vi "数据采集传输系统.vi"(8 "停止 2":bool) -> ()   [LabVIEW 2016]
uses:
  <vilib>/Averna/Notify Icon/NotifyIcon.llb/BalloonIcon.ctl
  <vilib>/Utility/miscctls.llb/LVPointTypeDef.ctl
  <vilib>/Utility/config.llb/Read Key (String).vi
  <vilib>/Utility/config.llb/Read Key (I32).vi
  <vilib>/Utility/config.llb/Read Key (Boolean).vi
  <vilib>/Utility/config.llb/Write Key (String).vi
  <vilib>/Utility/config.llb/Write Key (U32).vi
  <vilib>/Utility/config.llb/Write Key (I32).vi
  <vilib>/Utility/config.llb/Write Key (Boolean).vi
  <vilib>/Averna/Notify Icon/NotifyIcon.llb/GetSelectedItemEvent.vi
  <vilib>/Averna/Notify Icon/NotifyIcon.llb/SetVisible.vi
  <vilib>/Averna/Notify Icon/NotifyIcon.llb/SetMenuDefaultItem.vi
  <vilib>/Averna/Notify Icon/NotifyIcon.llb/SetTipText.vi
  <vilib>/Averna/Notify Icon/NotifyIcon.llb/NotifyIcon.lvclass
  <vilib>/Utility/config.llb/NI_LVConfig.lvlib
  data/FreeMem.dll
  <vilib>/ptbypt/NI_PtbyPt.lvlib
panel:
  in  "数据组合发送":bool
  in  "日志、参数发送":bool
  in  "2011发送":bool
  in  "判断数据反馈":bool
  in  "数据发送协议":enum16{"2005-212协议", "2017-212协议"}(ring)=enum."2017-212协议"
  in  "数据发送通道":enum16{"TCP", "VISA"}(ring)
  in  "baud rate":u32=9600 caption="波特率"
  in  "VISA resource name":refnum<visa-resource-name> caption="VISA资源名称"
  in  "查询质控数据起始时间":bool
  in  "返回主界面":bool
  out "零点核查索引起始时间":string
  out "跨度核查索引起始时间":string
  out "加标回收索引起始时间":string
  out "标样核查索引起始时间":string
  out "数据接收超时指示灯":bool
  in  "重发时间":T1(ring)
  in  "重发日期":T2(ring)
  in  "锁":bool
  in  "开机启动":bool
  in  "确定更改起始时间":bool
  in  "更改起始时间":bool
  in  "数据发送起始时间":timestamp format="%<%.3X\n%Y/%m/%d>T"
  in  "每周自动重发":bool=TRUE
  in  "确定":bool
  in  "返回":bool
  in  "PW":string
  in  "MN":string
  in  "PORT":string
  in  "IP":string
  in  "站点设备":string
  in  "站点名称":string
  out "设置超时时间/min":i32=1
  in  "实时数据发送时间间隔/min":u32=1
  out "空闲时间/s":string
  out "状态信息":T3={"1st Error to Convert "=63, "步骤 "=enum."打开连接", "元素"="实时数据", "TCP服务端掉线计数"=4, "TCP掉线时间节点"="2019/05/08 15:24:17"} {"1st Error to Convert" items=["无错误", "参数错误", "内存已满", "超出区域", "文件结束", "文件已打开", "一般文件IO错误", "未找到文件", "文件权限错误", "磁盘已满", "路径副本", "打开过多文件", "未启用", "未找到资源文件", "无法添加资源", "未找到资源", "未找到图像", "图像内存错误", "画笔不存在", "配置错误类型", "配置未找到解析段", "配置解析错误", "配置内存错误", "错误外部代码格式", "错误外部代码偏移量", "外部代码不存在", "空窗口", "销毁窗口错误", "空菜单", "打印已中止", "错误打印记录", "打印驱动程序错误", "打印时窗口错误", "打印时内存错误", "打印对话框错误", "一般打印错误", "无效设备引用句柄", "设备未找到", "设备参数错误", "设备单位错误", "无法打开设备", "设备调用已中止", "一般错误", "用户已取消", "对象ID过低", "对象ID过高", "对象不在堆中", "未知的堆", "错误DefProc ID", "DefProc不在表格中", "范围外信息", "空方法", "未知信息", "不支持管理器调用", "错误地址", "连接过程中", "连接超时", "连接过程中", "不支持网络属性", "网络错误", "正在使用的地址", "系统缺少内存", "连接已中止", "连接已拒绝", "连接未建立", "连接已建立", "连接已关闭", "初始化错误（交互应用程序管理器）", "错误事件发生", "等待无约束事件发生处理程序", "事件发生队列溢出", "错误路径", "未发出信号量", "未识别类型（交互应用程序管理器）"]}
  out "系统时间":string
  out "实时小时数据上传":bool
  out "系统状态改变":bool
  out "软件版本":string
  out "掉线指示":bool
  out "核查数据上传":bool
  out "通信状态":bool
  out "重发数据":bool
  out "配置信息":T4
  in  "参数配置":bool
  out "查询数据发送":bool
  out "读取报文显示":string
  out "发送报文显示":string
  out "心跳包":bool
  in  "参数数值":T5={"CODMn"=TRUE, "CODCr"=TRUE, "DO"=TRUE, "铜"=TRUE, "PH"=TRUE, "氨氮"=TRUE, "比电导率"=TRUE, "水温"=TRUE, "盐度(海水)"=TRUE, "浊度"=TRUE, "总氮"=TRUE, "总磷"=TRUE, "叶绿素a"=TRUE, "藻密度"=TRUE, "水位"=TRUE, "流速"=TRUE, "瞬时流量"=TRUE, "累积流量"=TRUE}
  in  "系统编码选择框":string(combo)="地表水质量监测"
  out "主队列输出":refnum<queue>
  in  "TCP掉线时间节点":string
  out "TCP服务端掉线计数":i32
  out "元素":string
  out "步骤":T6(ring)
  out "1st Error to Convert":i32(ring)=56 items=["无错误", "参数错误", "内存已满", "超出区域", "文件结束", "文件已打开", "一般文件IO错误", "未找到文件", "文件权限错误", "磁盘已满", "路径副本", "打开过多文件", "未启用", "未找到资源文件", "无法添加资源", "未找到资源", "未找到图像", "图像内存错误", "画笔不存在", "配置错误类型", "配置未找到解析段", "配置解析错误", "配置内存错误", "错误外部代码格式", "错误外部代码偏移量", "外部代码不存在", "空窗口", "销毁窗口错误", "空菜单", "打印已中止", "错误打印记录", "打印驱动程序错误", "打印时窗口错误", "打印时内存错误", "打印对话框错误", "一般打印错误", "无效设备引用句柄", "设备未找到", "设备参数错误", "设备单位错误", "无法打开设备", "设备调用已中止", "一般错误", "用户已取消", "对象ID过低", "对象ID过高", "对象不在堆中", "未知的堆", "错误DefProc ID", "DefProc不在表格中", "范围外信息", "空方法", "未知信息", "不支持管理器调用", "错误地址", "连接过程中", "连接超时", "连接过程中", "不支持网络属性", "网络错误", "正在使用的地址", "系统缺少内存", "连接已中止", "连接已拒绝", "连接未建立", "连接已建立", "连接已关闭", "初始化错误（交互应用程序管理器）", "错误事件发生", "等待无约束事件发生处理程序", "事件发生队列溢出", "错误路径", "未发出信号量", "未识别类型（交互应用程序管理器）"]
  out "QN":string
  out "时间QN":string
  out "系统编码ST":string
  out "命令编码CN":string
  out "密码PW":string
  out "设备编码MN":string
  out "拆分包及应答Flag":string
  out "数据":string
  in  "实时数据参数选择框":T7={"水样测量数据"=FALSE, "零点核查数据"=TRUE, "跨度核查数据"=TRUE, "加标回收数据"=TRUE, "平行样数据"=FALSE, "标样核查"=TRUE, "集成干预测试"=TRUE}
  out "数据输出":string
  in  "table元素":string
  out "数组":string[](array[string])
  out "数组 2":string[](array[string])
  out "空闲时间":dbl
  out "错误输出":errorcluster
  out "error out":errorcluster
  # "数 据 采 集 传 输 系 统"
  # "读取的参数区"
  # "水样测量数据"
  # "空白测试数据"
  # "跨度核查数据"
  # "加标回收数据"
  # "平行样数据"
  # "标样核查"
  # "集成干预测试"
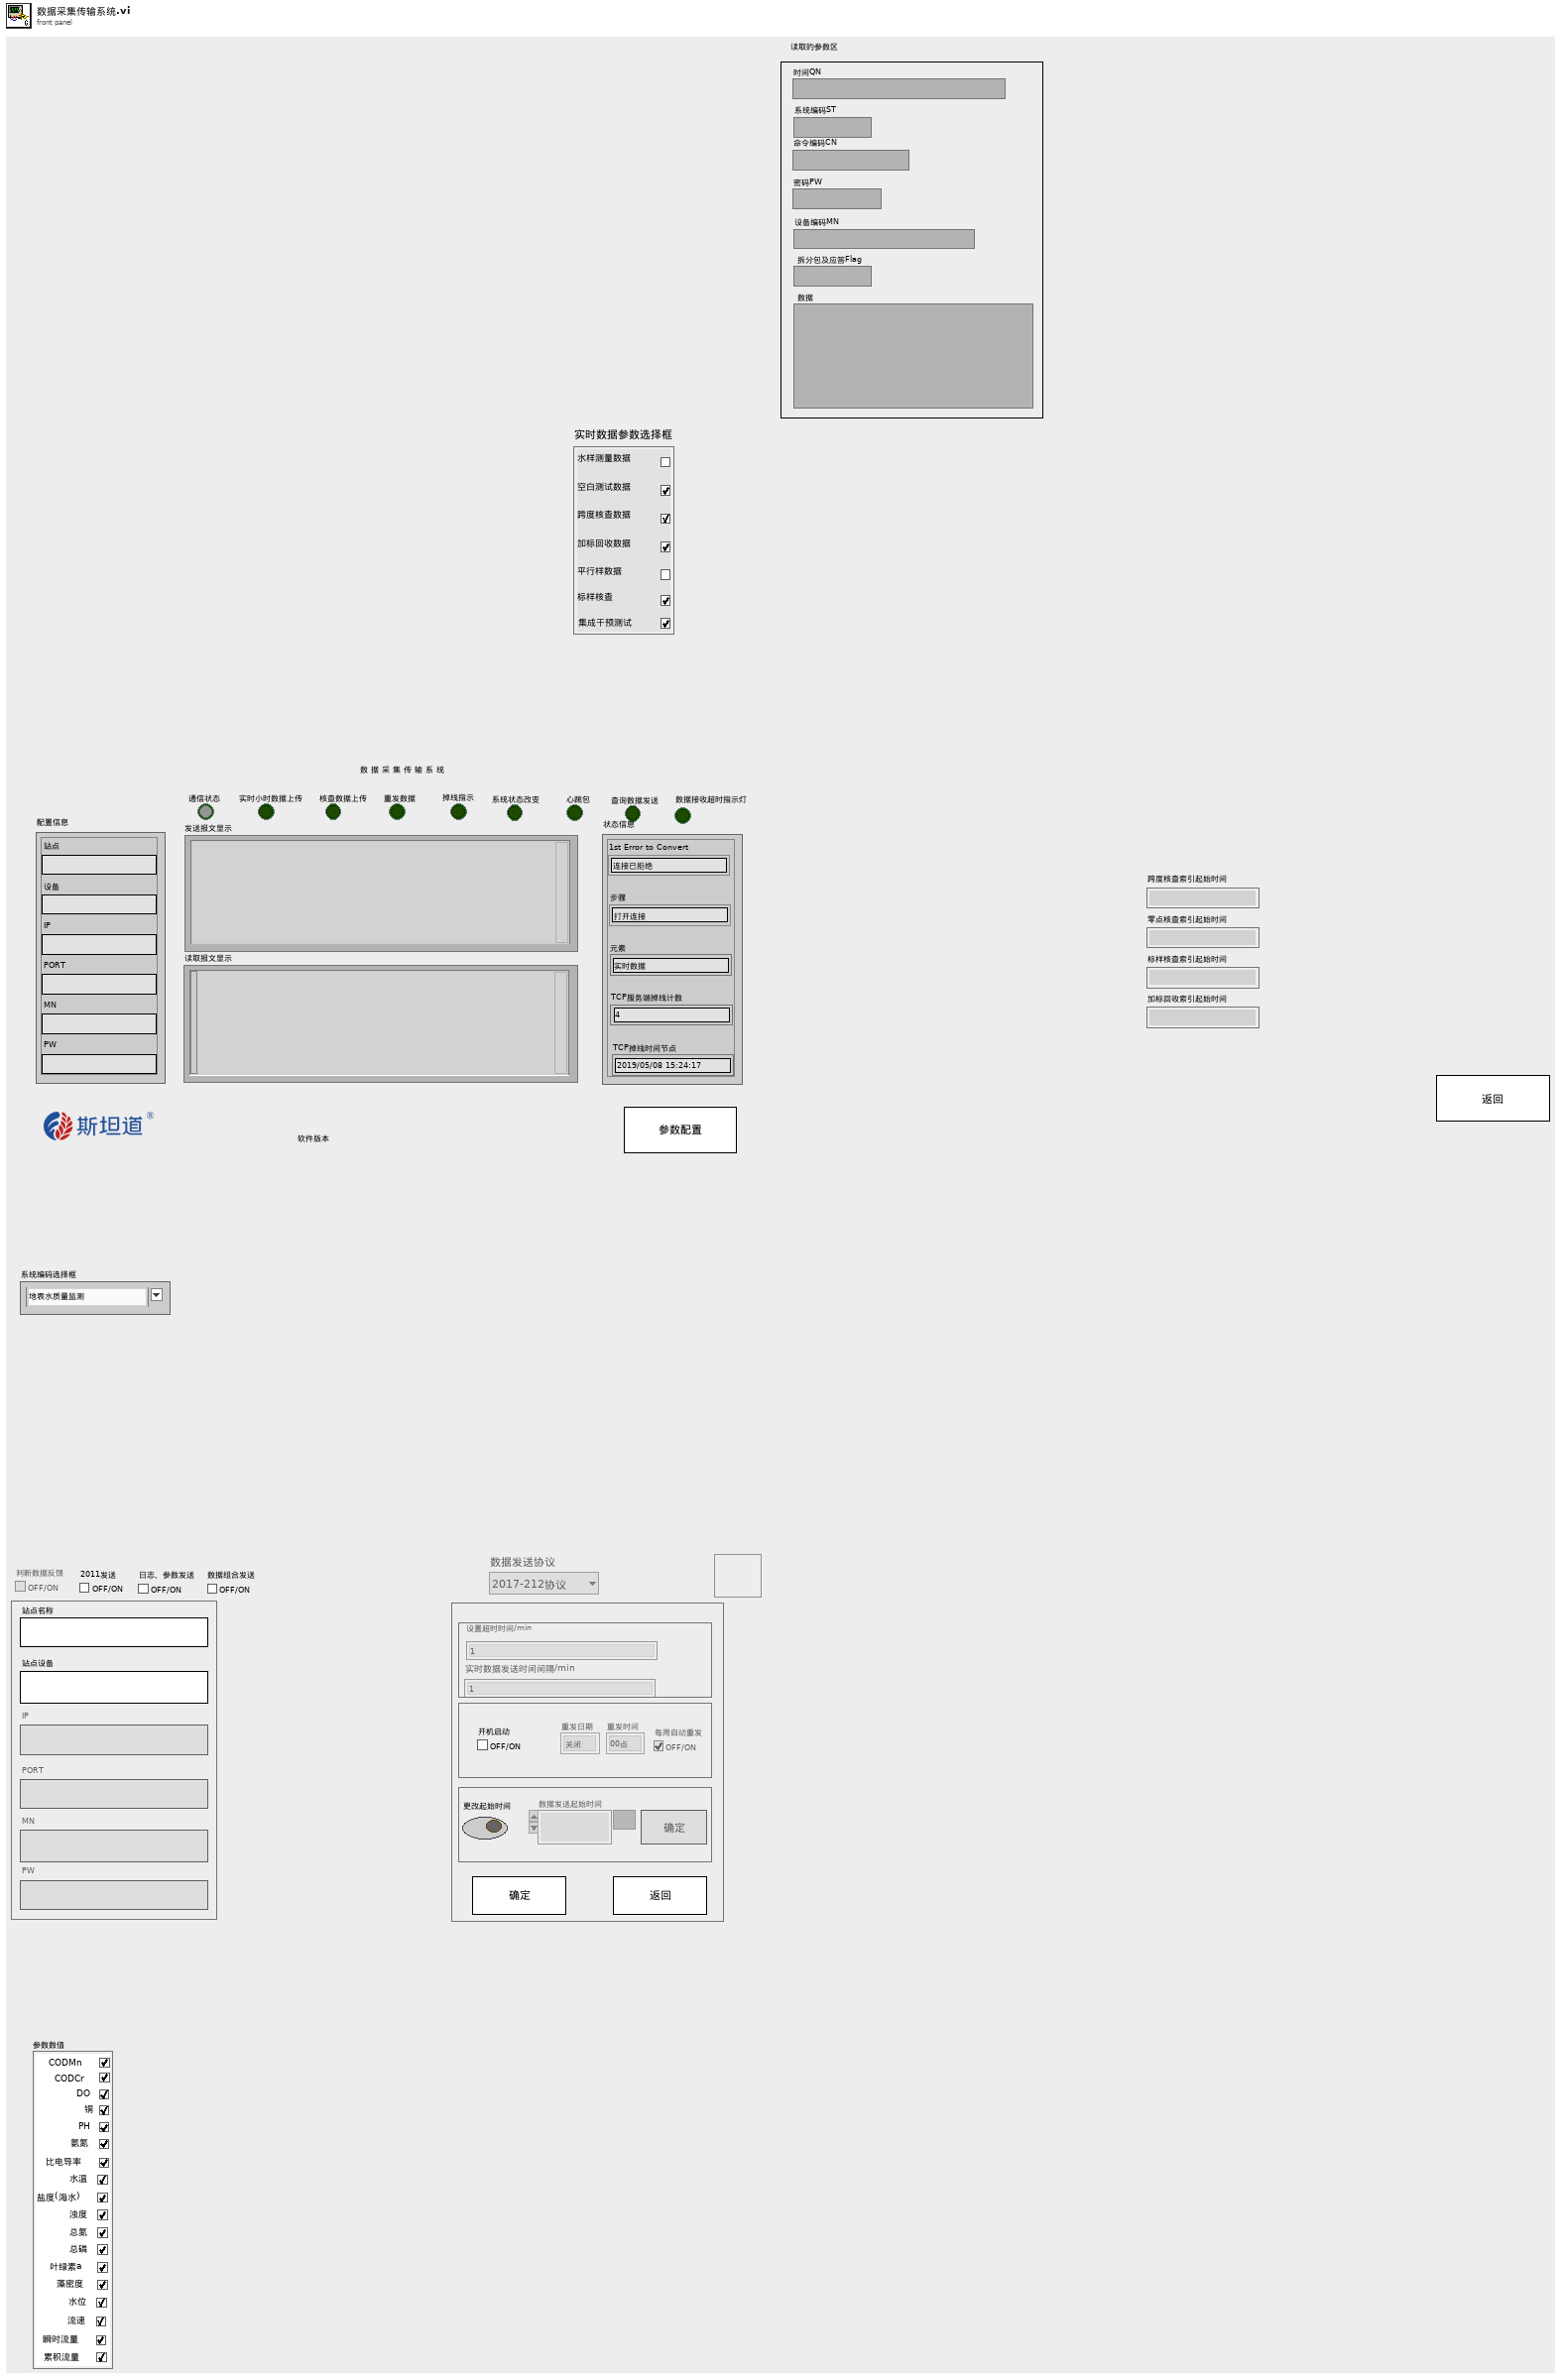
[diagram p1: front panel]
types:
  T1 = enum16{"00点", "01点", "02点", "03点", "04点", "05点", "06点", "07点", "08点", "09点", "10点", "11点", "12点", "13点", "14点", "15点", "16点", "17点", "18点", "19点", "20点", "21点", "22点", "23点"}
  T2 = enum16{"关闭", "星期日", "星期一", "星期二", "星期三", "星期四", "星期五", "星期六"}
  T3 = cluster{"1st Error to Convert ":i32, "步骤 ":enum16{"初始化", "打开连接", "表格比对", "发送数据", "读取数据", "数据处理"}, "元素":string, "TCP服务端掉线计数":i32, "TCP掉线时间节点":string}
  T4 = cluster{"站点":string, "设备":string, "IP":string, "PORT":string, "MN":string, "PW":string}
  T5 = cluster{"CODMn":bool, "CODCr":bool, "DO":bool, "铜":bool, "PH":bool, "氨氮":bool, "比电导率":bool, "水温":bool, "盐度(海水)":bool, "浊度":bool, "总氮":bool, "总磷":bool, "叶绿素a":bool, "藻密度":bool, "水位":bool, "流速":bool, "瞬时流量":bool, "累积流量":bool}
  T6 = enum16{"初始化", "打开连接", "表格比对", "发送数据", "读取数据", "数据处理"}
  T7 = cluster{"水样测量数据":bool, "零点核查数据":bool, "跨度核查数据":bool, "加标回收数据":bool, "平行样数据":bool, "标样核查":bool, "集成干预测试":bool}
  T8 = typedef "NI_LVConfig.lvlib/Config Data RefNum.ctl" = refnum<k1>
  T9 = typedef "LVDateTimeRec.ctl" = cluster{"秒数的小数部分":dbl, "秒":i32, "分":i32, "时":i32, "日":i32, "月":i32, "年":i32, "天数（周）":i32, "天数（年）":i32, "DST":i32}
  T10 = cluster{"PH":string[][], "CODCr":string[][], "氨氮":string[][], "CODMn":string[][], "总氮":string[][], "总磷":string[][], "电导率":string[][], "水温":string[][], "DO":string[][], "浊度":string[][], "叶绿素":string[][], "藻密度":string[][], "铜":string[][], "盐度":string[][], "水位":string[][], "流速":string[][], "瞬时流量":string[][], "累积流量":string[][]}
  T11 = typedef "LVPointTypeDef.ctl" = cluster{"Horizontal":i16, "Vertical":i16}
  T12 = enum8{"Enabled", "Disabled", "Disabled and Grayed Out"}
  T13 = typedef "imagedata.ctl" = cluster{"image type":i32, "image depth":i32, "image":u8[], "mask":u8[], "colors":u32[], "Rectangle":cluster{"left":i16, "top":i16, "right":i16, "bottom":i16}}
  T14 = enum32{"invalid app kind", "Development System", "Run Time System", "Student Edition", "Embedded LabVIEW", "Evaluation", "Custom"}
  T15 = enum32{"Invalid", "Standard", "Closed", "Hidden", "Minimized", "Maximized"}
  T16 = enum16{"水样测试", "小时数据", "日志信息", "报警信息", "零点核查", "标样核查", "平行样", "加标回收"}
  T17 = enum16{"CODMn", "CODCr", "氨氮", "总磷", "总氮", "数采仪"}
  T18 = cluster{"高锰酸盐":string, "化学需氧量":string, "氨氮":string, "总磷":string, "总氮":string, "数采仪":string, "高锰酸盐":bool, "化学需氧量":bool, "氨氮":bool, "总磷":bool, "总氮":bool, "数采仪":bool}
  T19 = typedef "NotifyIcon.lvlib/NotifyIcon.lvclass/BalloonIcon.ctl" = enum32{"None", "Information", "Warning", "Error"}
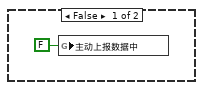
[diagram p3: hidden frame]
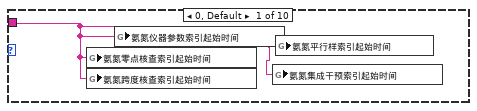
[diagram p7: hidden frame]
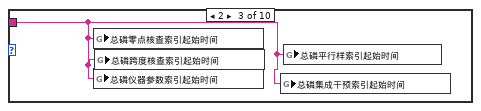
[diagram p8: hidden frame]
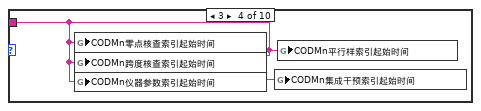
[diagram p9: hidden frame]
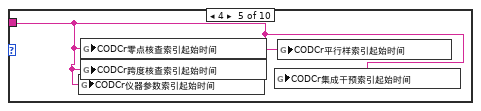
[diagram p10: hidden frame]
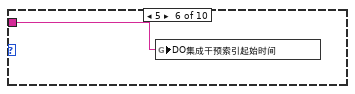
[diagram p11: hidden frame]
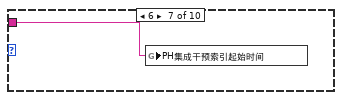
[diagram p12: hidden frame]
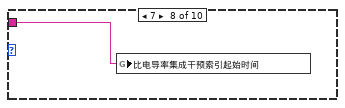
[diagram p13: hidden frame]
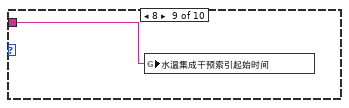
[diagram p14: hidden frame]
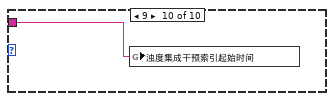
[diagram p15: hidden frame]
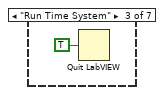
[diagram p17: hidden frame]
diagram:
  w23 = string[] ["OPEN线程一", "APP_SEPARATOR", "EXIT线程一"]
  (unwired) string[] ["CODMn", "CODCr", "DO", "DOper", "PH", "氨氮", "电导率", "水温", "盐度", "浊度", "总氮", "总磷", "叶绿素a", "藻密度", "水位", "流速", "瞬时流量", "累积流量"] ("查询参数数组")
  (unwired) 0 items=["无错误", "参数错误", "内存已满", "超出区域", "文件结束", "文件已打开", "一般文件IO错误", "未找到文件", "文件权限错误", "磁盘已满", "路径副本", "打开过多文件", "未启用", "未找到资源文件", "无法添加资源", "未找到资源", "未找到图像", "图像内存错误", "画笔不存在", "配置错误类型", "配置未找到解析段", "配置解析错误", "配置内存错误", "错误外部代码格式", "错误外部代码偏移量", "外部代码不存在", "空窗口", "销毁窗口错误", "空菜单", "打印已中止", "错误打印记录", "打印驱动程序错误", "打印时窗口错误", "打印时内存错误", "打印对话框错误", "一般打印错误", "无效设备引用句柄", "设备未找到", "设备参数错误", "设备单位错误", "无法打开设备", "设备调用已中止", "一般错误", "用户已取消", "对象ID过低", "对象ID过高", "对象不在堆中", "未知的堆", "错误DefProc ID", "DefProc不在表格中", "范围外信息", "空方法", "未知信息", "不支持管理器调用", "错误地址", "连接过程中", "连接超时", "连接过程中", "不支持网络属性", "网络错误", "正在使用的地址", "系统缺少内存", "连接已中止", "连接已拒绝", "连接未建立", "连接已建立", "连接已关闭", "初始化错误（交互应用程序管理器）", "错误事件发生", "等待无约束事件发生处理程序", "事件发生队列溢出", "错误路径", "未发出信号量", "未识别类型（交互应用程序管理器）"] ("1st Error to Convert")
  # "6."
  # "3."
  # "1."
  # "判定当数据没有传送完毕并掉线，将数据存储入临时表格"
  # "上传本地时间点的实时数据"
  # "目前时间太短，如果掉线了，数据存不了临时表格"
  # "获取需要发送的数据表"
  n1 = Cluster To Array(cluster="参数数值") -> (array=w33:bool[])
  n2 = for {
    tunnel: w33 -> [_] mode=indexing
    tunnel: [w73] -> w32
    i -> [w73]
    w62 = "线程一数据重发功能" ("section")
    # "初始化水样搜索起始时间"
    n3 = case shown="3" w73 {
      tunnel: [w104 w106 w108 w110 w112 w114 w116 w118 w120 w122 w124 w126 w128 w130 w132 w134 w136 w138] -> w77
      frame 0, Default {
        n4 = control-ref of="CODMn"() -> (w105:refnum<vi>)
        n5 = property class="Bool (严格)"(reference=w105) -> ("Label.Text"=w104:string)  [unwired: 1 in, 2 out]
      }
      frame 1 {
        n6 = control-ref of="CODCr"() -> (w107:refnum<vi>)
        n7 = property class="Bool (严格)"(reference=w107) -> ("Label.Text"=w106:string)  [unwired: 1 in, 2 out]
      }
      frame 2 {
        n8 = control-ref of="DO"() -> (w109:refnum<vi>)
        n9 = property class="Bool (严格)"(reference=w109) -> ("Label.Text"=w108:string)  [unwired: 1 in, 2 out]
      }
      frame 3 {
        n10 = control-ref of="铜"() -> (w111:refnum<vi>)
        n11 = property class="Bool (严格)"(reference=w111) -> ("Label.Text"=w110:string)  [unwired: 1 in, 2 out]
      }
      frame 4 {
        n12 = control-ref of="PH"() -> (w113:refnum<vi>)
        n13 = property class="Bool (严格)"(reference=w113) -> ("Label.Text"=w112:string)  [unwired: 1 in, 2 out]
      }
      frame 5 {
        n14 = control-ref of="氨氮"() -> (w115:refnum<vi>)
        n15 = property class="Bool (严格)"(reference=w115) -> ("Label.Text"=w114:string)  [unwired: 1 in, 2 out]
      }
      frame 6 {
        n16 = control-ref of="比电导率"() -> (w117:refnum<vi>)
        n17 = property class="Bool (严格)"(reference=w117) -> ("Label.Text"=w116:string)  [unwired: 1 in, 2 out]
      }
      frame 7 {
        n18 = control-ref of="水温"() -> (w119:refnum<vi>)
        n19 = property class="Bool (严格)"(reference=w119) -> ("Label.Text"=w118:string)  [unwired: 1 in, 2 out]
      }
      frame 8 {
        n20 = control-ref of="盐度(海水)"() -> (w121:refnum<vi>)
        n21 = property class="Bool (严格)"(reference=w121) -> ("Label.Text"=w120:string)  [unwired: 1 in, 2 out]
      }
      frame 9 {
        n22 = control-ref of="浊度"() -> (w123:refnum<vi>)
        n23 = property class="Bool (严格)"(reference=w123) -> ("Label.Text"=w122:string)  [unwired: 1 in, 2 out]
      }
      frame 10 {
        n24 = control-ref of="总氮"() -> (w125:refnum<vi>)
        n25 = property class="Bool (严格)"(reference=w125) -> ("Label.Text"=w124:string)  [unwired: 1 in, 2 out]
      }
      frame 11 {
        n26 = control-ref of="总磷"() -> (w127:refnum<vi>)
        n27 = property class="Bool (严格)"(reference=w127) -> ("Label.Text"=w126:string)  [unwired: 1 in, 2 out]
      }
      frame 12 {
        n28 = control-ref of="叶绿素a"() -> (w129:refnum<vi>)
        n29 = property class="Bool (严格)"(reference=w129) -> ("Label.Text"=w128:string)  [unwired: 1 in, 2 out]
      }
      frame 13 {
        n30 = control-ref of="藻密度"() -> (w131:refnum<vi>)
        n31 = property class="Bool (严格)"(reference=w131) -> ("Label.Text"=w130:string)  [unwired: 1 in, 2 out]
      }
      frame 14 {
        n32 = control-ref of="水位"() -> (w133:refnum<vi>)
        n33 = property class="Bool (严格)"(reference=w133) -> ("Label.Text"=w132:string)  [unwired: 1 in, 2 out]
      }
      frame 15 {
        n34 = control-ref of="流速"() -> (w135:refnum<vi>)
        n35 = property class="Bool (严格)"(reference=w135) -> ("Label.Text"=w134:string)  [unwired: 1 in, 2 out]
      }
      frame 16 {
        n36 = control-ref of="瞬时流量"() -> (w137:refnum<vi>)
        n37 = property class="Bool (严格)"(reference=w137) -> ("Label.Text"=w136:string)  [unwired: 1 in, 2 out]
      }
      frame 17 {
        n38 = control-ref of="累积流量"() -> (w139:refnum<vi>)
        n39 = property class="Bool (严格)"(reference=w139) -> ("Label.Text"=w138:string)  [unwired: 1 in, 2 out]
      }
    }
    n40 = call <vilib>:"Application Directory.vi"() -> ("Application Directory"=w83:path)
    n41 = Build Path(base path=w83, name or relative path="data\\Set.ini" ("名称或相对路径")) -> (appended path=w81:path)
    n42 = call <vilib>:"Open Config Data.vi"("configuration file path"=w81) -> ("error out"=w79:errorcluster, "refnum"=w80:T8)  [unwired: 8 in, 1 out]
    n43 = call-poly <vilib>:"Read Key.vi"("section"="线程一数据搜索起始时间", "error in (no error)"=w79, "key"=w77, "refnum"=w80) -> ("error out"=w71:errorcluster, "value"=w74:string, "refnum out"=w72:T8)  [unwired: 4 in, 1 out]
    n44 = Empty String/Path?(string/path=w74) -> (empty?=w76:bool)
    n45 = case shown="真" w76 {
      tunnel: [w84 "1904/01/01 00:00:00"] -> w75
      tunnel: w74 -> [w84 _]
      frame False {
      }
      frame True {
      }
    }
    n46 = call-poly <vilib>:"Read Key.vi"("section"=w62, "error in (no error)"=w71, "key"="重发功能", "refnum"=w72) -> ("error out"=w65:errorcluster, "value"=w69:bool, "refnum out"=w66:T8)  [unwired: 4 in, 1 out]
    n47 = local write "每周自动重发"(w69) -> ()
    n48 = call-poly <vilib>:"Read Key.vi"("section"=w62, "error in (no error)"=w65, "key"="重发日期", "refnum"=w66) -> ("error out"=w63:errorcluster, "value"=w59:i32, "refnum out"=w64:T8)  [unwired: 4 in, 1 out]
    n49 = local write "重发日期"(w59) -> ()
    n50 = case shown="3" w73 {
      tunnel: w75 -> [w86 w87 w88 w89 w90 w91 w92 w93 w94 w95 w96 w97 w98 w99 w100 w101 w102 w103]
      frame 0, Default {
        n51 = global write "全局 水样时间.vi" "time1"(w86) -> ()
      }
      frame 1 {
        n52 = global write "全局 水样时间.vi" "time2"(w87) -> ()
      }
      frame 2 {
        n53 = global write "全局 水样时间.vi" "time3"(w88) -> ()
      }
      frame 3 {
        n54 = global write "全局 水样时间.vi" "time4"(w89) -> ()
      }
      frame 4 {
        n55 = global write "全局 水样时间.vi" "time5"(w90) -> ()
      }
      frame 5 {
        n56 = global write "全局 水样时间.vi" "time6"(w91) -> ()
      }
      frame 6 {
        n57 = global write "全局 水样时间.vi" "time7"(w92) -> ()
      }
      frame 7 {
        n58 = global write "全局 水样时间.vi" "time8"(w93) -> ()
      }
      frame 8 {
        n59 = global write "全局 水样时间.vi" "time9"(w94) -> ()
      }
      frame 9 {
        n60 = global write "全局 水样时间.vi" "time10"(w95) -> ()
      }
      frame 10 {
        n61 = global write "全局 水样时间.vi" "time11"(w96) -> ()
      }
      frame 11 {
        n62 = global write "全局 水样时间.vi" "time12"(w97) -> ()
      }
      frame 12 {
        n63 = global write "全局 水样时间.vi" "time13"(w98) -> ()
      }
      frame 13 {
        n64 = global write "全局 水样时间.vi" "time14"(w99) -> ()
      }
      frame 14 {
        n65 = global write "全局 水样时间.vi" "time15"(w100) -> ()
      }
      frame 15 {
        n66 = global write "全局 水样时间.vi" "time16"(w101) -> ()
      }
      frame 16 {
        n67 = global write "全局 水样时间.vi" "time17"(w102) -> ()
      }
      frame 17 {
        n68 = global write "全局 水样时间.vi" "time18"(w103) -> ()
      }
    }
    n69 = call-poly <vilib>:"Read Key.vi"("section"=w62, "error in (no error)"=w63, "key"="重发时间", "refnum"=w64) -> ("error out"=w60:errorcluster, "value"=w58:i32, "refnum out"=w61:T8)  [unwired: 4 in, 1 out]
    n70 = local write "重发时间"(w58) -> ()
    n71 = call <vilib>:"Close Config Data.vi"("error in (no error)"=w60, "refnum"=w61) -> ()  [unwired: 8 in, 2 out]
  }
  n72 = Obtain Queue(name (unnamed)="数据发送" ("名称（未命名）"), element data type="") -> (queue out=w38:refnum<queue>, error out=w37:errorcluster)  [unwired: 3 in, 1 out]
  n73 = Obtain Queue(name (unnamed)="实时数据参数选择" ("名称（未命名）"), element data type="") -> (queue out=w39:refnum<queue>, error out=w36:errorcluster)  [unwired: 3 in, 1 out]
  n74 = while {
    tunnel: w38 -> [w155]
    stop <- FALSE stop-if-true
    # "核查和质控数据的定期发送在实时数据周期上传"
    # "指定周期发一次核查数据，仪器参数日志"
    n75 = local read "核查数据上传"() -> (w141:bool)
    n76 = local read "查询数据发送"() -> (w150:bool)
    n77 = local read "实时小时数据上传"() -> (w154:bool)
    n78 = local read "重发数据"() -> (w151:bool)
    n79 = Multiply(x="实时数据发送时间间隔/min", y=u32 60000 ("等待时间（毫秒）")) -> (x*y=w158:u32)
    n80 = local read "步骤"() -> (w149:T6)
    n81 = Not(x=w141) -> (.not. x?=w140:bool)
    n82 = Not(x=w150) -> (.not. x?=w146:bool)
    n83 = Wait (ms)(milliseconds to wait=w158) -> ()  [unwired: 1 out]
    n84 = Not(x=w151) -> (.not. x?=w145:bool)
    n85 = Not(x=w154) -> (.not. x?=w152:bool)
    n86 = First Call?() -> (First Call?: T/F=w156:bool)
    n87 = Equal?(x=w149, y=T6."读取数据" ("步骤")) -> (x = y?=w147:bool)
    n88 = case shown="真" w156 {
      tunnel: w155 -> [_ _]
      frame False {
      }
      frame True {
        (unwired) "1994/01/01 00:00:00"
        # "上传最近一年的质控数据"
        n89 = Get Date/Time In Seconds() -> (seconds since 1Jan1904=w193:timestamp)
        n90 = Seconds To Date/Time(time stamp (now)=w193) -> (date time rec=w192:T9)  [unwired: 1 in]
        n91 = Unbundle By Name(w192) -> ("年"=w177:i32)
        n92 = Bundle By Name(cluster=w192, "年"=w177) -> (w190:T9)
        n93 = Date/Time To Seconds(2:w190) -> (0:w191:timestamp)  [unwired: 1 in]
        n94 = Format Date/Time String(time format string (%c)="%Y/%m/%d %H:%M:%S" ("时间格式字符串(%c)"), seconds (now)=w191) -> (date/time string=w188:string)  [unwired: 1 in]
        n95 = global write "全局 时间2.vi" "跨度核查索引起始时间"(w188) -> ()
        n96 = global write "全局 时间2.vi" "零点核查索引起始时间"(w188) -> ()
        n97 = global write "全局 时间2.vi" "平行样索引起始时间"(w188) -> ()
        n98 = global write "全局 时间2.vi" "加标回收索引起始时间"(w188) -> ()
        n99 = global write "全局 时间2.vi" "标样核查索引起始时间"(w188) -> ()
        n100 = call <vilib>:"Application Directory.vi"() -> ("Application Directory"=w185:path)
        n101 = Build Path(base path=w185, name or relative path="data\\hecha.ini" ("名称或相对路径")) -> (appended path=w187:path)
        n102 = call <vilib>:"Open Config Data.vi"("configuration file path"=w187) -> ("error out"=w181:errorcluster, "refnum"=w182:T8)  [unwired: 8 in, 1 out]
        n103 = vi-ref "全局 时间2.vi"() -> (w183:refnum<vi>)
        n104 = call <userlib>:"Read Panel from INI__ogtk.vi"("error in (no error)"=w181, "VI ref"=w183, "refnum"=w182) -> ("error out"=w180:errorcluster, "refnum out"=w184:T8)  [unwired: 7 in]
        n105 = call <vilib>:"Close Config Data.vi"("error in (no error)"=w180, "refnum"=w184) -> ("error out"=w179:errorcluster)  [unwired: 8 in, 1 out]
        n106 = for {
          N: 10 -> [_]
          tunnel: w188 -> [w194]
          tunnel: w179 -> [_]
          i -> [w195]
          n107 = case shown="1" w195 {
            tunnel: w194 -> [w196 w197 w198 w199 w200 w201 w202 w203 w204 w205]
            frame 0, Default {
              n108 = global write "全局 时间2.vi" "氨氮零点核查索引起始时间"(w196) -> ()
              n109 = global write "全局 时间2.vi" "氨氮跨度核查索引起始时间"(w196) -> ()
              n110 = global write "全局 时间2.vi" "氨氮仪器参数索引起始时间"(w196) -> ()
              n111 = global write "全局 时间2.vi" "氨氮集成干预索引起始时间"(w196) -> ()
              n112 = global write "全局 时间2.vi" "氨氮平行样索引起始时间"(w196) -> ()
            }
            frame 1 {
              n113 = global write "全局 时间2.vi" "总氮仪器参数索引起始时间"(w197) -> ()
              n114 = global write "全局 时间2.vi" "总氮跨度核查索引起始时间"(w197) -> ()
              n115 = global write "全局 时间2.vi" "总氮零点核查索引起始时间"(w197) -> ()
              n116 = global write "全局 时间2.vi" "总氮集成干预索引起始时间"(w197) -> ()
              n117 = global write "全局 时间2.vi" "总氮平行样索引起始时间"(w197) -> ()
            }
            frame 2 {
              n118 = global write "全局 时间2.vi" "总磷零点核查索引起始时间"(w198) -> ()
              n119 = global write "全局 时间2.vi" "总磷仪器参数索引起始时间"(w198) -> ()
              n120 = global write "全局 时间2.vi" "总磷跨度核查索引起始时间"(w198) -> ()
              n121 = global write "全局 时间2.vi" "总磷集成干预索引起始时间"(w198) -> ()
              n122 = global write "全局 时间2.vi" "总磷平行样索引起始时间"(w198) -> ()
            }
            frame 3 {
              n123 = global write "全局 时间2.vi" "CODMn零点核查索引起始时间"(w199) -> ()
              n124 = global write "全局 时间2.vi" "CODMn跨度核查索引起始时间"(w199) -> ()
              n125 = global write "全局 时间2.vi" "CODMn仪器参数索引起始时间"(w199) -> ()
              n126 = global write "全局 时间2.vi" "CODMn集成干预索引起始时间"(w199) -> ()
              n127 = global write "全局 时间2.vi" "CODMn平行样索引起始时间"(w199) -> ()
            }
            frame 4 {
              n128 = global write "全局 时间2.vi" "CODCr仪器参数索引起始时间"(w200) -> ()
              n129 = global write "全局 时间2.vi" "CODCr零点核查索引起始时间"(w200) -> ()
              n130 = global write "全局 时间2.vi" "CODCr跨度核查索引起始时间"(w200) -> ()
              n131 = global write "全局 时间2.vi" "CODCr集成干预索引起始时间"(w200) -> ()
              n132 = global write "全局 时间2.vi" "CODCr平行样索引起始时间"(w200) -> ()
            }
            frame 5 {
              n133 = global write "全局 时间2.vi" "DO集成干预索引起始时间"(w201) -> ()
            }
            frame 6 {
              n134 = global write "全局 时间2.vi" "PH集成干预索引起始时间"(w202) -> ()
            }
            frame 7 {
              n135 = global write "全局 时间2.vi" "比电导率集成干预索引起始时间"(w203) -> ()
            }
            frame 8 {
              n136 = global write "全局 时间2.vi" "水温集成干预索引起始时间"(w204) -> ()
            }
            frame 9 {
              n137 = global write "全局 时间2.vi" "浊度集成干预索引起始时间"(w205) -> ()
            }
          }
        }
      }
    }
    n138 = local read "数据发送协议"() -> (w144:enum16{"2005-212协议", "2017-212协议"})
    n139 = Equal?(x=w144, y=enum16{"2005-212协议", "2017-212协议"}."2017-212协议" ("数据发送协议")) -> (x = y?=w142:bool)
    n140 = Compound Arithmetic op=AND ("复合运算")(w140, w142, w145, w146, w147, w152) -> (w153:bool)
    n141 = case shown="真" w153 {
      tunnel: w155 -> [_ w165]
      frame False {
      }
      frame True {
        n142 = call "实时数据参数入列队.vi"("实时数据参数选择框"="实时数据参数选择框") -> ("错误输出"=w167:errorcluster)  [unwired: 10 in]
        n143 = local read "日志、参数发送"() -> (w161:bool)
        n144 = call <vilib>:"Clear Errors.vi"("error in (no error)"=w167) -> ()  [unwired: 5 in, 2 out]
        n145 = Enqueue Element(queue=w165, element="send" ("元素")) -> (queue out=w164:refnum<queue>, error out=w163:errorcluster)  [unwired: 2 in, 1 out]
        n146 = case shown="真" w161 {
          tunnel: w164 -> [_ w174]
          tunnel: w163 -> [_ w173]
          frame False {
          }
          frame True {
            n147 = Enqueue Element(queue=w174, element="操作日志" ("元素"), error in (no error)=w173) -> (queue out=w171:refnum<queue>, error out=w170:errorcluster)  [unwired: 1 in, 1 out]
            n148 = Enqueue Element(queue=w171, element="仪器参数" ("元素"), error in (no error)=w170) -> (queue out=w169:refnum<queue>, error out=w168:errorcluster)  [unwired: 1 in, 1 out]
            n149 = Enqueue Element(queue=w169, element="报警信息" ("元素"), error in (no error)=w168) -> ()  [unwired: 1 in, 3 out]
          }
        }
      }
    }
  }
  n150 = while "While循环" {
    tunnel: w38 -> [w218]
    tunnel: w39 -> [w222]
    tunnel: w37 -> [w221]
    tunnel: w36 -> [w220]
    stop <- FALSE stop-if-true
    # "判定数据发送时要发送实时数据"
    # "所有的主动上传数据都是有数据才会上传"
    n151 = Get Queue Status(queue=w218) -> (# elements in queue=w210:i32)  [unwired: 2 in, 7 out]
    n152 = local read "查询数据发送"() -> (w216:bool)
    n153 = global read "全局 数据发送重叠.vi" "主动上报数据中"() -> (w208:bool)
    n154 = local read "重发数据"() -> (w207:bool)
    n155 = Not Equal To 0?(x=w210) -> (x != 0?=w217:bool)
    n156 = And(x=w217, y=w216) -> (x .and. y?=w209:bool)
    n157 = call <vilib>:"Boolean Crossing PtByPt.vi"("direction"=enum16{"either", "false-true", "true-false"}."false-true", "input"=w209) -> ("crossing"=w215:bool)  [unwired: 1 in]
    n158 = Not(x=w208) -> (.not. x?=w212:bool)
    n159 = Not(x=w207) -> (.not. x?=w206:bool)
    n160 = Not(x=w216) -> (.not. x?=w213:bool)
    n161 = case shown="真" w215 {
      frame False {
      }
      frame True {
        n162 = Get Date/Time In Seconds() -> (seconds since 1Jan1904=w228:timestamp)
        n163 = Seconds To Date/Time(time stamp (now)=w228) -> (date time rec=w225:T9)  [unwired: 1 in]
        n164 = Date/Time To Seconds(2:w225) -> (0:w227:timestamp)  [unwired: 1 in]
        n165 = Format Date/Time String(time format string (%c)="%Y/%m/%d %H:%M:%S" ("时间格式字符串(%c)"), seconds (now)=w227) -> (date/time string=w224:string)  [unwired: 1 in]
        n166 = global write "全局 数据发送重叠.vi" "数据发送重叠开始时间戳"(w224) -> ()
      }
    }
    n167 = Compound Arithmetic op=AND ("复合运算")(w213, w212, w206) -> (w211:bool)
    n168 = Wait (ms)(milliseconds to wait=u32 1000 ("等待时间（毫秒）")) -> ()  [unwired: 1 out]
    n169 = case shown="真" w211 {
      tunnel: w218 -> [_ w238]
      tunnel: w222 -> [_ w237]
      tunnel: w221 -> [_ w236]
      tunnel: w220 -> [_ w235]
      tunnel: w210 -> [_ w231]
      tunnel: w209 -> [_ w230]
      frame False {
        n170 = local write "核查数据上传"(FALSE ("数据上传")) -> ()
      }
      frame True {
        n171 = Equal To 0?(x=w231) -> (x = 0?=w232:bool)
        n172 = global write "全局 数据发送重叠.vi" "数据发送重叠"(w230) -> ()
        n173 = Not(x=w232) -> (.not. x?=w233:bool)
        n174 = local write "核查数据上传"(w233) -> ()
        n175 = Dequeue Element(queue=w238, error in (no error)=w236) -> (element=w234:string)  [unwired: 1 in, 3 out]
        n176 = case shown="\"仪器参数\"" w234 {
          tunnel: w237 -> [_ w240 _ _ _ _ _ _ _ _ _]
          tunnel: w235 -> [_ w239 _ _ _ _ _ _ _ _ _]
          frame "假", Default {
          }
          frame "send" {
            # "间隔时间上传"
            n177 = while {
              tunnel: w240 -> [w244]
              tunnel: w239 -> [w241]
              stop <- w245 stop-if-true
              n178 = Dequeue Element(queue=w244, error in (no error)=w241) -> (queue out=w243:refnum<queue>, element=w246:string)  [unwired: 1 in, 2 out]
              n179 = case shown="\"跨度核查\"" w246 {
                tunnel: [_ _ _ w412 _ _ _ w619] -> w245
                tunnel: w243 -> [_ _ _ _ _ _ _ w622]
                frame "水样测试" {
                  n180 = flat-sequence {
                    frame #0 {
                      n181 = global write "全局 小时数据发送次数.vi" "小时数据发送次数"(0 ("小时数据发送次数")) -> ()
                      n182 = global write "全局 实时数据参数.vi" "实时数据参数"("水样测试") -> ()
                      n183 = global write "全局1.vi" "枚举"(enum16{"返回请求应答", "上传数据", "返回执行结果"}."上传数据" ("枚举")) -> ()
                    }
                    frame #1 {
                      n184 = call "从数据库获取数据通用可配置(子VI).vi"("table输入"="实时数据" ("新元素/子数组"), "列队名（唯一）"="a") -> ()  [unwired: 8 in, 2 out]
                    }
                    frame #2 {
                      n185 = call "实时小时数据处理整合 (子VI).vi"("枚举"=enum16{"实时数据排序", "小时数据排序"}."实时数据排序") -> ("已排序的数组"=w253:string[])  [unwired: 10 in]
                      n186 = Array Size(array=w253) -> (size(s)=w254:i32)
                      n187 = global write "全局 数据数组大小.vi" "数据数组大小"(w254) -> ()
                    }
                    frame #3 {
                      n188 = while {
                        stop <- w259 stop-if-true
                        n189 = property on="TCP服务端掉线计数" class="DigNum (严格)"() -> ("Value"=w262:i32)  [unwired: 2 in, 2 out]
                        n190 = Greater Or Equal?(x=w262, y=1) -> (x >= y?=w261:bool)
                        n191 = case shown="假" w261 {
                          frame False {
                            n192 = global read "全局 数据数组大小.vi" "数据数组大小"() -> (w264:i32)
                            n193 = Greater Than 0?(x=w264) -> (x > 0?=w265:bool)
                            n194 = case shown="真" w265 {
                              frame False {
                              }
                              frame True {
                                n195 = local read "MN"() -> (w271:string)
                                n196 = local read "PW"() -> (w270:string)
                                n197 = local read "数据发送通道"() -> (w269:enum16{"TCP", "VISA"})
                                n198 = call "数据编码.vi"("table输入"="实时数据" ("新元素/子数组"), "MN"=w271, "PW"=w270) -> ("通讯包字符串"=w266:string)  [unwired: 11 in, 1 out]
                                n199 = local write "发送报文显示"(w266) -> ()
                                n200 = call "VISATCP组合选择发送.vi"("数据发送通道"=w269, "命令"="write", "写入缓冲区"=w266) -> ("错误输出"=→"错误输出":errorcluster)  [unwired: 9 in, 3 out]
                                n201 = Build Array(w266) -> (w273:string[])
                                n202 = call "发送数据记录到文档(子VI).vi"("数组"=w273) -> ()  [unwired: 9 in, 1 out]
                                "核查数据上传" <- TRUE ("主动数据上传")
                              }
                            }
                          }
                          frame True {
                          }
                        }
                        n203 = Wait (ms)(milliseconds to wait=u32 500 ("等待时间（毫秒）")) -> ()  [unwired: 1 out]
                        n204 = global read "全局 数据数组大小.vi" "数据数组大小"() -> (w256:i32)
                        n205 = global read "全局 小时数据发送次数.vi" "小时数据发送次数"() -> (w260:i32)
                        n206 = Decrement(x=w256) -> (x-1=w255:i32)
                        n207 = Greater Or Equal?(x=w260, y=w255) -> (x >= y?=w258:bool)
                        n208 = Compound Arithmetic op=OR ("复合运算")(w258) -> (w259:bool)
                      }
                    }
                  }
                }
                frame "空白测试" {
                  n209 = flat-sequence {
                    frame #0 {
                      n210 = global write "全局 小时数据发送次数.vi" "小时数据发送次数"(0 ("小时数据发送次数")) -> ()
                      n211 = global write "全局 实时数据参数.vi" "实时数据参数"("空白测试") -> ()
                      n212 = global write "全局1.vi" "枚举"(enum16{"返回请求应答", "上传数据", "返回执行结果"}."上传数据" ("枚举")) -> ()
                    }
                    frame #1 {
                      n213 = call "从数据库获取数据通用可配置(子VI).vi"("table输入"="实时数据" ("新元素/子数组"), "列队名（唯一）"="b") -> ()  [unwired: 8 in, 2 out]
                    }
                    frame #2 {
                      n214 = for {
                        N: 5 -> [_]
                        i -> [w282]
                        # "行数大于零"
                        n215 = case shown="3" w282 {
                          tunnel: [w286 w287 w288 w289 w290] -> w281
                          frame 0, Default {
                            n216 = global read "全局 所有参数.vi" "氨氮"() -> (w286:string[][])
                          }
                          frame 1 {
                            n217 = global read "全局 所有参数.vi" "总氮"() -> (w287:string[][])
                          }
                          frame 2 {
                            n218 = global read "全局 所有参数.vi" "总磷"() -> (w288:string[][])
                          }
                          frame 3 {
                            n219 = global read "全局 所有参数.vi" "CODMn"() -> (w289:string[][])
                          }
                          frame 4 {
                            n220 = global read "全局 所有参数.vi" "CODCr"() -> (w290:string[][])
                          }
                        }
                        n221 = Array Size(array=w281) -> (size(s)=w284:i32[])
                        n222 = Index Array(array=w284) -> (element=w283:i32)  [unwired: 1 in]
                        n223 = Greater Than 0?(x=w283) -> (x > 0?=w285:bool)
                        n224 = case shown="真" w285 {
                          tunnel: w282 -> [_ w296]
                          tunnel: w283 -> [_ _]
                          tunnel: w281 -> [_ w294]
                          frame False {
                          }
                          frame True {
                            # "最新时间戳加1分钟"
                            n225 = Index Array(array=w294, index (row)=0 ("禁用的索引 (行)"), index (col)=0 ("禁用的索引 (列)")) -> (element=w293:string)
                            n226 = call "日期时间字符串转换分钟数加一.vi"("data[0]"=w293) -> ("日期/时间字符串"=w292:string)  [unwired: 10 in]
                            n227 = case shown="0, 默认" w296 {
                              tunnel: w292 -> [w297 w298 w299 w300 w301]
                              frame 0, Default {
                                n228 = global write "全局 时间2.vi" "氨氮零点核查索引起始时间"(w297) -> ()
                              }
                              frame 1 {
                                n229 = global write "全局 时间2.vi" "总氮零点核查索引起始时间"(w298) -> ()
                              }
                              frame 2 {
                                n230 = global write "全局 时间2.vi" "总磷零点核查索引起始时间"(w299) -> ()
                              }
                              frame 3 {
                                n231 = global write "全局 时间2.vi" "CODMn零点核查索引起始时间"(w300) -> ()
                              }
                              frame 4 {
                                n232 = global write "全局 时间2.vi" "CODCr零点核查索引起始时间"(w301) -> ()
                              }
                            }
                          }
                        }
                      }
                    }
                    frame #3 {
                      n233 = call <vilib>:"Application Directory.vi"() -> ("Application Directory"=w315:path)
                      n234 = Build Path(base path=w315, name or relative path="data\\hecha.ini" ("名称或相对路径")) -> (appended path=w313:path)
                      n235 = call <vilib>:"Open Config Data.vi"("configuration file path"=w313) -> ("error out"=w309:errorcluster, "refnum"=w312:T8)  [unwired: 8 in, 1 out]
                      n236 = call "数据处理整合 (子VI).vi"("枚举"=enum16{"实时数据排序", "小时数据排序"}."实时数据排序") -> ("已排序的数组"=w318:string[])  [unwired: 10 in]
                      n237 = vi-ref "全局 时间2.vi"() -> (w311:refnum<vi>)
                      n238 = Array Size(array=w318) -> (size(s)=w317:i32)
                      n239 = call <userlib>:"Write Panel to INI__ogtk.vi"("error in (no error)"=w309, "VI ref"=w311, "refnum"=w312) -> ("error out"=w308:errorcluster, "refnum out"=w310:T8)  [unwired: 7 in]
                      n240 = call <vilib>:"Close Config Data.vi"("error in (no error)"=w308, "refnum"=w310) -> ("error out"=w303:errorcluster, "file path"=w302:path)  [unwired: 8 in]
                      n241 = global write "全局 数据数组大小.vi" "数据数组大小"(w317) -> ()
                      n242 = Open/Create/Replace File(file path (use dialog)=w302, error in=w303) -> (refnum out=w306:refnum<file>, error out=w307:errorcluster)  [unwired: 4 in, 1 out]
                      n243 = Flush File(refnum=w306, error in=w307) -> (refnum out=w305:refnum<file>, error out=w304:errorcluster)
                      n244 = Close File(refnum=w305, error in=w304) -> ()  [unwired: 2 out]
                    }
                    frame #4 {
                      n245 = while {
                        stop <- w321 stop-if-true
                        n246 = property on="TCP服务端掉线计数" class="DigNum (严格)"() -> ("Value"=w325:i32)  [unwired: 2 in, 2 out]
                        n247 = Greater Or Equal?(x=w325, y=1) -> (x >= y?=w324:bool)
                        n248 = case shown="假" w324 {
                          frame False {
                            n249 = global read "全局 数据数组大小.vi" "数据数组大小"() -> (w328:i32)
                            n250 = Greater Than 0?(x=w328) -> (x > 0?=w327:bool)
                            n251 = case shown="真" w327 {
                              frame False {
                              }
                              frame True {
                                w329 = 0 ("禁用的索引 (列)")
                                n252 = global read "插值后的新数组.vi" "插值后的数组元素"() -> (w339:T10)
                                n253 = local read "MN"() -> (w335:string)
                                n254 = local read "PW"() -> (w334:string)
                                n255 = local read "数据发送通道"() -> (w333:enum16{"TCP", "VISA"})
                                n256 = call "数据编码.vi"("table输入"="实时数据" ("新元素/子数组"), "MN"=w335, "PW"=w334) -> ("通讯包字符串"=w331:string)  [unwired: 11 in, 1 out]
                                n257 = Unbundle By Name(w339) -> ("氨氮"=w338:string[][])
                                n258 = local write "发送报文显示"(w331) -> ()
                                n259 = Build Array(w331) -> (w341:string[])
                                n260 = call "VISATCP组合选择发送.vi"("数据发送通道"=w333, "命令"="write", "写入缓冲区"=w331) -> ("错误输出"=w330:errorcluster)  [unwired: 9 in, 3 out]
                                n261 = Index Array(array=w338, index (row)=w329, index (col)=w329) -> (element=w337:string)
                                n262 = call "发送数据记录到文档(子VI).vi"("数组"=w341) -> ()  [unwired: 9 in, 1 out]
                                n263 = local write "错误输出"(w330) -> ()
                                n264 = call "日期时间字符串转换分钟数加一.vi"("data[0]"=w337) -> ("日期/时间字符串"=w336:string)  [unwired: 10 in]
                                n265 = global write "全局 时间2.vi" "零点核查索引起始时间"(w336) -> ()
                                n266 = local write "核查数据上传"(TRUE ("数据上传")) -> ()
                              }
                            }
                          }
                          frame True {
                          }
                        }
                        n267 = Wait (ms)(milliseconds to wait=u32 500 ("等待时间（毫秒）")) -> ()  [unwired: 1 out]
                        n268 = global read "全局 数据数组大小.vi" "数据数组大小"() -> (w319:i32)
                        n269 = global read "全局 小时数据发送次数.vi" "小时数据发送次数"() -> (w323:i32)
                        n270 = Greater Or Equal?(x=w323, y=w319) -> (x >= y?=w322:bool)
                        n271 = Compound Arithmetic op=OR ("复合运算")(w322) -> (w321:bool)
                      }
                    }
                  }
                }
                frame "跨度核查" {
                  n272 = flat-sequence {
                    frame #0 {
                      n273 = global write "全局 小时数据发送次数.vi" "小时数据发送次数"(0 ("小时数据发送次数")) -> ()
                      n274 = global write "全局 实时数据参数.vi" "实时数据参数"("跨度核查") -> ()
                      n275 = global write "全局1.vi" "枚举"(enum16{"返回请求应答", "上传数据", "返回执行结果"}."上传数据" ("枚举")) -> ()
                    }
                    frame #1 {
                      n276 = call "从数据库获取数据通用可配置(子VI).vi"("table输入"="实时数据" ("新元素/子数组"), "列队名（唯一）"="c") -> ()  [unwired: 8 in, 2 out]
                    }
                    frame #2 {
                      n277 = for {
                        N: 5 -> [_]
                        i -> [w349]
                        # "行数大于零"
                        n278 = case shown="3" w349 {
                          tunnel: [w354 w355 w356 w357 w358] -> w350
                          frame 0, Default {
                            n279 = global read "全局 所有参数.vi" "氨氮"() -> (w354:string[][])
                          }
                          frame 1 {
                            n280 = global read "全局 所有参数.vi" "总氮"() -> (w355:string[][])
                          }
                          frame 2 {
                            n281 = global read "全局 所有参数.vi" "总磷"() -> (w356:string[][])
                          }
                          frame 3 {
                            n282 = global read "全局 所有参数.vi" "CODMn"() -> (w357:string[][])
                          }
                          frame 4 {
                            n283 = global read "全局 所有参数.vi" "CODCr"() -> (w358:string[][])
                          }
                        }
                        n284 = Array Size(array=w350) -> (size(s)=w352:i32[])
                        n285 = Index Array(array=w352) -> (element=w351:i32)  [unwired: 1 in]
                        n286 = Greater Than 0?(x=w351) -> (x > 0?=w353:bool)
                        n287 = case shown="真" w353 {
                          tunnel: w349 -> [_ w364]
                          tunnel: w351 -> [_ _]
                          tunnel: w350 -> [_ w362]
                          frame False {
                          }
                          frame True {
                            # "最新时间戳加1分钟"
                            n288 = Index Array(array=w362, index (row)=0 ("禁用的索引 (行)"), index (col)=0 ("禁用的索引 (列)")) -> (element=w361:string)
                            n289 = call "日期时间字符串转换分钟数加一.vi"("data[0]"=w361) -> ("日期/时间字符串"=w360:string)  [unwired: 10 in]
                            n290 = case shown="3" w364 {
                              tunnel: w360 -> [w365 w366 w367 w368 w369]
                              frame 0, Default {
                                n291 = global write "全局 时间2.vi" "氨氮跨度核查索引起始时间"(w365) -> ()
                              }
                              frame 1 {
                                n292 = global write "全局 时间2.vi" "总氮跨度核查索引起始时间"(w366) -> ()
                              }
                              frame 2 {
                                n293 = global write "全局 时间2.vi" "总磷跨度核查索引起始时间"(w367) -> ()
                              }
                              frame 3 {
                                n294 = global write "全局 时间2.vi" "CODMn跨度核查索引起始时间"(w368) -> ()
                              }
                              frame 4 {
                                n295 = global write "全局 时间2.vi" "CODCr跨度核查索引起始时间"(w369) -> ()
                              }
                            }
                          }
                        }
                      }
                    }
                    frame #3 {
                      n296 = call <vilib>:"Application Directory.vi"() -> ("Application Directory"=w383:path)
                      n297 = call "数据处理整合 (子VI).vi"("枚举"=enum16{"实时数据排序", "小时数据排序"}."实时数据排序") -> ("已排序的数组"=w386:string[])  [unwired: 10 in]
                      n298 = Build Path(base path=w383, name or relative path="data\\hecha.ini" ("名称或相对路径")) -> (appended path=w381:path)
                      n299 = call <vilib>:"Open Config Data.vi"("configuration file path"=w381) -> ("error out"=w377:errorcluster, "refnum"=w380:T8)  [unwired: 8 in, 1 out]
                      n300 = Array Size(array=w386) -> (size(s)=w385:i32)
                      n301 = vi-ref "全局 时间2.vi"() -> (w379:refnum<vi>)
                      n302 = global write "全局 数据数组大小.vi" "数据数组大小"(w385) -> ()
                      n303 = call <userlib>:"Write Panel to INI__ogtk.vi"("error in (no error)"=w377, "VI ref"=w379, "refnum"=w380) -> ("error out"=w376:errorcluster, "refnum out"=w378:T8)  [unwired: 7 in]
                      n304 = call <vilib>:"Close Config Data.vi"("error in (no error)"=w376, "refnum"=w378) -> ("error out"=w371:errorcluster, "file path"=w370:path)  [unwired: 8 in]
                      n305 = Open/Create/Replace File(file path (use dialog)=w370, error in=w371) -> (refnum out=w374:refnum<file>, error out=w375:errorcluster)  [unwired: 4 in, 1 out]
                      n306 = Flush File(refnum=w374, error in=w375) -> (refnum out=w373:refnum<file>, error out=w372:errorcluster)
                      n307 = Close File(refnum=w373, error in=w372) -> ()  [unwired: 2 out]
                    }
                    frame #4 {
                      n308 = while {
                        stop <- w389 stop-if-true
                        n309 = property on="TCP服务端掉线计数" class="DigNum (严格)"() -> ("Value"=w393:i32)  [unwired: 2 in, 2 out]
                        n310 = property on="TCP服务端掉线计数" class="DigNum (严格)" props=["Value"]() -> ()  [unwired: 2 in, 3 out]
                        n311 = Greater Or Equal?(x=w393, y=1) -> (x >= y?=w392:bool)
                        n312 = case shown="假" w392 {
                          frame False {
                            n313 = global read "全局 数据数组大小.vi" "数据数组大小"() -> (w396:i32)
                            n314 = Greater Than 0?(x=w396) -> (x > 0?=w395:bool)
                            n315 = case shown="真" w395 {
                              frame False {
                              }
                              frame True {
                                w397 = 0 ("禁用的索引 (列)")
                                n316 = global read "插值后的新数组.vi" "插值后的数组元素"() -> (w407:T10)
                                n317 = local read "QN"() -> (w410:string)
                                n318 = local read "MN"() -> (w403:string)
                                n319 = local read "PW"() -> (w402:string)
                                n320 = local read "数据发送通道"() -> (w401:enum16{"TCP", "VISA"})
                                n321 = Unbundle By Name(w407) -> ("氨氮"=w406:string[][])
                                n322 = call "数据编码.vi"("table输入"="实时数据" ("新元素/子数组"), "QN"=w410, "MN"=w403, "PW"=w402) -> ("通讯包字符串"=w399:string)  [unwired: 10 in, 1 out]
                                n323 = local write "发送报文显示"(w399) -> ()
                                n324 = Index Array(array=w406, index (row)=w397, index (col)=w397) -> (element=w405:string)
                                n325 = call "VISATCP组合选择发送.vi"("数据发送通道"=w401, "命令"="write", "写入缓冲区"=w399) -> ("错误输出"=w398:errorcluster)  [unwired: 9 in, 3 out]
                                n326 = Build Array(w399) -> (w409:string[])
                                n327 = local write "核查数据上传"(TRUE ("数据上传")) -> ()
                                n328 = call "日期时间字符串转换分钟数加一.vi"("data[0]"=w405) -> ("日期/时间字符串"=w404:string)  [unwired: 10 in]
                                n329 = local write "错误输出"(w398) -> ()
                                n330 = call "发送数据记录到文档(子VI).vi"("数组"=w409) -> ()  [unwired: 9 in, 1 out]
                                n331 = global write "全局 时间2.vi" "跨度核查索引起始时间"(w404) -> ()
                              }
                            }
                          }
                          frame True {
                          }
                        }
                        n332 = Wait (ms)(milliseconds to wait=u32 500 ("等待时间（毫秒）")) -> ()  [unwired: 1 out]
                        n333 = global read "全局 数据数组大小.vi" "数据数组大小"() -> (w387:i32)
                        n334 = global read "全局 小时数据发送次数.vi" "小时数据发送次数"() -> (w391:i32)
                        n335 = Greater Or Equal?(x=w391, y=w387) -> (x >= y?=w390:bool)
                        n336 = Compound Arithmetic op=OR ("复合运算")(w390) -> (w389:bool)
                      }
                    }
                  }
                }
                frame "标样核查" {
                  n337 = flat-sequence {
                    tunnel: [w421] -> w412
                    frame #0 {
                      n338 = global write "全局 小时数据发送次数.vi" "小时数据发送次数"(0 ("小时数据发送次数")) -> ()
                      n339 = global write "全局 实时数据参数.vi" "实时数据参数"("核查数据") -> ()
                      n340 = global write "全局1.vi" "枚举"(enum16{"返回请求应答", "上传数据", "返回执行结果"}."上传数据" ("枚举")) -> ()
                    }
                    frame #1 {
                      n341 = call "从数据库获取数据通用可配置(子VI).vi"("table输入"="实时数据" ("新元素/子数组"), "列队名（唯一）"="n") -> ()  [unwired: 8 in, 2 out]
                    }
                    frame #2 {
                      n342 = call "数据处理整合 (子VI).vi"("枚举"=enum16{"实时数据排序", "小时数据排序"}."实时数据排序") -> ("已排序的数组"=w420:string[])  [unwired: 10 in]
                      n343 = Array Size(array=w420) -> (size(s)=w419:i32)
                      n344 = global write "全局 数据数组大小.vi" "数据数组大小"(w419) -> ()
                    }
                    frame #3 {
                      n345 = while {
                        tunnel: [w422] -> w421
                        stop <- w422 stop-if-true
                        n346 = property on="TCP服务端掉线计数" class="DigNum (严格)"() -> ("Value"=w428:i32)  [unwired: 2 in, 2 out]
                        n347 = property on="TCP服务端掉线计数" class="DigNum (严格)" props=["Value"]() -> ()  [unwired: 2 in, 3 out]
                        n348 = Greater Or Equal?(x=w428, y=1) -> (x >= y?=w427:bool)
                        n349 = case shown="假" w427 {
                          frame False {
                            n350 = global read "全局 数据数组大小.vi" "数据数组大小"() -> (w431:i32)
                            n351 = Greater Than 0?(x=w431) -> (x > 0?=w430:bool)
                            n352 = case shown="真" w430 {
                              frame False {
                              }
                              frame True {
                                w432 = 0 ("禁用的索引 (列)")
                                n353 = global read "插值后的新数组.vi" "插值后的数组元素"() -> (w442:T10)
                                n354 = local read "QN"() -> (w445:string)
                                n355 = local read "MN"() -> (w438:string)
                                n356 = local read "PW"() -> (w437:string)
                                n357 = local read "数据发送通道"() -> (w436:enum16{"TCP", "VISA"})
                                n358 = Unbundle By Name(w442) -> ("氨氮"=w441:string[][])
                                n359 = call "数据编码.vi"("table输入"="实时数据" ("新元素/子数组"), "QN"=w445, "MN"=w438, "PW"=w437) -> ("通讯包字符串"=w434:string)  [unwired: 10 in, 1 out]
                                n360 = local write "发送报文显示"(w434) -> ()
                                n361 = call "VISATCP组合选择发送.vi"("数据发送通道"=w436, "命令"="write", "写入缓冲区"=w434) -> ("错误输出"=w433:errorcluster)  [unwired: 9 in, 3 out]
                                n362 = Index Array(array=w441, index (row)=w432, index (col)=w432) -> (element=w440:string)
                                n363 = Build Array(w434) -> (w444:string[])
                                n364 = local write "核查数据上传"(TRUE ("数据上传")) -> ()
                                n365 = call "日期时间字符串转换分钟数加一.vi"("data[0]"=w440) -> ("日期/时间字符串"=w439:string)  [unwired: 10 in]
                                n366 = local write "错误输出"(w433) -> ()
                                n367 = call "发送数据记录到文档(子VI).vi"("数组"=w444) -> ()  [unwired: 9 in, 1 out]
                                n368 = global write "全局 时间2.vi" "标样核查索引起始时间"(w439) -> ()
                              }
                            }
                          }
                          frame True {
                          }
                        }
                        n369 = Wait (ms)(milliseconds to wait=u32 500 ("等待时间（毫秒）")) -> ()  [unwired: 1 out]
                        n370 = global read "全局 数据数组大小.vi" "数据数组大小"() -> (w423:i32)
                        n371 = global read "全局 小时数据发送次数.vi" "小时数据发送次数"() -> (w426:i32)
                        n372 = Greater Or Equal?(x=w426, y=w423) -> (x >= y?=w425:bool)
                        n373 = Compound Arithmetic op=OR ("复合运算")(w425) -> (w422:bool)
                      }
                    }
                  }
                }
                frame "加标回收" {
                  n374 = flat-sequence {
                    frame #0 {
                      n375 = global write "全局 小时数据发送次数.vi" "小时数据发送次数"(0 ("小时数据发送次数")) -> ()
                      n376 = global write "全局 实时数据参数.vi" "实时数据参数"("加标回收测试") -> ()
                      n377 = global write "全局1.vi" "枚举"(enum16{"返回请求应答", "上传数据", "返回执行结果"}."上传数据" ("枚举")) -> ()
                    }
                    frame #1 {
                      n378 = call "从数据库获取数据通用可配置(子VI).vi"("table输入"="加标回收" ("新元素/子数组"), "列队名（唯一）"="d") -> ()  [unwired: 8 in, 2 out]
                    }
                    frame #2 {
                      n379 = call "加标回收数据处理整合 (子VI).vi"("枚举"=enum16{"实时数据排序", "小时数据排序"}."实时数据排序") -> ("已排序的数组"=w453:string[])  [unwired: 10 in]
                      n380 = Array Size(array=w453) -> (size(s)=w454:i32)
                      n381 = global write "全局 数据数组大小.vi" "数据数组大小"(w454) -> ()
                    }
                    frame #3 {
                      n382 = while {
                        stop <- w457 stop-if-true
                        n383 = property on="TCP服务端掉线计数" class="DigNum (严格)"() -> ("Value"=w462:i32)  [unwired: 2 in, 2 out]
                        n384 = Greater Or Equal?(x=w462, y=1) -> (x >= y?=w460:bool)
                        n385 = case shown="假" w460 {
                          frame False {
                            n386 = global read "全局 数据数组大小.vi" "数据数组大小"() -> (w464:i32)
                            n387 = Greater Than 0?(x=w464) -> (x > 0?=w463:bool)
                            n388 = case shown="真" w463 {
                              frame False {
                              }
                              frame True {
                                n389 = global read "全局 数据数组大小.vi" "数据数组大小"() -> (w474:i32)
                                n390 = global read "插值后的新数组.vi" "插值后的数组元素"() -> (w477:T10)
                                n391 = local read "MN"() -> (w470:string)
                                n392 = local read "PW"() -> (w469:string)
                                n393 = local read "数据发送通道"() -> (w468:enum16{"TCP", "VISA"})
                                n394 = Decrement(x=w474) -> (x-1=w473:i32)
                                n395 = call "数据编码.vi"("table输入"="实时数据" ("新元素/子数组"), "MN"=w470, "PW"=w469) -> ("通讯包字符串"=w466:string)  [unwired: 11 in, 1 out]
                                n396 = Unbundle By Name(w477) -> ("氨氮"=w476:string[][])
                                n397 = local write "发送报文显示"(w466) -> ()
                                n398 = call "VISATCP组合选择发送.vi"("数据发送通道"=w468, "命令"="write", "写入缓冲区"=w466) -> ("错误输出"=w465:errorcluster)  [unwired: 9 in, 3 out]
                                n399 = Index Array(array=w476, index (row)=w473, index (col)=0 ("禁用的索引 (列)")) -> (element=w472:string)
                                n400 = local write "核查数据上传"(TRUE ("数据上传")) -> ()
                                n401 = Build Array(w466) -> (w479:string[])
                                n402 = call "日期时间字符串转换分钟数加一.vi"("data[0]"=w472) -> ("日期/时间字符串"=w471:string)  [unwired: 10 in]
                                n403 = local write "错误输出"(w465) -> ()
                                n404 = call "发送数据记录到文档(子VI).vi"("数组"=w479) -> ()  [unwired: 9 in, 1 out]
                                n405 = global write "全局 时间2.vi" "加标回收索引起始时间"(w471) -> ()
                              }
                            }
                          }
                          frame True {
                          }
                        }
                        n406 = Wait (ms)(milliseconds to wait=u32 500 ("等待时间（毫秒）")) -> ()  [unwired: 1 out]
                        n407 = global read "全局 数据数组大小.vi" "数据数组大小"() -> (w455:i32)
                        n408 = global read "全局 小时数据发送次数.vi" "小时数据发送次数"() -> (w459:i32)
                        n409 = Greater Or Equal?(x=w459, y=w455) -> (x >= y?=w458:bool)
                        n410 = Compound Arithmetic op=OR ("复合运算")(w458) -> (w457:bool)
                      }
                    }
                  }
                }
                frame "平行样" {
                  n411 = flat-sequence {
                    frame #0 {
                      n412 = global write "全局 小时数据发送次数.vi" "小时数据发送次数"(0 ("小时数据发送次数")) -> ()
                      n413 = global write "全局 实时数据参数.vi" "实时数据参数"("平行样测试") -> ()
                      n414 = global write "全局1.vi" "枚举"(enum16{"返回请求应答", "上传数据", "返回执行结果"}."上传数据" ("枚举")) -> ()
                    }
                    frame #1 {
                      n415 = call "从数据库获取数据通用可配置(子VI).vi"("table输入"="平行样测试" ("新元素/子数组"), "列队名（唯一）"="e") -> ()  [unwired: 8 in, 2 out]
                    }
                    frame #2 {
                      n416 = for {
                        N: 5 -> [_]
                        i -> [w487]
                        # "行数大于零"
                        n417 = case shown="3" w487 {
                          tunnel: [w492 w493 w494 w495 w496] -> w488
                          frame 0, Default {
                            n418 = global read "全局 所有参数.vi" "氨氮"() -> (w492:string[][])
                          }
                          frame 1 {
                            n419 = global read "全局 所有参数.vi" "总氮"() -> (w493:string[][])
                          }
                          frame 2 {
                            n420 = global read "全局 所有参数.vi" "总磷"() -> (w494:string[][])
                          }
                          frame 3 {
                            n421 = global read "全局 所有参数.vi" "CODMn"() -> (w495:string[][])
                          }
                          frame 4 {
                            n422 = global read "全局 所有参数.vi" "CODCr"() -> (w496:string[][])
                          }
                        }
                        n423 = Array Size(array=w488) -> (size(s)=w490:i32[])
                        n424 = Index Array(array=w490) -> (element=w489:i32)  [unwired: 1 in]
                        n425 = Greater Than 0?(x=w489) -> (x > 0?=w491:bool)
                        n426 = case shown="真" w491 {
                          tunnel: w487 -> [_ w502]
                          tunnel: w489 -> [_ _]
                          tunnel: w488 -> [_ w500]
                          frame False {
                          }
                          frame True {
                            # "最新时间戳加1分钟"
                            n427 = Index Array(array=w500, index (row)=0 ("禁用的索引 (行)"), index (col)=0 ("禁用的索引 (列)")) -> (element=w499:string)
                            n428 = call "日期时间字符串转换分钟数加一.vi"("data[0]"=w499) -> ("日期/时间字符串"=w498:string)  [unwired: 10 in]
                            n429 = case shown="0, 默认" w502 {
                              tunnel: w498 -> [w503 w504 w505 w506 w507]
                              frame 0, Default {
                                n430 = global write "全局 时间2.vi" "氨氮平行样索引起始时间"(w503) -> ()
                              }
                              frame 1 {
                                n431 = global write "全局 时间2.vi" "总氮平行样索引起始时间"(w504) -> ()
                              }
                              frame 2 {
                                n432 = global write "全局 时间2.vi" "总磷平行样索引起始时间"(w505) -> ()
                              }
                              frame 3 {
                                n433 = global write "全局 时间2.vi" "CODMn平行样索引起始时间"(w506) -> ()
                              }
                              frame 4 {
                                n434 = global write "全局 时间2.vi" "CODCr平行样索引起始时间"(w507) -> ()
                              }
                            }
                          }
                        }
                      }
                    }
                    frame #3 {
                      n435 = call "数据处理整合 (子VI).vi"("枚举"=enum16{"实时数据排序", "小时数据排序"}."实时数据排序") -> ("已排序的数组"=w524:string[])  [unwired: 10 in]
                      n436 = Array Size(array=w524) -> (size(s)=w523:i32)
                      n437 = call <vilib>:"Application Directory.vi"() -> ("Application Directory"=w521:path)
                      n438 = Build Path(base path=w521, name or relative path="data\\hecha.ini" ("名称或相对路径")) -> (appended path=w519:path)
                      n439 = global write "全局 数据数组大小.vi" "数据数组大小"(w523) -> ()
                      n440 = call <vilib>:"Open Config Data.vi"("configuration file path"=w519) -> ("error out"=w515:errorcluster, "refnum"=w518:T8)  [unwired: 8 in, 1 out]
                      n441 = vi-ref "全局 时间2.vi"() -> (w517:refnum<vi>)
                      n442 = call <userlib>:"Write Panel to INI__ogtk.vi"("error in (no error)"=w515, "VI ref"=w517, "refnum"=w518) -> ("error out"=w514:errorcluster, "refnum out"=w516:T8)  [unwired: 7 in]
                      n443 = call <vilib>:"Close Config Data.vi"("error in (no error)"=w514, "refnum"=w516) -> ("error out"=w509:errorcluster, "file path"=w508:path)  [unwired: 8 in]
                      n444 = Open/Create/Replace File(file path (use dialog)=w508, error in=w509) -> (refnum out=w512:refnum<file>, error out=w513:errorcluster)  [unwired: 4 in, 1 out]
                      n445 = Flush File(refnum=w512, error in=w513) -> (refnum out=w511:refnum<file>, error out=w510:errorcluster)
                      n446 = Close File(refnum=w511, error in=w510) -> ()  [unwired: 2 out]
                    }
                    frame #4 {
                      n447 = while {
                        stop <- w527 stop-if-true
                        n448 = property on="TCP服务端掉线计数" class="DigNum (严格)"() -> ("Value"=w533:i32)  [unwired: 2 in, 2 out]
                        n449 = property on="TCP服务端掉线计数" class="DigNum (严格)" props=["Value"]() -> ()  [unwired: 2 in, 3 out]
                        n450 = Greater Or Equal?(x=w533, y=1) -> (x >= y?=w531:bool)
                        n451 = case shown="假" w531 {
                          frame False {
                            n452 = global read "全局 数据数组大小.vi" "数据数组大小"() -> (w535:i32)
                            n453 = Greater Than 0?(x=w535) -> (x > 0?=w534:bool)
                            n454 = case shown="真" w534 {
                              frame False {
                              }
                              frame True {
                                n455 = local read "MN"() -> (w541:string)
                                n456 = local read "PW"() -> (w540:string)
                                n457 = local read "数据发送通道"() -> (w539:enum16{"TCP", "VISA"})
                                n458 = local write "核查数据上传"(TRUE ("数据上传")) -> ()
                                n459 = call "数据编码.vi"("table输入"="实时数据" ("新元素/子数组"), "MN"=w541, "PW"=w540) -> ("通讯包字符串"=w537:string)  [unwired: 11 in, 1 out]
                                n460 = local write "发送报文显示"(w537) -> ()
                                n461 = call "VISATCP组合选择发送.vi"("数据发送通道"=w539, "命令"="write", "写入缓冲区"=w537) -> ("错误输出"=w536:errorcluster)  [unwired: 9 in, 3 out]
                                n462 = Build Array(w537) -> (w543:string[])
                                n463 = call "发送数据记录到文档(子VI).vi"("数组"=w543) -> ()  [unwired: 9 in, 1 out]
                                n464 = local write "错误输出"(w536) -> ()
                              }
                            }
                          }
                          frame True {
                          }
                        }
                        n465 = Wait (ms)(milliseconds to wait=u32 500 ("等待时间（毫秒）")) -> ()  [unwired: 1 out]
                        n466 = global read "全局 数据数组大小.vi" "数据数组大小"() -> (w530:i32)
                        n467 = global read "全局 小时数据发送次数.vi" "小时数据发送次数"() -> (w529:i32)
                        n468 = Decrement(x=w530) -> (x-1=w526:i32)
                        n469 = Greater Or Equal?(x=w529, y=w526) -> (x >= y?=w528:bool)
                        n470 = Compound Arithmetic op=OR ("复合运算")(w528) -> (w527:bool)
                      }
                    }
                  }
                }
                frame "集成干预" {
                  n471 = flat-sequence {
                    frame #0 {
                      n472 = global write "全局 小时数据发送次数.vi" "小时数据发送次数"(0 ("小时数据发送次数")) -> ()
                      n473 = global write "全局 实时数据参数.vi" "实时数据参数"("集成干预测试") -> ()
                      n474 = global write "全局1.vi" "枚举"(enum16{"返回请求应答", "上传数据", "返回执行结果"}."上传数据" ("枚举")) -> ()
                    }
                    frame #1 {
                      n475 = call "从数据库获取数据通用可配置(子VI).vi"("table输入"="集成干预测试" ("新元素/子数组"), "列队名（唯一）"="f") -> ()  [unwired: 8 in, 2 out]
                    }
                    frame #2 {
                      n476 = for {
                        N: 10 -> [_]
                        i -> [w551]
                        # "行数大于零"
                        n477 = case shown="9" w551 {
                          tunnel: [w556 w557 w558 w559 w560 w561 w562 w563 w564 w565] -> w552
                          frame 0, Default {
                            n478 = global read "全局 所有参数.vi" "氨氮"() -> (w556:string[][])
                          }
                          frame 1 {
                            n479 = global read "全局 所有参数.vi" "总氮"() -> (w557:string[][])
                          }
                          frame 2 {
                            n480 = global read "全局 所有参数.vi" "总磷"() -> (w558:string[][])
                          }
                          frame 3 {
                            n481 = global read "全局 所有参数.vi" "CODMn"() -> (w559:string[][])
                          }
                          frame 4 {
                            n482 = global read "全局 所有参数.vi" "CODCr"() -> (w560:string[][])
                          }
                          frame 5 {
                            n483 = global read "全局 所有参数.vi" "DO"() -> (w561:string[][])
                          }
                          frame 6 {
                            n484 = global read "全局 所有参数.vi" "PH"() -> (w562:string[][])
                          }
                          frame 7 {
                            n485 = global read "全局 所有参数.vi" "电导率"() -> (w563:string[][])
                          }
                          frame 8 {
                            n486 = global read "全局 所有参数.vi" "水温"() -> (w564:string[][])
                          }
                          frame 9 {
                            n487 = global read "全局 所有参数.vi" "浊度"() -> (w565:string[][])
                          }
                        }
                        n488 = Array Size(array=w552) -> (size(s)=w554:i32[])
                        n489 = Index Array(array=w554) -> (element=w553:i32)  [unwired: 1 in]
                        n490 = Greater Than 0?(x=w553) -> (x > 0?=w555:bool)
                        n491 = case shown="真" w555 {
                          tunnel: w551 -> [_ w571]
                          tunnel: w553 -> [_ _]
                          tunnel: w552 -> [_ w569]
                          frame False {
                          }
                          frame True {
                            # "最新时间戳加1分钟"
                            n492 = Index Array(array=w569, index (row)=0 ("禁用的索引 (行)"), index (col)=0 ("禁用的索引 (列)")) -> (element=w568:string)
                            n493 = call "日期时间字符串转换分钟数加一.vi"("data[0]"=w568) -> ("日期/时间字符串"=w567:string)  [unwired: 10 in]
                            n494 = case shown="9" w571 {
                              tunnel: w567 -> [w572 w573 w574 w575 w576 w577 w578 w579 w580 w581]
                              frame 0, Default {
                                n495 = global write "全局 时间2.vi" "氨氮集成干预索引起始时间"(w572) -> ()
                              }
                              frame 1 {
                                n496 = global write "全局 时间2.vi" "总氮集成干预索引起始时间"(w573) -> ()
                              }
                              frame 2 {
                                n497 = global write "全局 时间2.vi" "总磷集成干预索引起始时间"(w574) -> ()
                              }
                              frame 3 {
                                n498 = global write "全局 时间2.vi" "CODMn集成干预索引起始时间"(w575) -> ()
                              }
                              frame 4 {
                                n499 = global write "全局 时间2.vi" "CODCr集成干预索引起始时间"(w576) -> ()
                              }
                              frame 5 {
                                n500 = global write "全局 时间2.vi" "DO集成干预索引起始时间"(w577) -> ()
                              }
                              frame 6 {
                                n501 = global write "全局 时间2.vi" "PH集成干预索引起始时间"(w578) -> ()
                              }
                              frame 7 {
                                n502 = global write "全局 时间2.vi" "比电导率集成干预索引起始时间"(w579) -> ()
                              }
                              frame 8 {
                                n503 = global write "全局 时间2.vi" "水温集成干预索引起始时间"(w580) -> ()
                              }
                              frame 9 {
                                n504 = global write "全局 时间2.vi" "浊度集成干预索引起始时间"(w581) -> ()
                              }
                            }
                          }
                        }
                      }
                    }
                    frame #3 {
                      n505 = call "数据处理整合 (子VI).vi"("枚举"=enum16{"实时数据排序", "小时数据排序"}."实时数据排序") -> ("已排序的数组"=w598:string[])  [unwired: 10 in]
                      n506 = Array Size(array=w598) -> (size(s)=w597:i32)
                      n507 = call <vilib>:"Application Directory.vi"() -> ("Application Directory"=w595:path)
                      n508 = Build Path(base path=w595, name or relative path="data\\hecha.ini" ("名称或相对路径")) -> (appended path=w593:path)
                      n509 = global write "全局 数据数组大小.vi" "数据数组大小"(w597) -> ()
                      n510 = call <vilib>:"Open Config Data.vi"("configuration file path"=w593) -> ("error out"=w589:errorcluster, "refnum"=w592:T8)  [unwired: 8 in, 1 out]
                      n511 = vi-ref "全局 时间2.vi"() -> (w591:refnum<vi>)
                      n512 = call <userlib>:"Write Panel to INI__ogtk.vi"("error in (no error)"=w589, "VI ref"=w591, "refnum"=w592) -> ("error out"=w588:errorcluster, "refnum out"=w590:T8)  [unwired: 7 in]
                      n513 = call <vilib>:"Close Config Data.vi"("error in (no error)"=w588, "refnum"=w590) -> ("error out"=w583:errorcluster, "file path"=w582:path)  [unwired: 8 in]
                      n514 = Open/Create/Replace File(file path (use dialog)=w582, error in=w583) -> (refnum out=w586:refnum<file>, error out=w587:errorcluster)  [unwired: 4 in, 1 out]
                      n515 = Flush File(refnum=w586, error in=w587) -> (refnum out=w585:refnum<file>, error out=w584:errorcluster)
                      n516 = Close File(refnum=w585, error in=w584) -> ()  [unwired: 2 out]
                    }
                    frame #4 {
                      n517 = while {
                        stop <- w601 stop-if-true
                        n518 = property on="TCP服务端掉线计数" class="DigNum (严格)"() -> ("Value"=w607:i32)  [unwired: 2 in, 2 out]
                        n519 = property on="TCP服务端掉线计数" class="DigNum (严格)" props=["Value"]() -> ()  [unwired: 2 in, 3 out]
                        n520 = Greater Or Equal?(x=w607, y=1) -> (x >= y?=w605:bool)
                        n521 = case shown="假" w605 {
                          frame False {
                            n522 = global read "全局 数据数组大小.vi" "数据数组大小"() -> (w609:i32)
                            n523 = Greater Than 0?(x=w609) -> (x > 0?=w608:bool)
                            n524 = case shown="真" w608 {
                              frame False {
                              }
                              frame True {
                                n525 = local read "MN"() -> (w615:string)
                                n526 = local read "PW"() -> (w614:string)
                                n527 = local read "数据发送通道"() -> (w613:enum16{"TCP", "VISA"})
                                n528 = local write "核查数据上传"(TRUE ("数据上传")) -> ()
                                n529 = call "数据编码.vi"("table输入"="实时数据" ("新元素/子数组"), "MN"=w615, "PW"=w614) -> ("通讯包字符串"=w611:string)  [unwired: 11 in, 1 out]
                                n530 = local write "发送报文显示"(w611) -> ()
                                n531 = call "VISATCP组合选择发送.vi"("数据发送通道"=w613, "命令"="write", "写入缓冲区"=w611) -> ("错误输出"=w610:errorcluster)  [unwired: 9 in, 3 out]
                                n532 = Build Array(w611) -> (w617:string[])
                                n533 = call "发送数据记录到文档(子VI).vi"("数组"=w617) -> ()  [unwired: 9 in, 1 out]
                                n534 = local write "错误输出"(w610) -> ()
                              }
                            }
                          }
                          frame True {
                          }
                        }
                        n535 = Wait (ms)(milliseconds to wait=u32 500 ("等待时间（毫秒）")) -> ()  [unwired: 1 out]
                        n536 = global read "全局 数据数组大小.vi" "数据数组大小"() -> (w604:i32)
                        n537 = global read "全局 小时数据发送次数.vi" "小时数据发送次数"() -> (w603:i32)
                        n538 = Decrement(x=w604) -> (x-1=w600:i32)
                        n539 = Greater Or Equal?(x=w603, y=w600) -> (x >= y?=w602:bool)
                        n540 = Compound Arithmetic op=OR ("复合运算")(w602) -> (w601:bool)
                      }
                    }
                  }
                }
                frame "", Default {
                  n541 = Get Queue Status(queue=w622) -> (# elements in queue=w621:i32)  [unwired: 2 in, 7 out]
                  n542 = Equal To 0?(x=w621) -> (x = 0?=w620:bool)
                  n543 = case shown="真" w620 {
                    tunnel: [_ TRUE] -> w619
                    frame False {
                    }
                    frame True {
                    }
                  }
                }
              }
              n544 = Wait (ms)(milliseconds to wait=u32 1000 ("等待时间（毫秒）")) -> ()  [unwired: 1 out]
            }
          }
          frame "小时数据" {
            # "间隔时间上传"
            n545 = flat-sequence {
              frame #0 {
                # "发送前2小时的数据"
                n546 = global write "全局 小时数据发送次数.vi" "小时数据发送次数"(1 ("小时数据发送次数")) -> ()
                n547 = global write "全局1.vi" "枚举"(enum16{"返回请求应答", "上传数据", "返回执行结果"}."上传数据" ("枚举")) -> ()
              }
              frame #1 {
                n548 = call "从数据库获取数据通用可配置(子VI).vi"("table输入"="小时数据" ("新元素/子数组"), "列队名（唯一）"="XS" ("名称（未命名）")) -> ()  [unwired: 8 in, 2 out]
              }
              frame #2 {
                n549 = property on="TCP服务端掉线计数" class="DigNum (严格)"() -> ("Value"=w629:i32)  [unwired: 2 in, 2 out]
                n550 = Greater Or Equal?(x=w629, y=1) -> (x >= y?=w628:bool)
                n551 = case shown="假" w628 {
                  frame False {
                    # "数据处理整合"
                    n552 = call "实时小时数据处理整合 (子VI).vi"("枚举"=enum16{"实时数据排序", "小时数据排序"}."小时数据排序") -> ("已排序的数组"=w631:string[])  [unwired: 10 in]
                    n553 = Array Size(array=w631) -> (size(s)=w634:i32)
                    n554 = global write "全局 数据数组大小.vi" "数据数组大小"(1 ("数据数组大小")) -> ()
                    n555 = Greater Than 0?(x=w634) -> (x > 0?=w635:bool)
                    n556 = case shown="真" w635 {
                      frame False {
                      }
                      frame True {
                        n557 = local write "核查数据上传"(TRUE ("数据上传")) -> ()
                        n558 = Get Date/Time In Seconds() -> (seconds since 1Jan1904=w646:timestamp)
                        n559 = Format Date/Time String(time format string (%c)="%Y%m%d%H%M%S%3u" ("时间格式字符串(%c)"), seconds (now)=w646) -> (date/time string=w647:string)  [unwired: 1 in]
                        n560 = local read "MN"() -> (w641:string)
                        n561 = local read "PW"() -> (w640:string)
                        n562 = Search and Replace String(input string=w647, search string="." ("搜索字符串")) -> (result string=w649:string)  [unwired: 6 in, 3 out]
                        n563 = local read "数据发送通道"() -> (w639:enum16{"TCP", "VISA"})
                        n564 = call "数据编码.vi"("table输入"="小时数据" ("新元素/子数组"), "QN"=w649, "MN"=w641, "PW"=w640) -> ("通讯包字符串"=w637:string)  [unwired: 10 in, 1 out]
                        n565 = local write "发送报文显示"(w637) -> ()
                        n566 = call "VISATCP组合选择发送.vi"("数据发送通道"=w639, "命令"="write", "写入缓冲区"=w637) -> ("错误输出"=w636:errorcluster)  [unwired: 9 in, 3 out]
                        n567 = Build Array(w637) -> (w643:string[])
                        n568 = local write "错误输出"(w636) -> ()
                        n569 = call "发送数据记录到文档(子VI).vi"("数组"=w643) -> ()  [unwired: 9 in, 1 out]
                      }
                    }
                  }
                  frame True {
                  }
                }
              }
            }
          }
          frame "操作日志" {
            # "间隔时间上传"
            # "直接1分钟查询 一次,有数据就按数据上传,没数据就不上传,在数据发送那边有做处理"
            n570 = flat-sequence {
              frame #0 {
                # "时间"
                n571 = global read "全局 数据发送重叠.vi" "数据发送重叠开始时间戳"() -> (w651:string)
                n572 = global read "全局 数据发送重叠.vi" "数据发送重叠"() -> (w650:bool)
                n573 = global write "全局 小时数据发送次数.vi" "小时数据发送次数"(0 ("小时数据发送次数")) -> ()
                n574 = global write "全局1.vi" "枚举"(enum16{"返回请求应答", "上传数据", "返回执行结果"}."上传数据" ("枚举")) -> ()
                n575 = call "日志信息主动发送(子VI).vi"("是否正在查询数据"=w650, "查询数据发送时间节点"=w651) -> ()  [unwired: 10 in]
              }
              frame #1 {
                n576 = call "获取操作日志 (子VI).vi"("table输入"="操作日志") -> ()  [unwired: 11 in]
              }
              frame #2 {
                n577 = call "数据处理整合 (子VI).vi"("枚举"=enum16{"实时数据排序", "小时数据排序"}."实时数据排序") -> ("已排序的数组"=w657:string[])  [unwired: 10 in]
                n578 = Array Size(array=w657) -> (size(s)=w656:i32)
                n579 = global write "全局 数据数组大小.vi" "数据数组大小"(w656) -> ()
              }
              frame #3 {
                n580 = while {
                  stop <- w658 stop-if-true
                  # "判定是否存表"
                  n581 = property on="TCP服务端掉线计数" class="DigNum (严格)"() -> ("Value"=w664:i32)  [unwired: 2 in, 2 out]
                  n582 = Greater Or Equal?(x=w664, y=1) -> (x >= y?=w663:bool)
                  n583 = case shown="假" w663 {
                    frame False {
                      n584 = global read "全局 数据数组大小.vi" "数据数组大小"() -> (w666:i32)
                      n585 = Greater Than 0?(x=w666) -> (x > 0?=w667:bool)
                      n586 = case shown="真" w667 {
                        frame False {
                        }
                        frame True {
                          n587 = global read "全局 小时数据发送次数.vi" "小时数据发送次数"() -> (w676:i32)
                          n588 = local write "核查数据上传"(TRUE ("数据上传")) -> ()
                          n589 = Get Date/Time In Seconds() -> (seconds since 1Jan1904=w681:timestamp)
                          n590 = Increment(x=w676) -> (x+1=w675:i32)
                          n591 = Format Date/Time String(time format string (%c)="%Y%m%d%H%M%S%3u" ("时间格式字符串(%c)"), seconds (now)=w681) -> (date/time string=w680:string)  [unwired: 1 in]
                          n592 = global write "全局 小时数据发送次数.vi" "小时数据发送次数"(w675) -> ()
                          n593 = Search and Replace String(input string=w680, search string="." ("搜索字符串")) -> (result string=w678:string)  [unwired: 6 in, 3 out]
                          n594 = local read "MN"() -> (w673:string)
                          n595 = local read "PW"() -> (w672:string)
                          n596 = call "数据编码.vi"("table输入"="操作日志" ("新元素/子数组"), "QN"=w678, "MN"=w673, "PW"=w672) -> ("通讯包字符串"=w669:string)  [unwired: 10 in, 1 out]
                          n597 = local read "数据发送通道"() -> (w671:enum16{"TCP", "VISA"})
                          n598 = local write "发送报文显示"(w669) -> ()
                          n599 = call "VISATCP组合选择发送.vi"("数据发送通道"=w671, "命令"="write", "写入缓冲区"=w669) -> ("错误输出"=w668:errorcluster)  [unwired: 9 in, 3 out]
                          n600 = Build Array(w669) -> (w677:string[])
                          n601 = local write "错误输出"(w668) -> ()
                          n602 = call "发送数据记录到文档(子VI).vi"("数组"=w677) -> ()  [unwired: 9 in, 1 out]
                        }
                      }
                    }
                    frame True {
                    }
                  }
                  n603 = Wait (ms)(milliseconds to wait=u32 500 ("等待时间（毫秒）")) -> ()  [unwired: 1 out]
                  n604 = global read "全局 数据数组大小.vi" "数据数组大小"() -> (w660:i32)
                  n605 = global read "全局 小时数据发送次数.vi" "小时数据发送次数"() -> (w662:i32)
                  n606 = Decrement(x=w660) -> (x-1=w659:i32)
                  n607 = Greater Or Equal?(x=w662, y=w659) -> (x >= y?=w658:bool)
                }
              }
            }
          }
          frame "仪器参数" {
            # "间隔时间上传"
            # "直接1分钟查询 一次,有数据就按数据上传,没数据就不上传,在数据发送那边有做处理"
            n608 = flat-sequence {
              frame #0 {
                # "时间"
                n609 = global write "全局 小时数据发送次数.vi" "小时数据发送次数"(0 ("小时数据发送次数")) -> ()
                n610 = global write "全局1.vi" "枚举"(enum16{"返回请求应答", "上传数据", "返回执行结果"}."上传数据" ("枚举")) -> ()
              }
              frame #1 {
                n611 = call "获取操作日志 (子VI).vi"("table输入"="仪器参数") -> ()  [unwired: 11 in]
              }
              frame #2 {
                n612 = for {
                  N: 5 -> [_]
                  i -> [w688]
                  # "行数大于零"
                  n613 = case shown="3" w688 {
                    tunnel: [w693 w694 w695 w696 w697] -> w689
                    frame 0, Default {
                      n614 = global read "全局 所有参数.vi" "氨氮"() -> (w693:string[][])
                    }
                    frame 1 {
                      n615 = global read "全局 所有参数.vi" "总氮"() -> (w694:string[][])
                    }
                    frame 2 {
                      n616 = global read "全局 所有参数.vi" "总磷"() -> (w695:string[][])
                    }
                    frame 3 {
                      n617 = global read "全局 所有参数.vi" "CODMn"() -> (w696:string[][])
                    }
                    frame 4 {
                      n618 = global read "全局 所有参数.vi" "CODCr"() -> (w697:string[][])
                    }
                  }
                  n619 = Array Size(array=w689) -> (size(s)=w691:i32[])
                  n620 = Index Array(array=w691) -> (element=w690:i32)  [unwired: 1 in]
                  n621 = Greater Than 0?(x=w690) -> (x > 0?=w692:bool)
                  n622 = case shown="真" w692 {
                    tunnel: w688 -> [_ w703]
                    tunnel: w690 -> [_ _]
                    tunnel: w689 -> [_ w701]
                    frame False {
                    }
                    frame True {
                      # "最新时间戳加1分钟"
                      n623 = Index Array(array=w701, index (row)=0 ("禁用的索引 (行)"), index (col)=0 ("禁用的索引 (列)")) -> (element=w700:string)
                      n624 = call "日期时间字符串转换分钟数加一.vi"("data[0]"=w700) -> ("日期/时间字符串"=w699:string)  [unwired: 10 in]
                      n625 = case shown="0, 默认" w703 {
                        tunnel: w699 -> [w704 w705 w706 w707 w708]
                        frame 0, Default {
                          n626 = global write "全局 时间2.vi" "氨氮仪器参数索引起始时间"(w704) -> ()
                        }
                        frame 1 {
                          n627 = global write "全局 时间2.vi" "总氮仪器参数索引起始时间"(w705) -> ()
                        }
                        frame 2 {
                          n628 = global write "全局 时间2.vi" "总磷仪器参数索引起始时间"(w706) -> ()
                        }
                        frame 3 {
                          n629 = global write "全局 时间2.vi" "CODMn仪器参数索引起始时间"(w707) -> ()
                        }
                        frame 4 {
                          n630 = global write "全局 时间2.vi" "CODCr仪器参数索引起始时间"(w708) -> ()
                        }
                      }
                    }
                  }
                }
              }
              frame #3 {
                n631 = call <vilib>:"Application Directory.vi"() -> ("Application Directory"=w722:path)
                n632 = call "数据处理整合 (子VI).vi"("枚举"=enum16{"实时数据排序", "小时数据排序"}."实时数据排序") -> ("已排序的数组"=w725:string[])  [unwired: 10 in]
                n633 = Build Path(base path=w722, name or relative path="data\\hecha.ini" ("名称或相对路径")) -> (appended path=w720:path)
                n634 = Array Size(array=w725) -> (size(s)=w724:i32)
                n635 = call <vilib>:"Open Config Data.vi"("configuration file path"=w720) -> ("error out"=w716:errorcluster, "refnum"=w719:T8)  [unwired: 8 in, 1 out]
                n636 = vi-ref "全局 时间2.vi"() -> (w718:refnum<vi>)
                n637 = global write "全局 数据数组大小.vi" "数据数组大小"(w724) -> ()
                n638 = call <userlib>:"Write Panel to INI__ogtk.vi"("error in (no error)"=w716, "VI ref"=w718, "refnum"=w719) -> ("error out"=w715:errorcluster, "refnum out"=w717:T8)  [unwired: 7 in]
                n639 = call <vilib>:"Close Config Data.vi"("error in (no error)"=w715, "refnum"=w717) -> ("error out"=w710:errorcluster, "file path"=w709:path)  [unwired: 8 in]
                n640 = Open/Create/Replace File(file path (use dialog)=w709, error in=w710) -> (refnum out=w713:refnum<file>, error out=w714:errorcluster)  [unwired: 4 in, 1 out]
                n641 = Flush File(refnum=w713, error in=w714) -> (refnum out=w712:refnum<file>, error out=w711:errorcluster)
                n642 = Close File(refnum=w712, error in=w711) -> ()  [unwired: 2 out]
              }
              frame #4 {
                n643 = while {
                  stop <- w726 stop-if-true
                  # "判定是否存表"
                  n644 = property on="TCP服务端掉线计数" class="DigNum (严格)"() -> ("Value"=w732:i32)  [unwired: 2 in, 2 out]
                  n645 = Greater Or Equal?(x=w732, y=1) -> (x >= y?=w731:bool)
                  n646 = case shown="假" w731 {
                    frame False {
                      n647 = global read "全局 数据数组大小.vi" "数据数组大小"() -> (w734:i32)
                      n648 = Greater Than 0?(x=w734) -> (x > 0?=w735:bool)
                      n649 = case shown="真" w735 {
                        frame False {
                        }
                        frame True {
                          n650 = global read "全局 小时数据发送次数.vi" "小时数据发送次数"() -> (w744:i32)
                          n651 = local write "核查数据上传"(TRUE ("数据上传")) -> ()
                          n652 = Get Date/Time In Seconds() -> (seconds since 1Jan1904=w749:timestamp)
                          n653 = Increment(x=w744) -> (x+1=w743:i32)
                          n654 = Format Date/Time String(time format string (%c)="%Y%m%d%H%M%S%3u" ("时间格式字符串(%c)"), seconds (now)=w749) -> (date/time string=w748:string)  [unwired: 1 in]
                          n655 = global write "全局 小时数据发送次数.vi" "小时数据发送次数"(w743) -> ()
                          n656 = Search and Replace String(input string=w748, search string="." ("搜索字符串")) -> (result string=w746:string)  [unwired: 6 in, 3 out]
                          n657 = local read "MN"() -> (w741:string)
                          n658 = local read "PW"() -> (w740:string)
                          n659 = call "数据编码.vi"("table输入"="仪器参数" ("新元素/子数组"), "QN"=w746, "MN"=w741, "PW"=w740) -> ("通讯包字符串"=w737:string)  [unwired: 10 in, 1 out]
                          n660 = local read "数据发送通道"() -> (w739:enum16{"TCP", "VISA"})
                          n661 = local write "发送报文显示"(w737) -> ()
                          n662 = call "VISATCP组合选择发送.vi"("数据发送通道"=w739, "命令"="write", "写入缓冲区"=w737) -> ("错误输出"=w736:errorcluster)  [unwired: 9 in, 3 out]
                          n663 = Build Array(w737) -> (w745:string[])
                          n664 = local write "错误输出"(w736) -> ()
                          n665 = call "发送数据记录到文档(子VI).vi"("数组"=w745) -> ()  [unwired: 9 in, 1 out]
                        }
                      }
                    }
                    frame True {
                    }
                  }
                  n666 = Wait (ms)(milliseconds to wait=u32 500 ("等待时间（毫秒）")) -> ()  [unwired: 1 out]
                  n667 = global read "全局 数据数组大小.vi" "数据数组大小"() -> (w728:i32)
                  n668 = global read "全局 小时数据发送次数.vi" "小时数据发送次数"() -> (w730:i32)
                  n669 = Decrement(x=w728) -> (x-1=w727:i32)
                  n670 = Greater Or Equal?(x=w730, y=w727) -> (x >= y?=w726:bool)
                }
              }
            }
          }
          frame "系统状态" {
            # "直接1分钟查询 一次,有变化就按上传,没变化就不上传"
            n671 = flat-sequence {
              frame #0 {
                # "时间"
                n672 = global write "全局 小时数据发送次数.vi" "小时数据发送次数"(0 ("小时数据发送次数")) -> ()
                n673 = global write "全局 数据数组大小.vi" "数据数组大小"(1 ("数据数组大小")) -> ()
                n674 = global write "全局1.vi" "枚举"(enum16{"返回请求应答", "上传数据", "返回执行结果"}."上传数据" ("枚举")) -> ()
              }
              frame #1 {
                # "判定是否存表"
                n675 = property on="TCP服务端掉线计数" class="DigNum (严格)"() -> ("Value"=w756:i32)  [unwired: 2 in, 2 out]
                n676 = Greater Or Equal?(x=w756, y=1) -> (x >= y?=w755:bool)
                n677 = case shown="假" w755 {
                  frame False {
                    n678 = global read "全局 数据数组大小.vi" "数据数组大小"() -> (w758:i32)
                    n679 = Greater Than 0?(x=w758) -> (x > 0?=w759:bool)
                    n680 = case shown="真" w759 {
                      frame False {
                      }
                      frame True {
                        n681 = global read "全局 小时数据发送次数.vi" "小时数据发送次数"() -> (w768:i32)
                        n682 = local write "核查数据上传"(TRUE ("数据上传")) -> ()
                        n683 = Get Date/Time In Seconds() -> (seconds since 1Jan1904=w773:timestamp)
                        n684 = Increment(x=w768) -> (x+1=w767:i32)
                        n685 = Format Date/Time String(time format string (%c)="%Y%m%d%H%M%S%3u" ("时间格式字符串(%c)"), seconds (now)=w773) -> (date/time string=w772:string)  [unwired: 1 in]
                        n686 = global write "全局 小时数据发送次数.vi" "小时数据发送次数"(w767) -> ()
                        n687 = Search and Replace String(input string=w772, search string="." ("搜索字符串")) -> (result string=w770:string)  [unwired: 6 in, 3 out]
                        n688 = local read "MN"() -> (w765:string)
                        n689 = local read "PW"() -> (w764:string)
                        n690 = call "数据编码.vi"("table输入"="系统状态" ("新元素/子数组"), "QN"=w770, "MN"=w765, "PW"=w764) -> ("通讯包字符串"=w761:string)  [unwired: 10 in, 1 out]
                        n691 = local read "数据发送通道"() -> (w763:enum16{"TCP", "VISA"})
                        n692 = local write "发送报文显示"(w761) -> ()
                        n693 = call "VISATCP组合选择发送.vi"("数据发送通道"=w763, "命令"="write", "写入缓冲区"=w761) -> ("错误输出"=w760:errorcluster)  [unwired: 9 in, 3 out]
                        n694 = Build Array(w761) -> (w769:string[])
                        n695 = local write "错误输出"(w760) -> ()
                        n696 = call "发送数据记录到文档(子VI).vi"("数组"=w769) -> ()  [unwired: 9 in, 1 out]
                      }
                    }
                  }
                  frame True {
                  }
                }
              }
            }
          }
          frame "运行模式" {
            # "直接1分钟查询 一次,有变化就按上传,没变化就不上传"
            n697 = flat-sequence {
              frame #0 {
                # "时间"
                n698 = global write "全局 小时数据发送次数.vi" "小时数据发送次数"(0 ("小时数据发送次数")) -> ()
                n699 = global write "全局 数据数组大小.vi" "数据数组大小"(1 ("数据数组大小")) -> ()
                n700 = global write "全局1.vi" "枚举"(enum16{"返回请求应答", "上传数据", "返回执行结果"}."上传数据" ("枚举")) -> ()
              }
              frame #1 {
                # "判定是否存表"
                n701 = property on="TCP服务端掉线计数" class="DigNum (严格)"() -> ("Value"=w780:i32)  [unwired: 2 in, 2 out]
                n702 = Greater Or Equal?(x=w780, y=1) -> (x >= y?=w779:bool)
                n703 = case shown="假" w779 {
                  frame False {
                    n704 = global read "全局 数据数组大小.vi" "数据数组大小"() -> (w782:i32)
                    n705 = Greater Than 0?(x=w782) -> (x > 0?=w783:bool)
                    n706 = case shown="真" w783 {
                      frame False {
                      }
                      frame True {
                        n707 = global read "全局 小时数据发送次数.vi" "小时数据发送次数"() -> (w792:i32)
                        n708 = local write "核查数据上传"(TRUE ("数据上传")) -> ()
                        n709 = Get Date/Time In Seconds() -> (seconds since 1Jan1904=w797:timestamp)
                        n710 = Increment(x=w792) -> (x+1=w791:i32)
                        n711 = Format Date/Time String(time format string (%c)="%Y%m%d%H%M%S%3u" ("时间格式字符串(%c)"), seconds (now)=w797) -> (date/time string=w796:string)  [unwired: 1 in]
                        n712 = global write "全局 小时数据发送次数.vi" "小时数据发送次数"(w791) -> ()
                        n713 = Search and Replace String(input string=w796, search string="." ("搜索字符串")) -> (result string=w794:string)  [unwired: 6 in, 3 out]
                        n714 = local read "MN"() -> (w788:string)
                        n715 = local read "PW"() -> (w789:string)
                        n716 = local read "数据发送通道"() -> (w787:enum16{"TCP", "VISA"})
                        n717 = call "数据编码.vi"("table输入"="运行模式" ("新元素/子数组"), "QN"=w794, "MN"=w788, "PW"=w789) -> ("通讯包字符串"=w784:string)  [unwired: 10 in, 1 out]
                        n718 = local write "发送报文显示"(w784) -> ()
                        n719 = call "VISATCP组合选择发送.vi"("数据发送通道"=w787, "命令"="write", "写入缓冲区"=w784) -> ("错误输出"=w785:errorcluster)  [unwired: 9 in, 3 out]
                        n720 = Build Array(w784) -> (w793:string[])
                        n721 = local write "错误输出"(w785) -> ()
                        n722 = call "发送数据记录到文档(子VI).vi"("数组"=w793) -> ()  [unwired: 9 in, 1 out]
                      }
                    }
                  }
                  frame True {
                  }
                }
              }
            }
          }
          frame "测量周期" {
            # "直接1分钟查询 一次,有变化就按上传,没变化就不上传"
            n723 = flat-sequence {
              frame #0 {
                # "时间"
                n724 = global write "全局 小时数据发送次数.vi" "小时数据发送次数"(0 ("小时数据发送次数")) -> ()
                n725 = global write "全局 数据数组大小.vi" "数据数组大小"(1 ("数据数组大小")) -> ()
                n726 = global write "全局1.vi" "枚举"(enum16{"返回请求应答", "上传数据", "返回执行结果"}."上传数据" ("枚举")) -> ()
              }
              frame #1 {
                # "判定是否存表"
                n727 = property on="TCP服务端掉线计数" class="DigNum (严格)"() -> ("Value"=w804:i32)  [unwired: 2 in, 2 out]
                n728 = Greater Or Equal?(x=w804, y=1) -> (x >= y?=w803:bool)
                n729 = case shown="假" w803 {
                  frame False {
                    n730 = global read "全局 数据数组大小.vi" "数据数组大小"() -> (w806:i32)
                    n731 = Greater Than 0?(x=w806) -> (x > 0?=w807:bool)
                    n732 = case shown="真" w807 {
                      frame False {
                      }
                      frame True {
                        n733 = global read "全局 小时数据发送次数.vi" "小时数据发送次数"() -> (w816:i32)
                        n734 = local write "核查数据上传"(TRUE ("数据上传")) -> ()
                        n735 = Get Date/Time In Seconds() -> (seconds since 1Jan1904=w821:timestamp)
                        n736 = Increment(x=w816) -> (x+1=w815:i32)
                        n737 = Format Date/Time String(time format string (%c)="%Y%m%d%H%M%S%3u" ("时间格式字符串(%c)"), seconds (now)=w821) -> (date/time string=w820:string)  [unwired: 1 in]
                        n738 = global write "全局 小时数据发送次数.vi" "小时数据发送次数"(w815) -> ()
                        n739 = Search and Replace String(input string=w820, search string="." ("搜索字符串")) -> (result string=w818:string)  [unwired: 6 in, 3 out]
                        n740 = local read "MN"() -> (w813:string)
                        n741 = local read "PW"() -> (w812:string)
                        n742 = call "数据编码.vi"("table输入"="测量周期" ("新元素/子数组"), "QN"=w818, "MN"=w813, "PW"=w812) -> ("通讯包字符串"=w809:string)  [unwired: 10 in, 1 out]
                        n743 = local read "数据发送通道"() -> (w811:enum16{"TCP", "VISA"})
                        n744 = local write "发送报文显示"(w809) -> ()
                        n745 = call "VISATCP组合选择发送.vi"("数据发送通道"=w811, "命令"="write", "写入缓冲区"=w809) -> ("错误输出"=w808:errorcluster)  [unwired: 9 in, 3 out]
                        n746 = Build Array(w809) -> (w817:string[])
                        n747 = local write "错误输出"(w808) -> ()
                        n748 = call "发送数据记录到文档(子VI).vi"("数组"=w817) -> ()  [unwired: 9 in, 1 out]
                      }
                    }
                  }
                  frame True {
                  }
                }
              }
            }
          }
          frame "超标留样" {
            # "直接1分钟查询 一次,有变化就按上传,没变化就不上传"
            n749 = flat-sequence {
              frame #0 {
                # "时间"
                n750 = global write "全局 小时数据发送次数.vi" "小时数据发送次数"(0 ("小时数据发送次数")) -> ()
                n751 = global write "全局 数据数组大小.vi" "数据数组大小"(1 ("数据数组大小")) -> ()
                n752 = global write "全局1.vi" "枚举"(enum16{"返回请求应答", "上传数据", "返回执行结果"}."上传数据" ("枚举")) -> ()
              }
              frame #1 {
                # "判定是否存表"
                n753 = property on="TCP服务端掉线计数" class="DigNum (严格)"() -> ("Value"=w828:i32)  [unwired: 2 in, 2 out]
                n754 = Greater Or Equal?(x=w828, y=1) -> (x >= y?=w827:bool)
                n755 = case shown="假" w827 {
                  frame False {
                    n756 = global read "全局 数据数组大小.vi" "数据数组大小"() -> (w830:i32)
                    n757 = Greater Than 0?(x=w830) -> (x > 0?=w831:bool)
                    n758 = case shown="真" w831 {
                      frame False {
                      }
                      frame True {
                        n759 = global read "全局 小时数据发送次数.vi" "小时数据发送次数"() -> (w840:i32)
                        n760 = local write "核查数据上传"(TRUE ("数据上传")) -> ()
                        n761 = Get Date/Time In Seconds() -> (seconds since 1Jan1904=w845:timestamp)
                        n762 = Increment(x=w840) -> (x+1=w839:i32)
                        n763 = Format Date/Time String(time format string (%c)="%Y%m%d%H%M%S%3u" ("时间格式字符串(%c)"), seconds (now)=w845) -> (date/time string=w844:string)  [unwired: 1 in]
                        n764 = global write "全局 小时数据发送次数.vi" "小时数据发送次数"(w839) -> ()
                        n765 = Search and Replace String(input string=w844, search string="." ("搜索字符串")) -> (result string=w842:string)  [unwired: 6 in, 3 out]
                        n766 = local read "MN"() -> (w837:string)
                        n767 = local read "PW"() -> (w836:string)
                        n768 = call "数据编码.vi"("table输入"="超标留样" ("新元素/子数组"), "QN"=w842, "MN"=w837, "PW"=w836) -> ("通讯包字符串"=w833:string)  [unwired: 10 in, 1 out]
                        n769 = local read "数据发送通道"() -> (w835:enum16{"TCP", "VISA"})
                        n770 = local write "发送报文显示"(w833) -> ()
                        n771 = call "VISATCP组合选择发送.vi"("数据发送通道"=w835, "命令"="write", "写入缓冲区"=w833) -> ("错误输出"=w832:errorcluster)  [unwired: 9 in, 3 out]
                        n772 = Build Array(w833) -> (w841:string[])
                        n773 = local write "错误输出"(w832) -> ()
                        n774 = call "发送数据记录到文档(子VI).vi"("数组"=w841) -> ()  [unwired: 9 in, 1 out]
                      }
                    }
                  }
                  frame True {
                  }
                }
              }
            }
          }
          frame "报警信息" {
            # "间隔时间上传"
            # "直接1分钟查询 一次,有数据就按数据上传,没数据为空的不传,在数据发送那边有做处理"
            n775 = flat-sequence {
              frame #0 {
                # "分钟时间间隔"
                n776 = global read "全局 数据发送重叠.vi" "数据发送重叠开始时间戳"() -> (w849:string)
                n777 = global read "全局 数据发送重叠.vi" "数据发送重叠"() -> (w848:bool)
                n778 = global write "全局 小时数据发送次数.vi" "小时数据发送次数"(0 ("小时数据发送次数")) -> ()
                n779 = global write "全局1.vi" "枚举"(enum16{"返回请求应答", "上传数据", "返回执行结果"}."上传数据" ("枚举")) -> ()
                n780 = call "日志信息主动发送(子VI).vi"("是否正在查询数据"=w848, "查询数据发送时间节点"=w849) -> ()  [unwired: 10 in]
              }
              frame #1 {
                n781 = call "获取报警信息 (子VI).vi"() -> ()  [unwired: 12 in]
              }
              frame #2 {
                n782 = call "数据处理整合 (子VI).vi"("枚举"=enum16{"实时数据排序", "小时数据排序"}."实时数据排序") -> ("已排序的数组"=w854:string[])  [unwired: 10 in]
                n783 = Array Size(array=w854) -> (size(s)=w853:i32)
                n784 = global write "全局 数据数组大小.vi" "数据数组大小"(w853) -> ()
              }
              frame #3 {
                n785 = while {
                  stop <- w855 stop-if-true
                  # "判定是否存表"
                  n786 = property on="TCP服务端掉线计数" class="DigNum (严格)"() -> ("Value"=w861:i32)  [unwired: 2 in, 2 out]
                  n787 = Greater Or Equal?(x=w861, y=1) -> (x >= y?=w860:bool)
                  n788 = case shown="假" w860 {
                    frame False {
                      # "判定数据不为空才发"
                      n789 = global read "全局 数据数组大小.vi" "数据数组大小"() -> (w863:i32)
                      n790 = Greater Than 0?(x=w863) -> (x > 0?=w864:bool)
                      n791 = case shown="真" w864 {
                        frame False {
                          n792 = local write "核查数据上传"(FALSE ("数据上传")) -> ()
                        }
                        frame True {
                          n793 = global read "全局 小时数据发送次数.vi" "小时数据发送次数"() -> (w873:i32)
                          n794 = Get Date/Time In Seconds() -> (seconds since 1Jan1904=w878:timestamp)
                          n795 = Increment(x=w873) -> (x+1=w872:i32)
                          n796 = Format Date/Time String(time format string (%c)="%Y%m%d%H%M%S%3u" ("时间格式字符串(%c)"), seconds (now)=w878) -> (date/time string=w877:string)  [unwired: 1 in]
                          n797 = global write "全局 小时数据发送次数.vi" "小时数据发送次数"(w872) -> ()
                          n798 = Search and Replace String(input string=w877, search string="." ("搜索字符串")) -> (result string=w875:string)  [unwired: 6 in, 3 out]
                          n799 = local read "MN"() -> (w871:string)
                          n800 = local read "PW"() -> (w870:string)
                          n801 = local read "数据发送通道"() -> (w869:enum16{"TCP", "VISA"})
                          n802 = call "数据编码.vi"("table输入"="报警信息" ("新元素/子数组"), "QN"=w875, "MN"=w871, "PW"=w870) -> ("通讯包字符串"=w867:string)  [unwired: 10 in, 1 out]
                          n803 = local write "发送报文显示"(w867) -> ()
                          n804 = Build Array(w867) -> (w874:string[])
                          n805 = call "VISATCP组合选择发送.vi"("数据发送通道"=w869, "命令"="write", "写入缓冲区"=w867) -> ("错误输出"=w866:errorcluster)  [unwired: 9 in, 3 out]
                          n806 = local write "错误输出"(w866) -> ()
                          n807 = call "发送数据记录到文档(子VI).vi"("数组"=w874) -> ()  [unwired: 9 in, 1 out]
                        }
                      }
                    }
                    frame True {
                    }
                  }
                  n808 = Wait (ms)(milliseconds to wait=u32 500 ("等待时间（毫秒）")) -> ()  [unwired: 1 out]
                  n809 = global read "全局 数据数组大小.vi" "数据数组大小"() -> (w857:i32)
                  n810 = global read "全局 小时数据发送次数.vi" "小时数据发送次数"() -> (w859:i32)
                  n811 = Decrement(x=w857) -> (x-1=w856:i32)
                  n812 = Greater Or Equal?(x=w859, y=w856) -> (x >= y?=w855:bool)
                }
              }
            }
          }
          frame "环境参数" {
            # "间隔时间上传"
            # "直接1分钟查询 一次,有数据就按数据上传,没数据为空的不传,在数据发送那边有做处理"
            n813 = disable-structure shown="禁用" {
              frame Disabled {
                n814 = flat-sequence {
                  frame #0 {
                    # "分钟时间间隔"
                    n815 = global read "全局 数据发送重叠.vi" "数据发送重叠开始时间戳"() -> (w882:string)
                    n816 = global read "全局 数据发送重叠.vi" "数据发送重叠"() -> (w881:bool)
                    n817 = global write "全局 小时数据发送次数.vi" "小时数据发送次数"(0 ("小时数据发送次数")) -> ()
                    n818 = global write "全局1.vi" "枚举"(enum16{"返回请求应答", "上传数据", "返回执行结果"}."上传数据" ("枚举")) -> ()
                    n819 = call "日志信息主动发送(子VI).vi"("是否正在查询数据"=w881, "查询数据发送时间节点"=w882) -> ()  [unwired: 10 in]
                  }
                  frame #1 {
                    n820 = call "获取环境参数 (子VI).vi"() -> ()  [unwired: 12 in]
                  }
                  frame #2 {
                    n821 = call "数据处理整合 (子VI).vi"("枚举"=enum16{"实时数据排序", "小时数据排序"}."实时数据排序") -> ("已排序的数组"=w887:string[])  [unwired: 10 in]
                    n822 = Array Size(array=w887) -> (size(s)=w886:i32)
                    n823 = global write "全局 数据数组大小.vi" "数据数组大小"(w886) -> ()
                  }
                  frame #3 {
                    n824 = while {
                      stop <- w888 stop-if-true
                      # "判定是否存表"
                      n825 = property on="TCP服务端掉线计数" class="DigNum (严格)"() -> ("Value"=w894:i32)  [unwired: 2 in, 2 out]
                      n826 = Greater Or Equal?(x=w894, y=1) -> (x >= y?=w893:bool)
                      n827 = case shown="假" w893 {
                        frame False {
                          # "判定数据不为空才发"
                          n828 = global read "全局 数据数组大小.vi" "数据数组大小"() -> (w896:i32)
                          n829 = Greater Than 0?(x=w896) -> (x > 0?=w897:bool)
                          n830 = case shown="真" w897 {
                            frame False {
                            }
                            frame True {
                              n831 = global read "全局 小时数据发送次数.vi" "小时数据发送次数"() -> (w904:i32)
                              n832 = local write "核查数据上传"(TRUE ("数据上传")) -> ()
                              n833 = Get Date/Time In Seconds() -> (seconds since 1Jan1904=w909:timestamp)
                              n834 = Increment(x=w904) -> (x+1=w903:i32)
                              n835 = Format Date/Time String(time format string (%c)="%Y%m%d%H%M%S%3u" ("时间格式字符串(%c)"), seconds (now)=w909) -> (date/time string=w908:string)  [unwired: 1 in]
                              n836 = global write "全局 小时数据发送次数.vi" "小时数据发送次数"(w903) -> ()
                              n837 = Search and Replace String(input string=w908, search string="." ("搜索字符串")) -> (result string=w906:string)  [unwired: 6 in, 3 out]
                              n838 = local read "MN"() -> (w912:string)
                              n839 = local read "PW"() -> (w911:string)
                              n840 = local read "数据发送通道"() -> (w900:enum16{"TCP", "VISA"})
                              n841 = call "数据编码.vi"("table输入"="报警信息" ("新元素/子数组"), "QN"=w906, "MN"=w912, "PW"=w911) -> ("通讯包字符串"=w899:string)  [unwired: 10 in, 1 out]
                              n842 = local write "发送报文显示"(w899) -> ()
                              n843 = call "VISATCP组合选择发送.vi"("数据发送通道"=w900, "命令"="write", "写入缓冲区"=w899) -> ("错误输出"=w898:errorcluster)  [unwired: 9 in, 3 out]
                              n844 = Build Array(w899) -> (w905:string[])
                              n845 = local write "错误输出"(w898) -> ()
                              n846 = call "发送数据记录到文档(子VI).vi"("数组"=w905) -> ()  [unwired: 9 in, 1 out]
                            }
                          }
                        }
                        frame True {
                        }
                      }
                      n847 = Wait (ms)(milliseconds to wait=u32 500 ("等待时间（毫秒）")) -> ()  [unwired: 1 out]
                      n848 = global read "全局 数据数组大小.vi" "数据数组大小"() -> (w890:i32)
                      n849 = global read "全局 小时数据发送次数.vi" "小时数据发送次数"() -> (w892:i32)
                      n850 = Decrement(x=w890) -> (x-1=w889:i32)
                      n851 = Greater Or Equal?(x=w892, y=w889) -> (x >= y?=w888:bool)
                    }
                  }
                }
              }
              frame Enabled {
              }
            }
          }
        }
      }
    }
  }
  n852 = while {
    tunnel: w38 -> [w917]
    stop <- FALSE stop-if-true
    # "和工控机通讯系统状态改变主动上传"
    # "整点发送小时数据(禁用）运行模式运行周期"
    n853 = Multiply(x=u32 1, y=u32 1000 ("等待时间（毫秒）")) -> (x*y=w923:u32)
    n854 = case shown="真" "每周自动重发" {
      frame False {
      }
      frame True {
        (unwired) T1."00点"
        (unwired) T2."关闭"
        # "自动重发水样数据"
        n855 = Get Date/Time In Seconds() -> (seconds since 1Jan1904=w988:timestamp)
        n856 = Seconds To Date/Time(time stamp (now)=w988) -> (date time rec=w982:T9)  [unwired: 1 in]
        n857 = Unbundle By Name(w982) -> ("天数（周）"=w987:i32, "时"=w977:i32, "分"=w986:i32)
        n858 = Equal To 0?(x=w986) -> (x = 0?=w983:bool)
        n859 = Equal?(x=w987, y="重发日期") -> (x = y?=w985:bool)
        n860 = Equal?(x=w977, y="重发时间") -> (x = y?=w984:bool)
        n861 = Compound Arithmetic op=AND ("复合运算")(w985, w984, w983) -> (w981:bool)
        n862 = call <vilib>:"Boolean Crossing PtByPt.vi"("direction"=enum16{"either", "false-true", "true-false"}."false-true", "input"=w981) -> ("crossing"=w980:bool)  [unwired: 1 in]
        n863 = case shown="真" w980 {
          tunnel: w982 -> [_ w990]
          frame False {
          }
          frame True {
            n864 = local read "参数数值"() -> (w995:T5)
            n865 = Unbundle By Name(w990) -> ("日"=w993:i32)
            n866 = Cluster To Array(cluster=w995) -> (array=w996:bool[])
            n867 = Subtract(x=w993, y=7) -> (x-y=w991:i32)
            n868 = Bundle By Name(cluster=w990, "日"=w991) -> (w994:T9)
            n869 = Date/Time To Seconds(2:w994) -> (0:w989:timestamp)  [unwired: 1 in]
            n870 = for {
              tunnel: w996 -> [_] mode=indexing
              tunnel: w989 -> [w997]
              i -> [w998]
              n871 = Format Date/Time String(time format string (%c)="%Y/%m/%d %H:%M:%S" ("时间格式字符串(%c)"), seconds (now)=w997) -> (date/time string=w999:string)  [unwired: 1 in]
              n872 = case shown="16" w998 {
                tunnel: w999 -> [w1001 w1002 w1003 w1004 w1005 w1006 w1007 w1008 w1009 w1010 w1011 w1012 w1013 w1014 w1015 w1016 w1017 w1018]
                frame 0, Default {
                  n873 = global write "全局 水样时间.vi" "time1"(w1001) -> ()
                }
                frame 1 {
                  n874 = global write "全局 水样时间.vi" "time2"(w1002) -> ()
                }
                frame 2 {
                  n875 = global write "全局 水样时间.vi" "time3"(w1003) -> ()
                }
                frame 3 {
                  n876 = global write "全局 水样时间.vi" "time4"(w1004) -> ()
                }
                frame 4 {
                  n877 = global write "全局 水样时间.vi" "time5"(w1005) -> ()
                }
                frame 5 {
                  n878 = global write "全局 水样时间.vi" "time6"(w1006) -> ()
                }
                frame 6 {
                  n879 = global write "全局 水样时间.vi" "time7"(w1007) -> ()
                }
                frame 7 {
                  n880 = global write "全局 水样时间.vi" "time8"(w1008) -> ()
                }
                frame 8 {
                  n881 = global write "全局 水样时间.vi" "time9"(w1009) -> ()
                }
                frame 9 {
                  n882 = global write "全局 水样时间.vi" "time10"(w1010) -> ()
                }
                frame 10 {
                  n883 = global write "全局 水样时间.vi" "time11"(w1011) -> ()
                }
                frame 11 {
                  n884 = global write "全局 水样时间.vi" "time12"(w1012) -> ()
                }
                frame 12 {
                  n885 = global write "全局 水样时间.vi" "time13"(w1013) -> ()
                }
                frame 13 {
                  n886 = global write "全局 水样时间.vi" "time14"(w1014) -> ()
                }
                frame 14 {
                  n887 = global write "全局 水样时间.vi" "time15"(w1015) -> ()
                }
                frame 15 {
                  n888 = global write "全局 水样时间.vi" "time16"(w1016) -> ()
                }
                frame 16 {
                  n889 = global write "全局 水样时间.vi" "time17"(w1017) -> ()
                }
                frame 17 {
                  n890 = global write "全局 水样时间.vi" "time18"(w1018) -> ()
                }
              }
            }
          }
        }
      }
    }
    n891 = Wait (ms)(milliseconds to wait=w923) -> ()  [unwired: 1 out]
    n892 = First Call?() -> (First Call?: T/F=w914:bool)
    n893 = case shown="假" w914 {
      tunnel: ["读取" ("读取写入选择") "打开" ("读取写入选择")] -> w920
      frame False {
      }
      frame True {
      }
    }
    n894 = call "Modbus Master.vi"("Unit ID"=u8 1, "读取写入选择"=w920) -> ("register values"=w918:u16[], "error out"=w915:errorcluster)  [unwired: 8 in]
    n895 = case shown="无错误" w915 {
      tunnel: w918 -> [w929 _]
      tunnel: w917 -> [w927 _]
      frame No Error {
        # "防止由于MBtcp错误导致状态为0发送至平台"
        n896 = global read "全局1.vi" "register values"() -> (w928:u16[])
        n897 = flat-sequence {
          tunnel: w929 -> [w935]
          tunnel: w928 -> [w955]
          tunnel: w927 -> [w931]
          tunnel: [w935] -> w930
          tunnel: w930 -> [w975]
          frame #0 {
            n898 = Index Array(array=w935) -> (element #1=w942:u16, element #2=w954:u16, element #3=w953:u16, element #4=w952:u16, element #5=w951:u16, element #6=w950:u16, element #7=w940:u16, element #8=w934:u16)  [unwired: 8 in]
            n899 = Index Array(array=w955) -> (element #1=w941:u16, element #2=w949:u16, element #3=w948:u16, element #4=w947:u16, element #5=w946:u16, element #6=w945:u16, element #7=w939:u16, element #8=w933:u16)  [unwired: 8 in]
            n900 = Build Array(w954, w953, w952, w951, w950) -> (w944:u16[])
            n901 = Build Array(w949, w948, w947, w946, w945) -> (w943:u16[])
            n902 = Not Equal?(x=w942, y=w941) -> (x != y?=w937:bool)
            n903 = Not Equal?(x=w940, y=w939) -> (x != y?=w938:bool)
            n904 = Not Equal?(x=w934, y=w933) -> (x != y?=w932:bool)
            n905 = Not Equal?(x=w944, y=w943) -> (x != y?=w936:bool[])
            n906 = while {
              tunnel: w931 -> [w964]
              tunnel: w936 -> [w961] mode=indexing
              i -> [w963]
              stop <- w959 stop-if-true
              n907 = Greater Or Equal?(x=w963, y=4) -> (x >= y?=w960:bool)
              n908 = Or(x=w961, y=w960) -> (x .or. y?=w959:bool)
              n909 = case shown="真" w961 {
                tunnel: w964 -> [_ w966]
                frame False {
                }
                frame True {
                  n910 = local write "系统状态改变"(TRUE ("系统状态改变")) -> ()
                  n911 = Enqueue Element(queue=w966, element="系统状态" ("元素")) -> ()  [unwired: 2 in, 3 out]
                }
              }
            }
            n912 = case shown="真" w937 {
              tunnel: w931 -> [_ w972]
              frame False {
              }
              frame True {
                n913 = Enqueue Element(queue=w972, element="运行模式" ("元素")) -> ()  [unwired: 2 in, 3 out]
                "系统状态改变" <- TRUE
              }
            }
            n914 = case shown="真" w932 {
              tunnel: w931 -> [_ w957]
              frame False {
              }
              frame True {
                n915 = local write "系统状态改变"(TRUE ("系统状态改变")) -> ()
                n916 = Enqueue Element(queue=w957, element="超标留样" ("元素")) -> ()  [unwired: 2 in, 3 out]
              }
            }
            n917 = case shown="真" w938 {
              tunnel: w931 -> [_ w969]
              frame False {
              }
              frame True {
                n918 = local write "系统状态改变"(TRUE ("系统状态改变")) -> ()
                n919 = Enqueue Element(queue=w969, element="测量周期" ("元素")) -> ()  [unwired: 2 in, 3 out]
              }
            }
          }
          frame #1 {
            n920 = global write "全局1.vi" "register values"(w975) -> ()
            n921 = local write "系统状态改变"(FALSE ("系统状态改变")) -> ()
          }
        }
      }
      frame Error {
      }
    }
  }
  n922 = while "While循环" {
    tunnel: [w1035] -> _
    tunnel: w32 -> [w1029]
    stop <- FALSE stop-if-true
    w1019 = FALSE ("小时数据上传")
    # "实时、小时数据出数据就上传"
    n923 = property on="TCP服务端掉线计数" class="DigNum (严格)"() -> ("Value"=w1032:i32)  [unwired: 2 in, 2 out]
    n924 = local read "查询数据发送"() -> (w1024:bool)
    n925 = local read "核查数据上传"() -> (w1023:bool)
    n926 = local read "重发数据"() -> (w1025:bool)
    n927 = local read "步骤"() -> (w1034:T6)
    n928 = local write "实时小时数据上传"(w1019) -> ()
    n929 = global write "全局 数据发送重叠.vi" "主动上报数据中"(w1019) -> ()
    n930 = Greater Or Equal?(x=w1029, y=17) -> (x >= y?=w1028:bool)
    n931 = Equal To 0?(x=w1032) -> (x = 0?=w1030:bool)
    n932 = Not(x=w1025) -> (.not. x?=w1022:bool)
    n933 = Not(x=w1024) -> (.not. x?=w1021:bool)
    n934 = Not(x=w1023) -> (.not. x?=w1020:bool)
    n935 = Equal?(x=w1034, y=T6."读取数据" ("步骤")) -> (x = y?=w1031:bool)
    n936 = Wait (ms)(milliseconds to wait=u32 75430 ("等待时间（毫秒）")) -> ()  [unwired: 1 out]
    n937 = Compound Arithmetic op=AND ("复合运算")(w1031, w1030, w1028, w1022, w1021, w1020) -> (w1026:bool)
    n938 = case shown="真" w1026 {
      tunnel: [_ w1040] -> w1035
      frame False {
        w1038 = FALSE ("小时数据上传")
        n939 = local write "实时小时数据上传"(w1038) -> ()
        n940 = global write "全局 数据发送重叠.vi" "主动上报数据中"(w1038) -> ()
      }
      frame True {
        n941 = global read "断电保存全局.vi" "数据组合发送"() -> (w1039:bool)
        n942 = case shown="假" w1039 {
          tunnel: [w1041 _] -> w1040
          frame False {
            # "数据非整点触发，而是实时触发，分条发送"
            n943 = flat-sequence {
              tunnel: [w1045] -> w1042
              tunnel: [w1411] -> w1041
              tunnel: w1042 -> [w1411]
              frame #0 {
                w1043 = TRUE ("小时数据上传")
                n944 = global write "全局 数据发送重叠.vi" "主动上报数据中"(w1043) -> ()
                n945 = local read "数据发送协议"() -> (w1044:enum16{"2005-212协议", "2017-212协议"})
                n946 = case shown="\"2017-212协议\", 默认" w1044 {
                  tunnel: [_ w1181] -> w1045
                  frame "2005-212协议" {
                    n947 = local read "参数数值"() -> (w1049:T5)
                    n948 = Cluster To Array(cluster=w1049) -> (array=w1048:bool[])
                    n949 = for {
                      tunnel: w1048 -> [_] mode=indexing
                      tunnel: [w1093] -> w1047
                      i -> [w1087]
                      w1088 = "1904/01/01 00:00:00"
                      (unwired) " where 时间 between #"
                      w1091 = "database1.mdb" ("database")
                      (unwired) "'and 数据类型 ='N' and 时间 between "
                      w1095 = 0 ("索引 (行)")
                      n950 = case shown="12" w1087 {
                        tunnel: [w1145 w1147 w1149 w1151 w1153 w1155 w1157 w1159 w1161 w1163 w1165 w1167 w1169 w1171 w1173 w1175 w1177 w1179] -> w1090
                        frame 0, Default {
                          n951 = control-ref of="CODMn"() -> (w1146:refnum<vi>)
                          n952 = property class="Bool (严格)"(reference=w1146) -> ("Label.Text"=w1145:string)  [unwired: 1 in, 2 out]
                        }
                        frame 1 {
                          n953 = control-ref of="CODCr"() -> (w1148:refnum<vi>)
                          n954 = property class="Bool (严格)"(reference=w1148) -> ("Label.Text"=w1147:string)  [unwired: 1 in, 2 out]
                        }
                        frame 2 {
                          n955 = control-ref of="DO"() -> (w1150:refnum<vi>)
                          n956 = property class="Bool (严格)"(reference=w1150) -> ("Label.Text"=w1149:string)  [unwired: 1 in, 2 out]
                        }
                        frame 3 {
                          n957 = control-ref of="铜"() -> (w1152:refnum<vi>)
                          n958 = property class="Bool (严格)"(reference=w1152) -> ("Label.Text"=w1151:string)  [unwired: 1 in, 2 out]
                        }
                        frame 4 {
                          n959 = control-ref of="PH"() -> (w1154:refnum<vi>)
                          n960 = property class="Bool (严格)"(reference=w1154) -> ("Label.Text"=w1153:string)  [unwired: 1 in, 2 out]
                        }
                        frame 5 {
                          n961 = control-ref of="氨氮"() -> (w1156:refnum<vi>)
                          n962 = property class="Bool (严格)"(reference=w1156) -> ("Label.Text"=w1155:string)  [unwired: 1 in, 2 out]
                        }
                        frame 6 {
                          n963 = control-ref of="比电导率"() -> (w1158:refnum<vi>)
                          n964 = property class="Bool (严格)"(reference=w1158) -> ("Label.Text"=w1157:string)  [unwired: 1 in, 2 out]
                        }
                        frame 7 {
                          n965 = control-ref of="水温"() -> (w1160:refnum<vi>)
                          n966 = property class="Bool (严格)"(reference=w1160) -> ("Label.Text"=w1159:string)  [unwired: 1 in, 2 out]
                        }
                        frame 8 {
                          n967 = control-ref of="盐度(海水)"() -> (w1162:refnum<vi>)
                          n968 = property class="Bool (严格)"(reference=w1162) -> ("Label.Text"=w1161:string)  [unwired: 1 in, 2 out]
                        }
                        frame 9 {
                          n969 = control-ref of="浊度"() -> (w1164:refnum<vi>)
                          n970 = property class="Bool (严格)"(reference=w1164) -> ("Label.Text"=w1163:string)  [unwired: 1 in, 2 out]
                        }
                        frame 10 {
                          n971 = control-ref of="总氮"() -> (w1166:refnum<vi>)
                          n972 = property class="Bool (严格)"(reference=w1166) -> ("Label.Text"=w1165:string)  [unwired: 1 in, 2 out]
                        }
                        frame 11 {
                          n973 = control-ref of="总磷"() -> (w1168:refnum<vi>)
                          n974 = property class="Bool (严格)"(reference=w1168) -> ("Label.Text"=w1167:string)  [unwired: 1 in, 2 out]
                        }
                        frame 12 {
                          n975 = control-ref of="叶绿素a"() -> (w1170:refnum<vi>)
                          n976 = property class="Bool (严格)"(reference=w1170) -> ("Label.Text"=w1169:string)  [unwired: 1 in, 2 out]
                        }
                        frame 13 {
                          n977 = control-ref of="藻密度"() -> (w1172:refnum<vi>)
                          n978 = property class="Bool (严格)"(reference=w1172) -> ("Label.Text"=w1171:string)  [unwired: 1 in, 2 out]
                        }
                        frame 14 {
                          n979 = control-ref of="水位"() -> (w1174:refnum<vi>)
                          n980 = property class="Bool (严格)"(reference=w1174) -> ("Label.Text"=w1173:string)  [unwired: 1 in, 2 out]
                        }
                        frame 15 {
                          n981 = control-ref of="流速"() -> (w1176:refnum<vi>)
                          n982 = property class="Bool (严格)"(reference=w1176) -> ("Label.Text"=w1175:string)  [unwired: 1 in, 2 out]
                        }
                        frame 16 {
                          n983 = control-ref of="瞬时流量"() -> (w1178:refnum<vi>)
                          n984 = property class="Bool (严格)"(reference=w1178) -> ("Label.Text"=w1177:string)  [unwired: 1 in, 2 out]
                        }
                        frame 17 {
                          n985 = control-ref of="累积流量"() -> (w1180:refnum<vi>)
                          n986 = property class="Bool (严格)"(reference=w1180) -> ("Label.Text"=w1179:string)  [unwired: 1 in, 2 out]
                        }
                      }
                      n987 = Get Date/Time In Seconds() -> (seconds since 1Jan1904=w1099:timestamp)
                      n988 = Format Date/Time String(time format string (%c)="%Y/%m/%d %H:%M:%S" ("时间格式字符串(%c)"), seconds (now)=w1099) -> (date/time string=w1089:string)  [unwired: 1 in]
                      n989 = Format Into String(format string="#%s#" ("初始字符串"), w1088) -> (resulting string=w1097:string)  [unwired: 2 in, 1 out]
                      n990 = Format Into String(format string="#%s#" ("初始字符串"), w1089) -> (resulting string=w1092:string)  [unwired: 2 in, 1 out]
                      n991 = case shown="0, 默认" w1087 {
                        selector: w1087 -> [_ w1131]
                        tunnel: w1097 -> [w1126 w1136]
                        tunnel: [w1125 w1137] -> w1096
                        tunnel: w1092 -> [w1122 w1135]
                        tunnel: w1091 -> [_ w1134]
                        tunnel: w1090 -> [_ w1133]
                        tunnel: w1088 -> [_ w1128]
                        tunnel: w1089 -> [_ w1130]
                        frame 0, Default {
                          n992 = Concatenate Strings("where 测量模式 ='水样测试" ("condition"), "'and 时间 between ", w1126, "and" ("字符串"), w1122, " order by 时间 desc" ("字符串")) -> (w1125:string)
                        }
                        frame 14..17 {
                          n993 = call "流量数据规范小时时间戳.vi"("字符串"=w1128) -> ("result string"=w1127:string)  [unwired: 10 in]
                          n994 = call "database1查询.vi"("时间2"=w1130, "table"=w1133, "时间1"=w1127, "database"=w1134) -> ("error out"=w1129:errorcluster, "data"=w1132:string[][])  [unwired: 4 in, 1 out]
                          n995 = call <vilib>:"Clear Errors.vi"("error in (no error)"=w1129) -> ()  [unwired: 5 in, 2 out]
                          n996 = case shown="14" w1131 {
                            tunnel: w1132 -> [_ w1141 w1142 w1143 w1144]
                            frame 0, Default {
                            }
                            frame 14 {
                              n997 = global write "全局流量数据小时.vi" "水位"(w1141) -> ()
                            }
                            frame 15 {
                              n998 = global write "全局流量数据小时.vi" "流速"(w1142) -> ()
                            }
                            frame 16 {
                              n999 = global write "全局流量数据小时.vi" "瞬时流量"(w1143) -> ()
                            }
                            frame 17 {
                              n1000 = global write "全局流量数据小时.vi" "累积流量"(w1144) -> ()
                            }
                          }
                          n1001 = Concatenate Strings(" where 时间 between ", w1136, "and" ("字符串"), w1135, " order by 时间 desc" ("字符串")) -> (w1137:string)
                        }
                      }
                      n1002 = call "SQL查询.vi"("condition"=w1096, "table输入"=w1090, "database"=w1091) -> ("error out"=w1093:errorcluster, "data"=w1086:string[][])  [unwired: 7 in]
                      n1003 = call "短日期时间转长日期格式.vi"("data"=w1086) -> ("输出数组"=w1094:string[][])  [unwired: 10 in]
                      n1004 = case shown="3" w1087 {
                        tunnel: w1086 -> [w1102 w1103 w1104 w1105 w1106 w1107 w1108 w1109 w1110 w1111 w1112 w1113 w1114 w1115 w1116 w1117 w1118 w1119]
                        frame 0, Default {
                          n1005 = global write "全局 所有参数.vi" "CODMn"(w1102) -> ()
                        }
                        frame 1 {
                          n1006 = global write "全局 所有参数.vi" "CODCr"(w1103) -> ()
                        }
                        frame 2 {
                          n1007 = global write "全局 所有参数.vi" "DO"(w1104) -> ()
                        }
                        frame 3 {
                          n1008 = global write "全局 所有参数.vi" "铜"(w1105) -> ()
                        }
                        frame 4 {
                          n1009 = global write "全局 所有参数.vi" "PH"(w1106) -> ()
                        }
                        frame 5 {
                          n1010 = global write "全局 所有参数.vi" "氨氮"(w1107) -> ()
                        }
                        frame 6 {
                          n1011 = global write "全局 所有参数.vi" "电导率"(w1108) -> ()
                        }
                        frame 7 {
                          n1012 = global write "全局 所有参数.vi" "水温"(w1109) -> ()
                        }
                        frame 8 {
                          n1013 = global write "全局 所有参数.vi" "盐度"(w1110) -> ()
                        }
                        frame 9 {
                          n1014 = global write "全局 所有参数.vi" "浊度"(w1111) -> ()
                        }
                        frame 10 {
                          n1015 = global write "全局 所有参数.vi" "总氮"(w1112) -> ()
                        }
                        frame 11 {
                          n1016 = global write "全局 所有参数.vi" "总磷"(w1113) -> ()
                        }
                        frame 12 {
                          n1017 = global write "全局 所有参数.vi" "叶绿素"(w1114) -> ()
                        }
                        frame 13 {
                          n1018 = global write "全局 所有参数.vi" "藻密度"(w1115) -> ()
                        }
                        frame 14 {
                          n1019 = global write "全局 所有参数.vi" "水位"(w1116) -> ()
                        }
                        frame 15 {
                          n1020 = global write "全局 所有参数.vi" "流速"(w1117) -> ()
                        }
                        frame 16 {
                          n1021 = global write "全局 所有参数.vi" "瞬时流量"(w1118) -> ()
                        }
                        frame 17 {
                          n1022 = global write "全局 所有参数.vi" "累积流量"(w1119) -> ()
                        }
                      }
                      n1023 = Index Array(array=w1094, index (row)=w1095, index (col)=w1095) -> ()  [unwired: 1 out]
                    }
                    n1024 = flat-sequence {
                      tunnel: w1047 -> [w1050]
                      tunnel: [w1050] -> w1046
                      tunnel: w1046 -> [w1056]
                      tunnel: [w1055] -> _
                      frame #0 {
                        n1025 = global write "全局 小时数据发送次数.vi" "小时数据发送次数"(0 ("小时数据发送次数")) -> ()
                        n1026 = call "数据处理直接插入整合 (子VI).vi"() -> ()  [unwired: 12 in]
                        n1027 = global write "全局1.vi" "枚举"(enum16{"返回请求应答", "上传数据", "返回执行结果"}."上传数据" ("枚举")) -> ()
                        n1028 = global write "全局 实时数据参数.vi" "实时数据参数"("水样测试" ("实时数据参数")) -> ()
                        n1029 = global write "全局 水样时间.vi" "选择发送的参数"("氨氮" ("选择发送的参数")) -> ()
                      }
                      frame #1 {
                        # "实时数据的大小"
                        n1030 = flat-sequence {
                          tunnel: [w1062] -> w1059
                          tunnel: [w1061] -> w1057
                          tunnel: w1056 -> [w1060]
                          tunnel: w1059 -> [_]
                          tunnel: [w1075] -> w1058
                          tunnel: w1057 -> [w1075]
                          tunnel: w1058 -> [w1083]
                          tunnel: [w1077] -> w1055
                          frame #0 {
                            n1031 = Get Date/Time In Seconds() -> (seconds since 1Jan1904=w1070:timestamp)
                            n1032 = Format Date/Time String(time format string (%c)="%Y%m%d%H%M%S%3u" ("时间格式字符串(%c)"), seconds (now)=w1070) -> (date/time string=w1071:string)  [unwired: 1 in]
                            n1033 = Search and Replace String(input string=w1071, search string="." ("搜索字符串")) -> (result string=w1073:string)  [unwired: 6 in, 3 out]
                            n1034 = local read "MN"() -> (w1066:string)
                            n1035 = local read "PW"() -> (w1065:string)
                            n1036 = local read "数据发送通道"() -> (w1064:enum16{"TCP", "VISA"})
                            n1037 = call "数据编码.vi"("table输入"="小时数据" ("新元素/子数组"), "QN"=w1073, "MN"=w1066, "PW"=w1065) -> ("通讯包字符串"=w1062:string)  [unwired: 10 in, 1 out]
                            n1038 = Build Array(w1062) -> (w1067:string[])
                            n1039 = local write "发送报文显示"(w1062) -> ()
                            n1040 = call "VISATCP组合选择发送.vi"("数据发送通道"=w1064, "命令"="write", "写入缓冲区"=w1062) -> ()  [unwired: 9 in, 4 out]
                            n1041 = call "发送数据记录到文档(子VI).vi"("错误输入"=w1060, "数组"=w1067) -> ("错误输出"=w1061:errorcluster)  [unwired: 8 in]
                          }
                          frame #1 {
                            n1042 = global write "全局 小时数据发送次数.vi" "小时数据发送次数"(0 ("小时数据发送次数")) -> ()
                            n1043 = Wait (ms)(milliseconds to wait=u32 500 ("等待时间（毫秒）")) -> ()  [unwired: 1 out]
                          }
                          frame #2 {
                            n1044 = local read "MN"() -> (w1082:string)
                            n1045 = local read "PW"() -> (w1081:string)
                            n1046 = call "数据编码.vi"("table输入"="实时数据" ("新元素/子数组"), "错误常量 2"=w1083, "MN"=w1082, "PW"=w1081) -> ("通讯包字符串"=w1078:string)  [unwired: 10 in, 1 out]
                            n1047 = Build Array(w1078) -> (w1085:string[])
                            n1048 = local read "数据发送通道"() -> (w1080:enum16{"TCP", "VISA"})
                            n1049 = local write "发送报文显示"(w1078) -> ()
                            n1050 = call "发送数据记录到文档(子VI).vi"("数组"=w1085) -> ()  [unwired: 9 in, 1 out]
                            n1051 = call "VISATCP组合选择发送.vi"("数据发送通道"=w1080, "命令"="write", "写入缓冲区"=w1078) -> ("错误输出"=w1077:errorcluster)  [unwired: 9 in, 3 out]
                          }
                        }
                      }
                    }
                  }
                  frame "2017-212协议", Default {
                    n1052 = local read "参数数值"() -> (w1183:T5)
                    n1053 = Cluster To Array(cluster=w1183) -> (array=w1182:bool[])
                    n1054 = for {
                      tunnel: w1182 -> [_] mode=indexing
                      tunnel: [w1190] -> w1181 mode=indexing
                      tunnel: [w1190] -> _
                      i -> [w1188]
                      (unwired) " where 时间 between #"
                      w1187 = "database1.mdb" ("database")
                      (unwired) "'and 数据类型 ='N' and 时间 between "
                      w1204 = 0 ("索引 (行)")
                      n1055 = case shown="3" w1188 {
                        tunnel: [w1374 w1376 w1378 w1380 w1382 w1384 w1386 w1388 w1390 w1392 w1394 w1396 w1398 w1400 w1402 w1404 w1406 w1408] -> w1186
                        frame 0, Default {
                          n1056 = control-ref of="CODMn"() -> (w1375:refnum<vi>)
                          n1057 = property class="Bool (严格)"(reference=w1375) -> ("Label.Text"=w1374:string)  [unwired: 1 in, 2 out]
                        }
                        frame 1 {
                          n1058 = control-ref of="CODCr"() -> (w1377:refnum<vi>)
                          n1059 = property class="Bool (严格)"(reference=w1377) -> ("Label.Text"=w1376:string)  [unwired: 1 in, 2 out]
                        }
                        frame 2 {
                          n1060 = control-ref of="DO"() -> (w1379:refnum<vi>)
                          n1061 = property class="Bool (严格)"(reference=w1379) -> ("Label.Text"=w1378:string)  [unwired: 1 in, 2 out]
                        }
                        frame 3 {
                          n1062 = control-ref of="铜"() -> (w1381:refnum<vi>)
                          n1063 = property class="Bool (严格)"(reference=w1381) -> ("Label.Text"=w1380:string)  [unwired: 1 in, 2 out]
                        }
                        frame 4 {
                          n1064 = control-ref of="PH"() -> (w1383:refnum<vi>)
                          n1065 = property class="Bool (严格)"(reference=w1383) -> ("Label.Text"=w1382:string)  [unwired: 1 in, 2 out]
                        }
                        frame 5 {
                          n1066 = control-ref of="氨氮"() -> (w1385:refnum<vi>)
                          n1067 = property class="Bool (严格)"(reference=w1385) -> ("Label.Text"=w1384:string)  [unwired: 1 in, 2 out]
                        }
                        frame 6 {
                          n1068 = control-ref of="比电导率"() -> (w1387:refnum<vi>)
                          n1069 = property class="Bool (严格)"(reference=w1387) -> ("Label.Text"=w1386:string)  [unwired: 1 in, 2 out]
                        }
                        frame 7 {
                          n1070 = control-ref of="水温"() -> (w1389:refnum<vi>)
                          n1071 = property class="Bool (严格)"(reference=w1389) -> ("Label.Text"=w1388:string)  [unwired: 1 in, 2 out]
                        }
                        frame 8 {
                          n1072 = control-ref of="盐度(海水)"() -> (w1391:refnum<vi>)
                          n1073 = property class="Bool (严格)"(reference=w1391) -> ("Label.Text"=w1390:string)  [unwired: 1 in, 2 out]
                        }
                        frame 9 {
                          n1074 = control-ref of="浊度"() -> (w1393:refnum<vi>)
                          n1075 = property class="Bool (严格)"(reference=w1393) -> ("Label.Text"=w1392:string)  [unwired: 1 in, 2 out]
                        }
                        frame 10 {
                          n1076 = control-ref of="总氮"() -> (w1395:refnum<vi>)
                          n1077 = property class="Bool (严格)"(reference=w1395) -> ("Label.Text"=w1394:string)  [unwired: 1 in, 2 out]
                        }
                        frame 11 {
                          n1078 = control-ref of="总磷"() -> (w1397:refnum<vi>)
                          n1079 = property class="Bool (严格)"(reference=w1397) -> ("Label.Text"=w1396:string)  [unwired: 1 in, 2 out]
                        }
                        frame 12 {
                          n1080 = control-ref of="叶绿素a"() -> (w1399:refnum<vi>)
                          n1081 = property class="Bool (严格)"(reference=w1399) -> ("Label.Text"=w1398:string)  [unwired: 1 in, 2 out]
                        }
                        frame 13 {
                          n1082 = control-ref of="藻密度"() -> (w1401:refnum<vi>)
                          n1083 = property class="Bool (严格)"(reference=w1401) -> ("Label.Text"=w1400:string)  [unwired: 1 in, 2 out]
                        }
                        frame 14 {
                          n1084 = control-ref of="水位"() -> (w1403:refnum<vi>)
                          n1085 = property class="Bool (严格)"(reference=w1403) -> ("Label.Text"=w1402:string)  [unwired: 1 in, 2 out]
                        }
                        frame 15 {
                          n1086 = control-ref of="流速"() -> (w1405:refnum<vi>)
                          n1087 = property class="Bool (严格)"(reference=w1405) -> ("Label.Text"=w1404:string)  [unwired: 1 in, 2 out]
                        }
                        frame 16 {
                          n1088 = control-ref of="瞬时流量"() -> (w1407:refnum<vi>)
                          n1089 = property class="Bool (严格)"(reference=w1407) -> ("Label.Text"=w1406:string)  [unwired: 1 in, 2 out]
                        }
                        frame 17 {
                          n1090 = control-ref of="累积流量"() -> (w1409:refnum<vi>)
                          n1091 = property class="Bool (严格)"(reference=w1409) -> ("Label.Text"=w1408:string)  [unwired: 1 in, 2 out]
                        }
                      }
                      n1092 = case shown="12" w1188 {
                        tunnel: [w1356 w1357 w1358 w1359 w1360 w1361 w1362 w1363 w1364 w1365 w1366 w1367 w1368 w1369 w1370 w1371 w1372 w1373] -> w1185
                        frame 0, Default {
                          n1093 = global read "全局 水样时间.vi" "time1"() -> (w1356:string)
                        }
                        frame 1 {
                          n1094 = global read "全局 水样时间.vi" "time2"() -> (w1357:string)
                        }
                        frame 2 {
                          n1095 = global read "全局 水样时间.vi" "time3"() -> (w1358:string)
                        }
                        frame 3 {
                          n1096 = global read "全局 水样时间.vi" "time4"() -> (w1359:string)
                        }
                        frame 4 {
                          n1097 = global read "全局 水样时间.vi" "time5"() -> (w1360:string)
                        }
                        frame 5 {
                          n1098 = global read "全局 水样时间.vi" "time6"() -> (w1361:string)
                        }
                        frame 6 {
                          n1099 = global read "全局 水样时间.vi" "time7"() -> (w1362:string)
                        }
                        frame 7 {
                          n1100 = global read "全局 水样时间.vi" "time8"() -> (w1363:string)
                        }
                        frame 8 {
                          n1101 = global read "全局 水样时间.vi" "time9"() -> (w1364:string)
                        }
                        frame 9 {
                          n1102 = global read "全局 水样时间.vi" "time10"() -> (w1365:string)
                        }
                        frame 10 {
                          n1103 = global read "全局 水样时间.vi" "time11"() -> (w1366:string)
                        }
                        frame 11 {
                          n1104 = global read "全局 水样时间.vi" "time12"() -> (w1367:string)
                        }
                        frame 12 {
                          n1105 = global read "全局 水样时间.vi" "time13"() -> (w1368:string)
                        }
                        frame 13 {
                          n1106 = global read "全局 水样时间.vi" "time14"() -> (w1369:string)
                        }
                        frame 14 {
                          n1107 = global read "全局 水样时间.vi" "time15"() -> (w1370:string)
                        }
                        frame 15 {
                          n1108 = global read "全局 水样时间.vi" "time16"() -> (w1371:string)
                        }
                        frame 16 {
                          n1109 = global read "全局 水样时间.vi" "time17"() -> (w1372:string)
                        }
                        frame 17 {
                          n1110 = global read "全局 水样时间.vi" "time18"() -> (w1373:string)
                        }
                      }
                      n1111 = Get Date/Time In Seconds() -> (seconds since 1Jan1904=w1209:timestamp)
                      n1112 = Format Date/Time String(time format string (%c)="%Y/%m/%d %H:%M:%S" ("时间格式字符串(%c)"), seconds (now)=w1209) -> (date/time string=w1184:string)  [unwired: 1 in]
                      n1113 = Format Into String(format string="#%s#" ("初始字符串"), w1185) -> (resulting string=w1207:string)  [unwired: 2 in, 1 out]
                      n1114 = Format Into String(format string="#%s#" ("初始字符串"), w1184) -> (resulting string=w1189:string)  [unwired: 2 in, 1 out]
                      n1115 = case shown="0, 默认" w1188 {
                        selector: w1188 -> [_ w1223]
                        tunnel: w1207 -> [w1218 w1228]
                        tunnel: [w1217 w1229] -> w1206
                        tunnel: w1189 -> [w1215 w1227]
                        tunnel: w1187 -> [_ w1226]
                        tunnel: w1186 -> [_ w1225]
                        tunnel: w1185 -> [_ w1220]
                        tunnel: w1184 -> [_ w1222]
                        frame 0, Default {
                          (unwired) " order by 时间 asc" ("字符串")
                          n1116 = Concatenate Strings("where 测量模式 ='水样测试" ("condition"), "'and 时间 between ", w1218, "and" ("字符串"), w1215, " order by 时间 desc" ("字符串")) -> (w1217:string)
                        }
                        frame 14..17 {
                          n1117 = call "流量数据规范小时时间戳.vi"("字符串"=w1220) -> ("result string"=w1219:string)  [unwired: 10 in]
                          n1118 = call "database1查询.vi"("时间2"=w1222, "table"=w1225, "时间1"=w1219, "database"=w1226) -> ("error out"=w1221:errorcluster, "data"=w1224:string[][])  [unwired: 4 in, 1 out]
                          n1119 = call <vilib>:"Clear Errors.vi"("error in (no error)"=w1221) -> ()  [unwired: 5 in, 2 out]
                          n1120 = case shown="14" w1223 {
                            tunnel: w1224 -> [_ w1233 w1234 w1235 w1236]
                            frame 0, Default {
                            }
                            frame 14 {
                              n1121 = global write "全局流量数据小时.vi" "水位"(w1233) -> ()
                            }
                            frame 15 {
                              n1122 = global write "全局流量数据小时.vi" "流速"(w1234) -> ()
                            }
                            frame 16 {
                              n1123 = global write "全局流量数据小时.vi" "瞬时流量"(w1235) -> ()
                            }
                            frame 17 {
                              n1124 = global write "全局流量数据小时.vi" "累积流量"(w1236) -> ()
                            }
                          }
                          n1125 = Concatenate Strings(" where 时间 between ", w1228, "and" ("字符串"), w1227, " order by 时间 desc" ("字符串")) -> (w1229:string)
                        }
                      }
                      n1126 = call "SQL查询.vi"("condition"=w1206, "table输入"=w1186, "database"=w1187) -> ("error out"=w1190:errorcluster, "data"=w1202:string[][])  [unwired: 7 in]
                      n1127 = Empty Array?(array=w1202) -> (empty?=w1205:bool)
                      n1128 = call "短日期时间转长日期格式.vi"("data"=w1202) -> ("输出数组"=w1203:string[][])  [unwired: 10 in]
                      n1129 = Not(x=w1205) -> (.not. x?=w1199:bool)
                      n1130 = Index Array(array=w1203, index (row)=w1204, index (col)=w1204) -> (element=w1196:string)
                      n1131 = global write "全局 水样时间.vi" "选择发送的参数"(w1186) -> ()
                      n1132 = flat-sequence {
                        tunnel: [w1244] -> w1201
                        tunnel: [w1243] -> w1200
                        tunnel: w1199 -> [w1244]
                        tunnel: w1202 -> [w1243]
                        tunnel: w1188 -> [w1238]
                        tunnel: w1186 -> [w1240]
                        tunnel: [w1240] -> w1197
                        tunnel: w1196 -> [w1239]
                        tunnel: [w1239] -> w1194
                        tunnel: [w1238] -> w1191
                        tunnel: w1201 -> [w1264]
                        tunnel: w1200 -> [w1267]
                        tunnel: [w1266] -> w1198
                        tunnel: w1197 -> [w1266]
                        tunnel: [w1265] -> w1195
                        tunnel: w1194 -> [w1265]
                        tunnel: [w1264] -> w1193
                        tunnel: [w1263] -> w1192
                        tunnel: w1191 -> [w1263]
                        tunnel: w1198 -> [w1324]
                        tunnel: w1195 -> [w1323]
                        tunnel: w1193 -> [w1321]
                        tunnel: w1192 -> [w1322]
                        frame #0 {
                          n1133 = case shown="3" w1238 {
                            tunnel: w1243 -> [w1245 w1246 w1247 w1248 w1249 w1250 w1251 w1252 w1253 w1254 w1255 w1256 w1257 w1258 w1259 w1260 w1261 w1262]
                            frame 0, Default {
                              n1134 = global write "全局 所有参数.vi" "CODMn"(w1245) -> ()
                            }
                            frame 1 {
                              n1135 = global write "全局 所有参数.vi" "CODCr"(w1246) -> ()
                            }
                            frame 2 {
                              n1136 = global write "全局 所有参数.vi" "DO"(w1247) -> ()
                            }
                            frame 3 {
                              n1137 = global write "全局 所有参数.vi" "铜"(w1248) -> ()
                            }
                            frame 4 {
                              n1138 = global write "全局 所有参数.vi" "PH"(w1249) -> ()
                            }
                            frame 5 {
                              n1139 = global write "全局 所有参数.vi" "氨氮"(w1250) -> ()
                            }
                            frame 6 {
                              n1140 = global write "全局 所有参数.vi" "电导率"(w1251) -> ()
                            }
                            frame 7 {
                              n1141 = global write "全局 所有参数.vi" "水温"(w1252) -> ()
                            }
                            frame 8 {
                              n1142 = global write "全局 所有参数.vi" "盐度"(w1253) -> ()
                            }
                            frame 9 {
                              n1143 = global write "全局 所有参数.vi" "浊度"(w1254) -> ()
                            }
                            frame 10 {
                              n1144 = global write "全局 所有参数.vi" "总氮"(w1255) -> ()
                            }
                            frame 11 {
                              n1145 = global write "全局 所有参数.vi" "总磷"(w1256) -> ()
                            }
                            frame 12 {
                              n1146 = global write "全局 所有参数.vi" "叶绿素"(w1257) -> ()
                            }
                            frame 13 {
                              n1147 = global write "全局 所有参数.vi" "藻密度"(w1258) -> ()
                            }
                            frame 14 {
                              n1148 = global write "全局 所有参数.vi" "水位"(w1259) -> ()
                            }
                            frame 15 {
                              n1149 = global write "全局 所有参数.vi" "流速"(w1260) -> ()
                            }
                            frame 16 {
                              n1150 = global write "全局 所有参数.vi" "瞬时流量"(w1261) -> ()
                            }
                            frame 17 {
                              n1151 = global write "全局 所有参数.vi" "累积流量"(w1262) -> ()
                            }
                          }
                          n1152 = global write "全局 小时数据发送次数.vi" "小时数据发送次数"(0 ("小时数据发送次数")) -> ()
                          n1153 = global write "全局 数据发送重叠.vi" "数据接收超时指示灯"(FALSE ("数据接收超时指示灯")) -> ()
                          n1154 = global write "全局1.vi" "枚举"(enum16{"返回请求应答", "上传数据", "返回执行结果"}."上传数据" ("枚举")) -> ()
                        }
                        frame #1 {
                          n1155 = case shown="真" w1264 {
                            tunnel: w1267 -> [_ w1270]
                            tunnel: w1263 -> [_ w1269]
                            tunnel: w1263 -> [_ w1268]
                            frame False {
                            }
                            frame True {
                              n1156 = for {
                                tunnel: w1270 -> [_] mode=indexing
                                tunnel: w1269 -> [w1288]
                                tunnel: w1268 -> [w1287]
                                # "实时数据的大小"
                                n1157 = Wait (ms)(milliseconds to wait=u32 500 ("等待时间（毫秒）")) -> ()  [unwired: 1 out]
                                n1158 = global write "全局 实时数据参数.vi" "实时数据参数"("水样测试" ("实时数据参数")) -> ()
                                n1159 = Get Date/Time In Seconds() -> (seconds since 1Jan1904=w1281:timestamp)
                                n1160 = Format Date/Time String(time format string (%c)="%Y%m%d%H%M%S%3u" ("时间格式字符串(%c)"), seconds (now)=w1281) -> (date/time string=w1282:string)  [unwired: 1 in]
                                n1161 = Search and Replace String(input string=w1282, search string="." ("搜索字符串")) -> (result string=w1284:string)  [unwired: 6 in, 3 out]
                                n1162 = local read "MN"() -> (w1276:string)
                                n1163 = local read "PW"() -> (w1275:string)
                                n1164 = local read "数据发送通道"() -> (w1274:enum16{"TCP", "VISA"})
                                n1165 = call "数据编码.vi"("table输入"="小时数据" ("新元素/子数组"), "QN"=w1284, "MN"=w1276, "PW"=w1275) -> ("通讯包字符串"=w1286:string)  [unwired: 10 in, 1 out]
                                n1166 = Build Array(w1286) -> (w1278:string[])
                                n1167 = local write "发送报文显示"(w1286) -> ()
                                n1168 = call "VISATCP组合选择发送.vi"("数据发送通道"=w1274, "命令"="write", "写入缓冲区"=w1286) -> ()  [unwired: 9 in, 4 out]
                                n1169 = call "发送数据记录到文档(子VI).vi"("数组"=w1278) -> ()  [unwired: 9 in, 1 out]
                                n1170 = local read "判断数据反馈"() -> (w1272:bool)
                                n1171 = case shown="真" w1272 {
                                tunnel: [_ w1311] -> w1285
                                tunnel: w1286 -> [_ w1310]
                                tunnel: w1288 -> [_ w1309]
                                frame False {
                                }
                                frame True {
                                n1172 = case shown="0, 默认" w1309 {
                                tunnel: [w1313 _] -> w1311
                                tunnel: w1310 -> [w1312 _]
                                frame 0, Default {
                                n1173 = Empty String/Path?(string/path=w1312) -> (empty?=w1314:bool)
                                n1174 = case shown="假" w1314 {
                                tunnel: [w1317 _] -> w1313
                                tunnel: w1312 -> [w1316 _]
                                frame False {
                                n1175 = local read "数据发送通道"() -> (w1315:enum16{"TCP", "VISA"})
                                n1176 = call "数据补发判定有限循环.vi"("数据输入"=w1316, "数据发送通道"=w1315) -> ("error out"=w1317:errorcluster)  [unwired: 9 in]
                                }
                                frame True {
                                }
                                }
                                }
                                frame 14..17 {
                                }
                                }
                                }
                                }
                                n1177 = local read "2011发送"() -> (w1271:bool)
                                n1178 = case shown="真" w1271 {
                                tunnel: w1287 -> [_ w1301]
                                tunnel: w1285 -> [_ w1300]
                                frame False {
                                }
                                frame True {
                                n1179 = local read "MN"() -> (w1295:string)
                                n1180 = local read "PW"() -> (w1294:string)
                                n1181 = global write "全局 实时数据参数.vi" "实时数据参数"("水样测试" ("实时数据参数")) -> ()
                                n1182 = call "数据编码.vi"("table输入"="实时数据" ("新元素/子数组"), "错误常量 2"=w1300, "MN"=w1295, "PW"=w1294) -> ("通讯包字符串"=w1299:string)  [unwired: 10 in, 1 out]
                                n1183 = Build Array(w1299) -> (w1297:string[])
                                n1184 = local read "数据发送通道"() -> (w1293:enum16{"TCP", "VISA"})
                                n1185 = local write "发送报文显示"(w1299) -> ()
                                n1186 = call "发送数据记录到文档(子VI).vi"("数组"=w1297) -> ()  [unwired: 9 in, 1 out]
                                n1187 = call "VISATCP组合选择发送.vi"("数据发送通道"=w1293, "命令"="write", "写入缓冲区"=w1299) -> ("错误输出"=w1298:errorcluster)  [unwired: 9 in, 3 out]
                                n1188 = local read "判断数据反馈"() -> (w1290:bool)
                                n1189 = case shown="真" w1290 {
                                tunnel: w1299 -> [_ w1304]
                                tunnel: w1298 -> [_ w1303]
                                tunnel: w1301 -> [_ w1302]
                                frame False {
                                }
                                frame True {
                                n1190 = case shown="0, 默认" w1302 {
                                tunnel: w1304 -> [w1308 _]
                                tunnel: w1303 -> [w1307 _]
                                frame 0, Default {
                                n1191 = local read "数据发送通道"() -> (w1305:enum16{"TCP", "VISA"})
                                n1192 = call "数据补发判定有限循环.vi"("错误输入（无错误）"=w1307, "数据输入"=w1308, "数据发送通道"=w1305) -> ("error out"=w1306:errorcluster)  [unwired: 8 in]
                                n1193 = local write "错误输出"(w1306) -> ()
                                }
                                frame 14..17 {
                                }
                                }
                                }
                                }
                                }
                                }
                              }
                            }
                          }
                        }
                        frame #2 {
                          n1194 = global read "全局 数据发送重叠.vi" "数据接收超时指示灯"() -> (w1318:bool)
                          n1195 = Not(x=w1318) -> (.not. x?=w1319:bool)
                          n1196 = Compound Arithmetic op=AND ("复合运算")(w1319, w1321) -> (w1320:bool)
                          n1197 = case shown="真" w1320 {
                            tunnel: w1323 -> [_ w1327]
                            tunnel: w1322 -> [_ w1337]
                            tunnel: w1324 -> [_ w1328]
                            frame False {
                            }
                            frame True {
                              n1198 = call "日期时间字符串转换分钟数加一.vi"("data[0]"=w1327) -> ("日期/时间字符串"=w1325:string)  [unwired: 10 in]
                              n1199 = call "时间日期字符串至时间标识转换.vi"("时间日期字符串"=w1325) -> ("时间标识"=w1326:timestamp)  [unwired: 10 in]
                              n1200 = call <vilib>:"Application Directory.vi"() -> ("Application Directory"=w1329:path)
                              n1201 = case shown="3" w1337 {
                                tunnel: w1325 -> [w1338 w1339 w1340 w1341 w1342 w1343 w1344 w1345 w1346 w1347 w1348 w1349 w1350 w1351 w1352 w1353 w1354 w1355]
                                frame 0, Default {
                                n1202 = global write "全局 水样时间.vi" "time1"(w1338) -> ()
                                }
                                frame 1 {
                                n1203 = global write "全局 水样时间.vi" "time2"(w1339) -> ()
                                }
                                frame 2 {
                                n1204 = global write "全局 水样时间.vi" "time3"(w1340) -> ()
                                }
                                frame 3 {
                                n1205 = global write "全局 水样时间.vi" "time4"(w1341) -> ()
                                }
                                frame 4 {
                                n1206 = global write "全局 水样时间.vi" "time5"(w1342) -> ()
                                }
                                frame 5 {
                                n1207 = global write "全局 水样时间.vi" "time6"(w1343) -> ()
                                }
                                frame 6 {
                                n1208 = global write "全局 水样时间.vi" "time7"(w1344) -> ()
                                }
                                frame 7 {
                                n1209 = global write "全局 水样时间.vi" "time8"(w1345) -> ()
                                }
                                frame 8 {
                                n1210 = global write "全局 水样时间.vi" "time9"(w1346) -> ()
                                }
                                frame 9 {
                                n1211 = global write "全局 水样时间.vi" "time10"(w1347) -> ()
                                }
                                frame 10 {
                                n1212 = global write "全局 水样时间.vi" "time11"(w1348) -> ()
                                }
                                frame 11 {
                                n1213 = global write "全局 水样时间.vi" "time12"(w1349) -> ()
                                }
                                frame 12 {
                                n1214 = global write "全局 水样时间.vi" "time13"(w1350) -> ()
                                }
                                frame 13 {
                                n1215 = global write "全局 水样时间.vi" "time14"(w1351) -> ()
                                }
                                frame 14 {
                                n1216 = global write "全局 水样时间.vi" "time15"(w1352) -> ()
                                }
                                frame 15 {
                                n1217 = global write "全局 水样时间.vi" "time16"(w1353) -> ()
                                }
                                frame 16 {
                                n1218 = global write "全局 水样时间.vi" "time17"(w1354) -> ()
                                }
                                frame 17 {
                                n1219 = global write "全局 水样时间.vi" "time18"(w1355) -> ()
                                }
                              }
                              n1220 = Build Path(base path=w1329, name or relative path="data\\Set.ini" ("名称或相对路径")) -> (appended path=w1331:path)
                              n1221 = call <vilib>:"Open Config Data.vi"("configuration file path"=w1331) -> ("error out"=w1333:errorcluster, "refnum"=w1332:T8)  [unwired: 8 in, 1 out]
                              n1222 = local write "数据发送起始时间"(w1326) -> ()
                              n1223 = call-poly <vilib>:"Write Key.vi"("section"="线程一数据搜索起始时间", "error in (no error)"=w1333, "value"=w1325, "key"=w1328, "refnum"=w1332) -> ("error out"=w1335:errorcluster, "refnum out"=w1334:T8)  [unwired: 4 in, 1 out]
                              n1224 = call <vilib>:"Close Config Data.vi"("error in (no error)"=w1335, "refnum"=w1334) -> ()  [unwired: 8 in, 2 out]
                            }
                          }
                        }
                      }
                    }
                  }
                }
                "实时小时数据上传" <- w1043
              }
              frame #1 {
                w1410 = FALSE ("小时数据上传")
                n1225 = local write "实时小时数据上传"(w1410) -> ()
                n1226 = global write "全局 数据发送重叠.vi" "主动上报数据中"(w1410) -> ()
              }
            }
          }
          frame True {
            # "数据整点触发，整条发送"
          }
        }
      }
    }
  }
  n1227 = while {
    stop <- FALSE stop-if-true
    # "数据整点触发，整条发送"
    n1228 = global read "断电保存全局.vi" "数据组合发送"() -> (w1412:bool)
    n1229 = case shown="真" w1412 {
      frame False {
      }
      frame True {
        n1230 = Get Date/Time In Seconds() -> (seconds since 1Jan1904=w1422:timestamp)
        n1231 = Seconds To Date/Time(time stamp (now)=w1422) -> (date time rec=w1423:T9)  [unwired: 1 in]
        n1232 = global read "断电保存全局.vi" "数据重发"() -> (w1415:bool)
        n1233 = Unbundle By Name(w1423) -> ("分"=w1421:i32)
        n1234 = Equal?(x=w1421, y=0) -> (x = y?=w1419:bool)
        n1235 = call <vilib>:"Boolean Crossing PtByPt.vi"("direction"=enum16{"either", "false-true", "true-false"}."false-true", "input"=w1419) -> ("crossing"=w1417:bool)  [unwired: 1 in]
        n1236 = Or(x=w1415, y=w1417) -> (x .or. y?=w1416:bool)
        n1237 = case shown="真" w1416 {
          frame False {
            n1238 = global write "全局 数据发送重叠.vi" "主动上报数据中"(FALSE ("主动上报数据中")) -> ()
          }
          frame True {
            n1239 = local read "数据发送通道"() -> (w1427:enum16{"TCP", "VISA"})
            n1240 = local read "MN"() -> (w1426:string)
            n1241 = local read "PW"() -> (w1425:string)
            n1242 = call "数据全参数一起发送整点触发.vi"("数据发送通道"=w1427, "PW"=w1425, "MN"=w1426) -> ()  [unwired: 8 in]
          }
        }
      }
    }
    n1243 = Wait (ms)(milliseconds to wait=u32 1000 ("等待时间（毫秒）")) -> ()  [unwired: 1 out]
  }
  n1244 = while {
    stop <- FALSE stop-if-true
    # "定期释放缓存"
    n1245 = Wait (ms)(milliseconds to wait=u32 600000 ("等待时间（毫秒）")) -> ()  [unwired: 1 out]
    n1246 = dll-call lib="PTH2Sabs F\tgitkrakenCC(平台数采程序 - V1.0（正式版）dataFreeMem.dll" fn="FreeMem"() -> ()  [unwired: 4 in, 2 out]
  }
  n1247 = while {
    stop <- FALSE stop-if-true
    n1248 = event shown="[12] \"确定更改起始时间\": 值改变" {
      selector: _ -> [_ _ _ _ _ _ _ _ _ _ _ _ _ _ _ _ _ _]
      dyn-events: _ -> [_ _ _ _ _ _ _ _ _ _ _ _ _ _ _ _ _ _]
      timeout: _ -> [_ _ _ _ _ _ _ _ _ _ _ _ _ _ _ _ _ _]
      event Timeout {
        n1249 = event-data() -> ()  [unwired: 1 in, 2 out]
      }
      event "站点名称", "站点设备", "IP", "PORT", "MN", "PW", "VISA resource name", "baud rate": Value Change {
        w1433 = "线程一自主部署站点保存"
        # "TCP服务器端口掉线"
        n1250 = event-data() -> ()  [unwired: 1 in, 6 out]
        n1251 = call <vilib>:"Application Directory.vi"() -> ("Application Directory"=w1475:path)
        n1252 = local read "站点名称"() -> (w1454:string)
        n1253 = Build Path(base path=w1475, name or relative path="data\\Set.ini" ("名称或相对路径")) -> (appended path=w1473:path)
        n1254 = call <vilib>:"Open Config Data.vi"("configuration file path"=w1473) -> ("error out"=w1471:errorcluster, "refnum"=w1472:T8)  [unwired: 8 in, 1 out]
        n1255 = local read "站点设备"() -> (w1453:string)
        n1256 = call-poly <vilib>:"Write Key.vi"("section"=w1433, "error in (no error)"=w1471, "value"=w1454, "key"="站点名称", "refnum"=w1472) -> ("error out"=w1468:errorcluster, "refnum out"=w1469:T8)  [unwired: 4 in, 1 out]
        n1257 = call-poly <vilib>:"Write Key.vi"("section"=w1433, "error in (no error)"=w1468, "value"=w1453, "key"="站点设备", "refnum"=w1469) -> ("error out"=w1465:errorcluster, "refnum out"=w1466:T8)  [unwired: 4 in, 1 out]
        n1258 = local read "IP"() -> (w1452:string)
        n1259 = call-poly <vilib>:"Write Key.vi"("section"=w1433, "error in (no error)"=w1465, "value"=w1452, "key"="IP", "refnum"=w1466) -> ("error out"=w1463:errorcluster, "refnum out"=w1464:T8)  [unwired: 4 in, 1 out]
        n1260 = local read "PORT"() -> (w1451:string)
        n1261 = call-poly <vilib>:"Write Key.vi"("section"=w1433, "error in (no error)"=w1463, "value"=w1451, "key"="PORT", "refnum"=w1464) -> ("error out"=w1461:errorcluster, "refnum out"=w1462:T8)  [unwired: 4 in, 1 out]
        n1262 = local read "MN"() -> (w1445:string)
        n1263 = call-poly <vilib>:"Write Key.vi"("section"=w1433, "error in (no error)"=w1461, "value"=w1445, "key"="MN", "refnum"=w1462) -> ("error out"=w1446:errorcluster, "refnum out"=w1449:T8)  [unwired: 4 in, 1 out]
        n1264 = local read "PW"() -> (w1447:string)
        n1265 = call-poly <vilib>:"Write Key.vi"("section"=w1433, "error in (no error)"=w1446, "value"=w1447, "key"="PW", "refnum"=w1449) -> ("error out"=w1434:errorcluster, "refnum out"=w1435:T8)  [unwired: 4 in, 1 out]
        n1266 = local read "VISA resource name"() -> (w1441:refnum<visa-resource-name>)
        n1267 = local read "主队列输出"() -> (w1460:refnum<queue>)
        n1268 = call-poly <vilib>:"Write Key.vi"("section"=w1433, "error in (no error)"=w1434, "value"=w1441, "key"="VISA", "refnum"=w1435) -> ("error out"=w1440:errorcluster, "refnum out"=w1437:T8)  [unwired: 4 in, 1 out]
        n1269 = local read "baud rate"() -> (w1439:u32)
        n1270 = Flush Queue(queue=w1460) -> (queue out=w1459:refnum<queue>)  [unwired: 1 in, 2 out]
        n1271 = call-poly <vilib>:"Write Key.vi"("section"=w1433, "error in (no error)"=w1440, "value"=w1439, "key"="BAUDRATE", "refnum"=w1437) -> ("error out"=w1431:errorcluster, "refnum out"=w1432:T8)  [unwired: 4 in, 1 out]
        n1272 = local read "数据发送通道"() -> (w1444:enum16{"TCP", "VISA"})
        n1273 = call <vilib>:"Close Config Data.vi"("error in (no error)"=w1431, "refnum"=w1432) -> ()  [unwired: 8 in, 2 out]
        n1274 = call "VISATCP组合选择发送.vi"("数据发送通道"=w1444, "命令"="close") -> ("错误输出"=w1442:errorcluster)  [unwired: 10 in, 3 out]
        n1275 = Enqueue Element(queue=w1459, element=T6."初始化" ("元素"), timeout in ms (-1)=1000 ("超时毫秒(-1)")) -> ()  [unwired: 1 in, 3 out]
        n1276 = call <vilib>:"Clear Errors.vi"("error in (no error)"=w1442) -> ()  [unwired: 5 in, 2 out]
      }
      event "确定": Value Change {
        w1480 = "线程一自主部署站点保存"
        # "TCP服务器端口掉线"
        n1277 = event-data() -> ()  [unwired: 1 in, 6 out]
        n1278 = call <vilib>:"Application Directory.vi"() -> ("Application Directory"=w1513:path)
        n1279 = local read "站点名称"() -> (w1508:string)
        n1280 = Build Path(base path=w1513, name or relative path="data\\Set.ini" ("名称或相对路径")) -> (appended path=w1511:path)
        n1281 = call <vilib>:"Open Config Data.vi"("configuration file path"=w1511) -> ("error out"=w1509:errorcluster, "refnum"=w1510:T8)  [unwired: 8 in, 1 out]
        n1282 = local read "站点设备"() -> (w1503:string)
        n1283 = call-poly <vilib>:"Write Key.vi"("section"=w1480, "error in (no error)"=w1509, "value"=w1508, "key"="站点名称", "refnum"=w1510) -> ("error out"=w1505:errorcluster, "refnum out"=w1506:T8)  [unwired: 4 in, 1 out]
        n1284 = call-poly <vilib>:"Write Key.vi"("section"=w1480, "error in (no error)"=w1505, "value"=w1503, "key"="站点设备", "refnum"=w1506) -> ("error out"=w1501:errorcluster, "refnum out"=w1502:T8)  [unwired: 4 in, 1 out]
        n1285 = local read "IP"() -> (w1496:string)
        n1286 = local read "PORT"() -> (w1495:string)
        n1287 = call-poly <vilib>:"Write Key.vi"("section"=w1480, "error in (no error)"=w1501, "value"=w1496, "key"="IP", "refnum"=w1502) -> ("error out"=w1499:errorcluster, "refnum out"=w1500:T8)  [unwired: 4 in, 1 out]
        n1288 = call-poly <vilib>:"Write Key.vi"("section"=w1480, "error in (no error)"=w1499, "value"=w1495, "key"="PORT", "refnum"=w1500) -> ("error out"=w1491:errorcluster, "refnum out"=w1492:T8)  [unwired: 4 in, 1 out]
        n1289 = local read "MN"() -> (w1488:string)
        n1290 = call-poly <vilib>:"Write Key.vi"("section"=w1480, "error in (no error)"=w1491, "value"=w1488, "key"="MN", "refnum"=w1492) -> ("error out"=w1489:errorcluster, "refnum out"=w1490:T8)  [unwired: 4 in, 1 out]
        n1291 = local read "PW"() -> (w1487:string)
        n1292 = call-poly <vilib>:"Write Key.vi"("section"=w1480, "error in (no error)"=w1489, "value"=w1487, "key"="PW", "refnum"=w1490) -> ("error out"=w1485:errorcluster, "refnum out"=w1486:T8)  [unwired: 4 in, 1 out]
        n1293 = call <vilib>:"Close Config Data.vi"("error in (no error)"=w1485, "refnum"=w1486) -> ("error out"=w1479:errorcluster)  [unwired: 8 in, 1 out]
        n1294 = local read "主队列输出"() -> (w1484:refnum<queue>)
        n1295 = local read "数据发送通道"() -> (w1478:enum16{"TCP", "VISA"})
        n1296 = call "VISATCP组合选择发送.vi"("数据发送通道"=w1478, "命令"="close") -> ("错误输出"=w1476:errorcluster)  [unwired: 10 in, 3 out]
        n1297 = Flush Queue(queue=w1484) -> (queue out=w1483:refnum<queue>)  [unwired: 1 in, 2 out]
        n1298 = case shown="错误" w1479 {
          frame No Error {
            n1299 = One Button Dialog(message="保存成功" ("消息"), button name ("OK")="确定" ("按钮名称（“确定”）")) -> ()  [unwired: 1 out]
          }
          frame Error {
            n1300 = One Button Dialog(message="保存失败" ("消息"), button name ("OK")="确定" ("按钮名称（“确定”）")) -> ()  [unwired: 1 out]
          }
        }
        n1301 = call <vilib>:"Clear Errors.vi"("error in (no error)"=w1476) -> ()  [unwired: 5 in, 2 out]
        n1302 = Enqueue Element(queue=w1483, element=T6."初始化" ("元素"), timeout in ms (-1)=1000 ("超时毫秒(-1)")) -> ()  [unwired: 1 in, 3 out]
      }
      event "参数配置": Value Change {
        n1303 = event-data() -> ()  [unwired: 1 in, 6 out]
        n1304 = property on="窗格" class="Pane"("Origin"=T11 {"Horizontal"=0, "Vertical"=1000} ("原点")) -> ()  [unwired: 2 in, 2 out]
      }
      event "返回": Value Change {
        n1305 = event-data() -> ()  [unwired: 1 in, 6 out]
        n1306 = property on="窗格" class="Pane"("Origin"=T11 {"Horizontal"=0, "Vertical"=0} ("原点")) -> ()  [unwired: 2 in, 2 out]
      }
      event "系统编码选择框": Value Change {
        n1307 = event-data() -> ()  [unwired: 1 in, 6 out]
        n1308 = call <vilib>:"Application Directory.vi"() -> ("Application Directory"=w1528:path)
        n1309 = Build Path(base path=w1528, name or relative path="data\\Set.ini" ("名称或相对路径")) -> (appended path=w1529:path)
        n1310 = call <vilib>:"Open Config Data.vi"("configuration file path"=w1529) -> ("error out"=w1525:errorcluster, "refnum"=w1526:T8)  [unwired: 8 in, 1 out]
        n1311 = call-poly <vilib>:"Write Key.vi"("section"="系统编码选择", "error in (no error)"=w1525, "value"="系统编码选择框", "key"="系统编码", "refnum"=w1526) -> ("error out"=w1523:errorcluster, "refnum out"=w1524:T8)  [unwired: 4 in, 1 out]
        n1312 = call <vilib>:"Close Config Data.vi"("error in (no error)"=w1523, "refnum"=w1524) -> ()  [unwired: 8 in, 2 out]
      }
      event "数据发送通道": Value Change {
        w1530 = "数据发送通道"
        n1313 = event-data() -> ()  [unwired: 1 in, 6 out]
        n1314 = local read "数据发送通道"() -> (w1531:enum16{"TCP", "VISA"})
        n1315 = call <vilib>:"Application Directory.vi"() -> ("Application Directory"=w1537:path)
        n1316 = Build Path(base path=w1537, name or relative path="data\\Set.ini" ("名称或相对路径")) -> (appended path=w1538:path)
        n1317 = call <vilib>:"Open Config Data.vi"("configuration file path"=w1538) -> ("error out"=w1534:errorcluster, "refnum"=w1535:T8)  [unwired: 8 in, 1 out]
        n1318 = call-poly <vilib>:"Write Key.vi"("section"=w1530, "error in (no error)"=w1534, "value"=w1531, "key"=w1530, "refnum"=w1535) -> ("error out"=w1532:errorcluster, "refnum out"=w1533:T8)  [unwired: 4 in, 1 out]
        n1319 = call <vilib>:"Close Config Data.vi"("error in (no error)"=w1532, "refnum"=w1533) -> ()  [unwired: 8 in, 2 out]
      }
      event "数据发送协议": Value Change {
        w1540 = "数据发送协议"
        n1320 = event-data() -> ()  [unwired: 1 in, 6 out]
        n1321 = call <vilib>:"Application Directory.vi"() -> ("Application Directory"=w1546:path)
        n1322 = Build Path(base path=w1546, name or relative path="data\\Set.ini" ("名称或相对路径")) -> (appended path=w1547:path)
        n1323 = call <vilib>:"Open Config Data.vi"("configuration file path"=w1547) -> ("error out"=w1543:errorcluster, "refnum"=w1544:T8)  [unwired: 8 in, 1 out]
        n1324 = call-poly <vilib>:"Write Key.vi"("section"=w1540, "error in (no error)"=w1543, "value"="数据发送协议", "key"=w1540, "refnum"=w1544) -> ("error out"=w1541:errorcluster, "refnum out"=w1542:T8)  [unwired: 4 in, 1 out]
        n1325 = call <vilib>:"Close Config Data.vi"("error in (no error)"=w1541, "refnum"=w1542) -> ()  [unwired: 8 in, 2 out]
      }
      event "判断数据反馈", "2011发送", "日志、参数发送", "数据组合发送": Value Change {
        n1326 = event-data() -> ()  [unwired: 1 in, 6 out]
        n1327 = flat-sequence {
          frame #0 {
            n1328 = global write "断电保存全局.vi" "日志、参数发送"("日志、参数发送") -> ()
            n1329 = global write "断电保存全局.vi" "判断数据反馈"("判断数据反馈") -> ()
            n1330 = global write "断电保存全局.vi" "2011发送"("2011发送") -> ()
            n1331 = global write "断电保存全局.vi" "数据组合发送"("数据组合发送") -> ()
          }
          frame #1 {
            n1332 = call <vilib>:"Application Directory.vi"() -> ("Application Directory"=w1552:path)
            n1333 = Build Path(base path=w1552, name or relative path="data\\sys.ini" ("名称或相对路径")) -> (appended path=w1554:path)
            n1334 = call <vilib>:"Open Config Data.vi"("configuration file path"=w1554) -> ("error out"=w1558:errorcluster, "refnum"=w1555:T8)  [unwired: 8 in, 1 out]
            n1335 = vi-ref "断电保存全局.vi"() -> (w1556:refnum<vi>)
            n1336 = call <userlib>:"Write Panel to INI__ogtk.vi"("error in (no error)"=w1558, "VI ref"=w1556, "refnum"=w1555) -> ("error out"=w1559:errorcluster, "refnum out"=w1557:T8)  [unwired: 7 in]
            n1337 = call <vilib>:"Close Config Data.vi"("error in (no error)"=w1559, "refnum"=w1557) -> ("error out"=w1564:errorcluster, "file path"=w1565:path)  [unwired: 8 in]
            n1338 = Open/Create/Replace File(file path (use dialog)=w1565, error in=w1564) -> (refnum out=w1561:refnum<file>, error out=w1560:errorcluster)  [unwired: 4 in, 1 out]
            n1339 = Flush File(refnum=w1561, error in=w1560) -> (refnum out=w1562:refnum<file>, error out=w1563:errorcluster)
            n1340 = Close File(refnum=w1562, error in=w1563) -> ()  [unwired: 2 out]
          }
        }
      }
      event "每周自动重发": Value Change {
        n1341 = event-data() -> ()  [unwired: 1 in, 6 out]
        n1342 = call <vilib>:"Application Directory.vi"() -> ("Application Directory"=w1574:path)
        n1343 = Build Path(base path=w1574, name or relative path="data\\Set.ini" ("名称或相对路径")) -> (appended path=w1575:path)
        n1344 = local read "每周自动重发"() -> (w1566:bool)
        n1345 = call <vilib>:"Open Config Data.vi"("configuration file path"=w1575) -> ("error out"=w1571:errorcluster, "refnum"=w1572:T8)  [unwired: 8 in, 1 out]
        n1346 = call-poly <vilib>:"Write Key.vi"("section"="线程一数据重发功能", "error in (no error)"=w1571, "value"=w1566, "key"="重发功能", "refnum"=w1572) -> ("error out"=w1569:errorcluster, "refnum out"=w1570:T8)  [unwired: 4 in, 1 out]
        n1347 = call <vilib>:"Close Config Data.vi"("error in (no error)"=w1569, "refnum"=w1570) -> ()  [unwired: 8 in, 2 out]
      }
      event "重发日期": Value Change {
        n1348 = event-data() -> ()  [unwired: 1 in, 6 out]
        n1349 = call <vilib>:"Application Directory.vi"() -> ("Application Directory"=w1584:path)
        n1350 = Build Path(base path=w1584, name or relative path="data\\Set.ini" ("名称或相对路径")) -> (appended path=w1585:path)
        n1351 = local read "重发日期"() -> (w1576:T2)
        n1352 = call <vilib>:"Open Config Data.vi"("configuration file path"=w1585) -> ("error out"=w1581:errorcluster, "refnum"=w1582:T8)  [unwired: 8 in, 1 out]
        n1353 = call-poly <vilib>:"Write Key.vi"("section"="线程一数据重发功能", "error in (no error)"=w1581, "value"=w1576, "key"="重发日期", "refnum"=w1582) -> ("error out"=w1579:errorcluster, "refnum out"=w1580:T8)  [unwired: 4 in, 1 out]
        n1354 = call <vilib>:"Close Config Data.vi"("error in (no error)"=w1579, "refnum"=w1580) -> ()  [unwired: 8 in, 2 out]
      }
      event "重发时间": Value Change {
        n1355 = event-data() -> ()  [unwired: 1 in, 6 out]
        n1356 = call <vilib>:"Application Directory.vi"() -> ("Application Directory"=w1594:path)
        n1357 = Build Path(base path=w1594, name or relative path="data\\Set.ini" ("名称或相对路径")) -> (appended path=w1595:path)
        n1358 = local read "重发时间"() -> (w1586:T1)
        n1359 = call <vilib>:"Open Config Data.vi"("configuration file path"=w1595) -> ("error out"=w1591:errorcluster, "refnum"=w1592:T8)  [unwired: 8 in, 1 out]
        n1360 = call-poly <vilib>:"Write Key.vi"("section"="线程一数据重发功能", "error in (no error)"=w1591, "value"=w1586, "key"="重发时间", "refnum"=w1592) -> ("error out"=w1589:errorcluster, "refnum out"=w1590:T8)  [unwired: 4 in, 1 out]
        n1361 = call <vilib>:"Close Config Data.vi"("error in (no error)"=w1589, "refnum"=w1590) -> ()  [unwired: 8 in, 2 out]
      }
      event "确定更改起始时间": Value Change {
        n1362 = event-data() -> ()  [unwired: 1 in, 6 out]
        n1363 = local write "更改起始时间"(FALSE ("更改起始时间")) -> ()
        n1364 = Two Button Dialog(message="确定以当前设置时间作为数据索引起始时间？" ("消息")) -> (T button?=w1597:bool)  [unwired: 2 in]
        n1365 = case shown="真" w1597 {
          frame False {
          }
          frame True {
            n1366 = local read "参数数值"() -> (w1602:T5)
            n1367 = global write "断电保存全局.vi" "数据重发"(TRUE ("数据重发")) -> ()
            n1368 = Cluster To Array(cluster=w1602) -> (array=w1603:bool[])
            n1369 = for {
              tunnel: w1603 -> [_] mode=indexing
              tunnel: [w1613] -> w1601
              i -> [w1614]
              n1370 = Format Date/Time String(time format string (%c)="%Y/%m/%d %H:%M:%S" ("时间格式字符串(%c)"), seconds (now)="数据发送起始时间") -> (date/time string=w1613:string)  [unwired: 1 in]
              n1371 = global write "断电保存全局.vi" "数据重发时间戳"(w1613) -> ()
              n1372 = case shown="0, 默认" w1614 {
                tunnel: w1613 -> [w1617 w1618 w1619 w1620 w1621 w1622 w1623 w1624 w1625 w1626 w1627 w1628 w1629 w1630 w1631 w1632 w1633 w1634]
                frame 0, Default {
                  n1373 = global write "全局 水样时间.vi" "time1"(w1617) -> ()
                }
                frame 1 {
                  n1374 = global write "全局 水样时间.vi" "time2"(w1618) -> ()
                }
                frame 2 {
                  n1375 = global write "全局 水样时间.vi" "time3"(w1619) -> ()
                }
                frame 3 {
                  n1376 = global write "全局 水样时间.vi" "time4"(w1620) -> ()
                }
                frame 4 {
                  n1377 = global write "全局 水样时间.vi" "time5"(w1621) -> ()
                }
                frame 5 {
                  n1378 = global write "全局 水样时间.vi" "time6"(w1622) -> ()
                }
                frame 6 {
                  n1379 = global write "全局 水样时间.vi" "time7"(w1623) -> ()
                }
                frame 7 {
                  n1380 = global write "全局 水样时间.vi" "time8"(w1624) -> ()
                }
                frame 8 {
                  n1381 = global write "全局 水样时间.vi" "time9"(w1625) -> ()
                }
                frame 9 {
                  n1382 = global write "全局 水样时间.vi" "time10"(w1626) -> ()
                }
                frame 10 {
                  n1383 = global write "全局 水样时间.vi" "time11"(w1627) -> ()
                }
                frame 11 {
                  n1384 = global write "全局 水样时间.vi" "time12"(w1628) -> ()
                }
                frame 12 {
                  n1385 = global write "全局 水样时间.vi" "time13"(w1629) -> ()
                }
                frame 13 {
                  n1386 = global write "全局 水样时间.vi" "time14"(w1630) -> ()
                }
                frame 14 {
                  n1387 = global write "全局 水样时间.vi" "time15"(w1631) -> ()
                }
                frame 15 {
                  n1388 = global write "全局 水样时间.vi" "time16"(w1632) -> ()
                }
                frame 16 {
                  n1389 = global write "全局 水样时间.vi" "time17"(w1633) -> ()
                }
                frame 17 {
                  n1390 = global write "全局 水样时间.vi" "time18"(w1634) -> ()
                }
              }
            }
            n1391 = global read "断电保存全局.vi" "数据组合发送"() -> (w1599:bool)
            n1392 = case shown="真" w1599 {
              tunnel: w1601 -> [w1604 _]
              frame False {
                n1393 = global write "全局 时间2.vi" "跨度核查索引起始时间"(w1604) -> ()
                n1394 = global write "全局 时间2.vi" "标样核查索引起始时间"(w1604) -> ()
                n1395 = global write "全局 时间2.vi" "零点核查索引起始时间"(w1604) -> ()
                n1396 = global write "全局 时间2.vi" "加标回收索引起始时间"(w1604) -> ()
                n1397 = for {
                  N: 5 -> [_]
                  tunnel: w1604 -> [w1606]
                  i -> [w1607]
                  n1398 = case shown="4" w1607 {
                    tunnel: w1606 -> [w1608 w1609 w1610 w1611 w1612]
                    frame 0, Default {
                      n1399 = global write "全局 时间2.vi" "氨氮跨度核查索引起始时间"(w1608) -> ()
                      n1400 = global write "全局 时间2.vi" "氨氮零点核查索引起始时间"(w1608) -> ()
                    }
                    frame 1 {
                      n1401 = global write "全局 时间2.vi" "总氮跨度核查索引起始时间"(w1609) -> ()
                      n1402 = global write "全局 时间2.vi" "总氮零点核查索引起始时间"(w1609) -> ()
                    }
                    frame 2 {
                      n1403 = global write "全局 时间2.vi" "总磷跨度核查索引起始时间"(w1610) -> ()
                      n1404 = global write "全局 时间2.vi" "总磷零点核查索引起始时间"(w1610) -> ()
                    }
                    frame 3 {
                      n1405 = global write "全局 时间2.vi" "CODMn跨度核查索引起始时间"(w1611) -> ()
                      n1406 = global write "全局 时间2.vi" "CODMn零点核查索引起始时间"(w1611) -> ()
                    }
                    frame 4 {
                      n1407 = global write "全局 时间2.vi" "CODCr跨度核查索引起始时间"(w1612) -> ()
                      n1408 = global write "全局 时间2.vi" "CODCr零点核查索引起始时间"(w1612) -> ()
                    }
                  }
                }
              }
              frame True {
              }
            }
          }
        }
      }
      event "开机启动": Value Change {
        n1409 = event-data() -> ("NewVal"=w1635:bool)  [unwired: 1 in, 5 out]
        n1410 = case shown="假" w1635 {
          frame False {
            n1411 = Two Button Dialog(message="是否删除开机启动" ("消息"), 1:"否" ("F按钮名称（“取消”）"), 2:"是" ("T按钮名称（“确定”）")) -> (T button?=w1636:bool)
            n1412 = case shown="真" w1636 {
              frame False {
              }
              frame True {
                n1413 = call <vilib>:"Application Directory.vi"() -> ("Application Directory"=w1641:path)
                n1414 = call "删除启动项.vi"("启动文件路径"=w1641) -> ("删除标记"=w1640:bool)  [unwired: 9 in, 1 out]
                n1415 = case shown="假" w1640 {
                  tunnel: ["删除开机启动失败" ("T按钮名称（“确定”）") "删除开机启动成功" ("T按钮名称（“确定”）")] -> w1642
                  frame False {
                  }
                  frame True {
                  }
                }
                n1416 = One Button Dialog(message=w1642) -> ()  [unwired: 1 in, 1 out]
              }
            }
          }
          frame True {
            n1417 = Two Button Dialog(message="是否添加开机启动" ("消息"), 1:"否" ("F按钮名称（“取消”）"), 2:"是" ("T按钮名称（“确定”）")) -> (T button?=w1645:bool)
            n1418 = case shown="真" w1645 {
              frame False {
              }
              frame True {
                n1419 = call <vilib>:"Application Directory.vi"() -> ("Application Directory"=w1651:path)
                n1420 = call "添加启动项.vi"("启动文件路径"=w1651) -> ("添加成功标记"=w1650:bool)  [unwired: 9 in, 1 out]
                n1421 = case shown="真" w1650 {
                  tunnel: ["添加开机启动失败" ("T按钮名称（“确定”）") "添加开机启动成功" ("T按钮名称（“确定”）")] -> w1649
                  frame False {
                  }
                  frame True {
                  }
                }
                n1422 = One Button Dialog(message=w1649) -> ()  [unwired: 1 in, 1 out]
              }
            }
          }
        }
      }
      event "IP": Mouse Down {
        n1423 = event-data() -> ("CtlRef"=w1654:refnum<vi>)  [unwired: 1 in, 5 out]
        n1424 = property class="Str" props=["Value"](reference=w1654) -> ()  [unwired: 1 in, 3 out]
        n1425 = local read "IP"() -> (w1656:string)
        n1426 = call "IP键盘.vi"("OldNumber"=w1656) -> ("NewNumber"=w1655:string)
        n1427 = local write "IP"(w1655) -> ()
      }
      event "PORT": Mouse Down {
        n1428 = event-data() -> ()  [unwired: 1 in, 6 out]
        n1429 = local read "PORT"() -> (w1658:string)
        n1430 = call "IP键盘.vi"("OldNumber"=w1658) -> ("NewNumber"=w1657:string)
        n1431 = local write "PORT"(w1657) -> ()
      }
      event "查询质控数据起始时间": Value Change {
        n1432 = event-data() -> ()  [unwired: 1 in, 6 out]
        n1433 = property on="窗格" class="Pane"("Origin"=T11 {"Horizontal"=1000, "Vertical"=0} ("原点")) -> ()  [unwired: 2 in, 2 out]
      }
      event "返回主界面": Value Change {
        n1434 = event-data() -> ()  [unwired: 1 in, 6 out]
        n1435 = property on="窗格" class="Pane"("Origin"=T11 {"Horizontal"=0, "Vertical"=0} ("原点")) -> ()  [unwired: 2 in, 2 out]
      }
    }
  }
  n1436 = while {
    stop <- FALSE stop-if-true
    # "心跳包"
    n1437 = global read "全局 数据发送重叠.vi" "掉线指示灯"() -> (→"掉线指示":bool)
    n1438 = Get Date/Time In Seconds() -> (seconds since 1Jan1904=w1702:timestamp)
    n1439 = local read "数据发送通道"() -> (w1677:enum16{"TCP", "VISA"})
    n1440 = local read "空闲时间"() -> (w1694:dbl)
    n1441 = case shown="\"VISA\"" "数据发送通道" {
      tunnel: [w1734 w1737] -> w1681
      tunnel: [w1733 w1735] -> w1680
      frame "TCP", Default {
        n1442 = local read "PORT"() -> (w1733:string)
        n1443 = local read "IP"() -> (w1734:string)
      }
      frame "VISA" {
        n1444 = local read "baud rate"() -> (w1736:u32)
        n1445 = local read "VISA resource name"() -> (w1737:refnum<visa-resource-name>)
        n1446 = Number To Decimal String(number=w1736) -> (decimal integer string=w1735:string)  [unwired: 1 in]
      }
    }
    n1447 = Wait (ms)(milliseconds to wait=u32 1000 ("等待时间（毫秒）")) -> ()  [unwired: 1 out]
    n1448 = global read "全局 数据发送重叠.vi" "主动上报数据中"() -> (w1661:bool)
    n1449 = local read "核查数据上传"() -> (w1689:bool)
    n1450 = local read "空闲时间"() -> (w1725:dbl)
    n1451 = local read "查询数据发送"() -> (w1692:bool)
    n1452 = Number To Decimal String(number=w1694) -> (decimal integer string=→"空闲时间/s":string)  [unwired: 1 in]
    n1453 = local read "站点设备"() -> (w1682:string)
    n1454 = local read "站点名称"() -> (w1683:string)
    n1455 = global read "全局 数据发送重叠.vi" "数据接收超时指示灯"() -> (→"数据接收超时指示灯":bool)
    n1456 = local read "MN"() -> (w1679:string)
    n1457 = Format Date/Time String(time format string (%c)="%Y/%m/%d %H:%M:%S" ("时间格式字符串(%c)"), seconds (now)=w1702) -> (date/time string=→"系统时间":string)  [unwired: 1 in]
    n1458 = local read "PW"() -> (w1678:string)
    n1459 = local read "步骤"() -> (w1719:T6)
    n1460 = case shown="\"TCP\", 默认" w1677 {
      frame "TCP", Default {
        w1738 = TRUE ("可见")
        w1739 = FALSE ("可见")
        n1461 = property on="VISA resource name" class="VISAName"("Visible"=w1739) -> ()  [unwired: 2 in, 2 out]
        n1462 = property on="baud rate" class="DigNum (严格)"("Visible"=w1739) -> ()  [unwired: 2 in, 2 out]
        n1463 = property on="IP" class="Str"("Visible"=w1738) -> ()  [unwired: 2 in, 2 out]
        n1464 = property on="PORT" class="Str"("Visible"=w1738) -> ()  [unwired: 2 in, 2 out]
      }
      frame "VISA" {
        w1740 = TRUE ("可见")
        w1741 = FALSE ("可见")
        n1465 = property on="baud rate" class="DigNum (严格)"("Visible"=w1740) -> ()  [unwired: 2 in, 2 out]
        n1466 = property on="VISA resource name" class="VISAName"("Visible"=w1740) -> ()  [unwired: 2 in, 2 out]
        n1467 = property on="IP" class="Str"("Visible"=w1741) -> ()  [unwired: 2 in, 2 out]
        n1468 = property on="PORT" class="Str"("Visible"=w1741) -> ()  [unwired: 2 in, 2 out]
      }
    }
    n1469 = local read "数据发送协议"() -> (w1674:enum16{"2005-212协议", "2017-212协议"})
    n1470 = Not(x=w1689) -> (.not. x?=w1690:bool)
    n1471 = Greater?(x=w1725, y=30.0) -> (0:w1723:bool)
    n1472 = Not(x=w1661) -> (.not. x?=w1691:bool)
    n1473 = property on="数据发送通道" class="Enum (严格)"("Visible"="锁") -> ()  [unwired: 2 in, 2 out]
    n1474 = Not(x=w1692) -> (.not. x?=w1713:bool)
    n1475 = Equal?(x=w1719, y=T6."读取数据" ("步骤")) -> (x = y?=w1717:bool)
    n1476 = Bundle By Name(cluster=T4 {"站点"="", "设备"="", "IP"="", "PORT"="", "MN"="", "PW"=""} ("配置信息"), "站点"=w1683, "设备"=w1682, "IP"=w1681, "PORT"=w1680, "MN"=w1679, "PW"=w1678) -> (→"配置信息":T4)
    n1477 = Select(t=T12."Enabled" ("禁用"), s="更改起始时间", f=T12."Disabled and Grayed Out" ("禁用")) -> (s? t:f=w1705:T12)
    n1478 = case shown="真" w1723 {
      tunnel: w1723 -> [_ w1751]
      tunnel: [FALSE w1751] -> w1720
      frame False {
      }
      frame True {
        n1479 = local read "QN"() -> (w1749:string)
        n1480 = local write "空闲时间"(0.0 ("空闲时间")) -> ()
        n1481 = local read "MN"() -> (w1748:string)
        n1482 = local read "PW"() -> (w1747:string)
        n1483 = local read "数据发送通道"() -> (w1746:enum16{"TCP", "VISA"})
        n1484 = call "数据编码.vi"("table输入"="心跳包", "QN"=w1749, "MN"=w1748, "PW"=w1747) -> ("通讯包字符串"=w1744:string)  [unwired: 10 in, 1 out]
        n1485 = local write "发送报文显示"(w1744) -> ()
        n1486 = call "VISATCP组合选择发送.vi"("数据发送通道"=w1746, "命令"="write", "写入缓冲区"=w1744) -> ("错误输出"=w1743:errorcluster)  [unwired: 9 in, 3 out]
        n1487 = call <vilib>:"Clear Errors.vi"("error in (no error)"=w1743) -> ()  [unwired: 5 in, 2 out]
      }
    }
    "心跳包" <- w1720
    n1488 = Select(t=T12."Enabled" ("禁用"), s="锁", f=T12."Disabled and Grayed Out" ("禁用")) -> (s? t:f=w1666:T12)
    n1489 = property on="数据发送起始时间" class="AbsTime (严格)"("DisabledEnum"=w1705) -> ()  [unwired: 2 in, 2 out]
    n1490 = global read "全局 时间2.vi" "跨度核查索引起始时间"() -> (→"跨度核查索引起始时间":string)
    n1491 = case shown="\"2017-212协议\", 默认" w1674 {
      tunnel: ["32" ("设备编码MN") w1728] -> w1711
      frame "2005-212协议" {
      }
      frame "2017-212协议", Default {
        n1492 = local read "系统编码选择框"() -> (w1729:string)
        n1493 = case shown="\"地表水质量监测\", 默认" w1729 {
          tunnel: ["52" ("设备编码MN") "32" ("设备编码MN") "21" ("设备编码MN")] -> w1728
          frame "污水排放过程监测" {
          }
          frame "地表水体污染源" {
          }
          frame "地表水质量监测", Default {
          }
        }
      }
    }
    n1494 = global read "全局 时间2.vi" "标样核查索引起始时间"() -> (→"标样核查索引起始时间":string)
    n1495 = global read "全局 时间2.vi" "零点核查索引起始时间"() -> (→"零点核查索引起始时间":string)
    n1496 = global read "全局 时间2.vi" "加标回收索引起始时间"() -> (→"加标回收索引起始时间":string)
    n1497 = property on="设置超时时间/min" class="DigNum (严格)"("DisabledEnum"=w1666) -> ()  [unwired: 2 in, 2 out]
    n1498 = property on="IP" class="Str"("DisabledEnum"=w1666) -> ()  [unwired: 2 in, 2 out]
    n1499 = property on="每周自动重发" class="Bool (严格)"("DisabledEnum"=w1666) -> ()  [unwired: 2 in, 2 out]
    n1500 = property on="PORT" class="Str"("DisabledEnum"=w1666) -> ()  [unwired: 2 in, 2 out]
    n1501 = local read "数据发送协议"() -> (w1673:enum16{"2005-212协议", "2017-212协议"})
    n1502 = local read "TCP服务端掉线计数"() -> (w1697:i32)
    n1503 = local read "1st Error to Convert"() -> (w1700:i32)
    n1504 = local read "TCP掉线时间节点"() -> (w1696:string)
    n1505 = property on="确定更改起始时间" class="Bool"("DisabledEnum"=w1705) -> ()  [unwired: 2 in, 2 out]
    n1506 = property on="MN" class="Str"("DisabledEnum"=w1666) -> ()  [unwired: 2 in, 2 out]
    n1507 = property on="PW" class="Str"("DisabledEnum"=w1666) -> ()  [unwired: 2 in, 2 out]
    n1508 = property on="实时数据发送时间间隔/min" class="DigNum (严格)"("DisabledEnum"=w1666) -> ()  [unwired: 2 in, 2 out]
    n1509 = local read "元素"() -> (w1698:string)
    n1510 = local read "步骤"() -> (w1699:T6)
    n1511 = Equal?(x=w1673, y=enum16{"2005-212协议", "2017-212协议"}."2017-212协议" ("数据发送协议")) -> (x = y?=w1671:bool)
    n1512 = Compound Arithmetic op=AND ("复合运算")(w1671, w1717, w1713, w1691, w1690) -> (w1714:bool)
    n1513 = case shown="真" w1714 {
      frame False {
      }
      frame True {
        n1514 = local read "空闲时间"() -> (w1754:dbl)
        n1515 = Increment(x=w1754) -> (x+1=→"空闲时间":dbl)
      }
    }
    n1516 = property on="数据发送通道" class="Enum (严格)"("DisabledEnum"=w1666) -> ()  [unwired: 2 in, 2 out]
    n1517 = Bundle By Name(cluster=T3 {"1st Error to Convert "=54, "步骤 "=enum."打开连接", "元素"="实时数据", "TCP服务端掉线计数"=4, "TCP掉线时间节点"="2019/05/08 15:24:17"} ("状态信息"), "1st Error to Convert"=w1700, "步骤"=w1699, "元素"=w1698, "TCP服务端掉线计数"=w1697, "TCP掉线时间节点"=w1696) -> (→"状态信息":T3)
    n1518 = global read "全局1.vi" "通讯包字符串"() -> (w1662:string)
    n1519 = property on="重发时间" class="Enum (严格)"("DisabledEnum"=w1666) -> ()  [unwired: 2 in, 2 out]
    n1520 = property on="重发日期" class="Enum (严格)"("DisabledEnum"=w1666) -> ()  [unwired: 2 in, 2 out]
    n1521 = property on="VISA resource name" class="VISAName"("DisabledEnum"=w1666) -> ()  [unwired: 2 in, 2 out]
    n1522 = property on="判断数据反馈" class="Bool (严格)"("DisabledEnum"=w1666) -> ()  [unwired: 2 in, 2 out]
    n1523 = property on="baud rate" class="DigNum (严格)"("DisabledEnum"=w1666) -> ()  [unwired: 2 in, 2 out]
    n1524 = property on="数据发送协议" class="Enum (严格)"("DisabledEnum"=w1666) -> ()  [unwired: 2 in, 2 out]
    n1525 = property on="2011发送" class="Bool (严格)"("DisabledEnum"=w1666) -> ()  [unwired: 2 in, 2 out]
    n1526 = feedback #1(w1662) -> (w1663:string)
    n1527 = feedback-in #1(w1662) -> ()
    n1528 = global write "全局1.vi" "系统编码ST"(w1711) -> ()
    n1529 = property on="日志、参数发送" class="Bool (严格)"("DisabledEnum"=w1666) -> ()  [unwired: 2 in, 2 out]
    n1530 = property on="数据组合发送" class="Bool (严格)"("DisabledEnum"=w1666) -> ()  [unwired: 2 in, 2 out]
    n1531 = Not Equal?(x=w1662, y=w1663) -> (x != y?=w1664:bool)
    n1532 = case shown="真" w1664 {
      tunnel: w1662 -> [_ w1726]
      frame False {
      }
      frame True {
        n1533 = local write "发送报文显示"(w1726) -> ()
      }
    }
    n1534 = global read "断电保存全局.vi" "日志、参数发送"() -> (w1667:bool)
    n1535 = global read "断电保存全局.vi" "数据组合发送"() -> (w1665:bool)
    n1536 = global read "断电保存全局.vi" "判断数据反馈"() -> (w1669:bool)
    n1537 = local read "数据发送协议"() -> (w1670:enum16{"2005-212协议", "2017-212协议"})
    n1538 = global read "断电保存全局.vi" "2011发送"() -> (w1668:bool)
    n1539 = local write "日志、参数发送"(w1667) -> ()
    n1540 = local write "数据组合发送"(w1665) -> ()
    n1541 = local write "判断数据反馈"(w1669) -> ()
    n1542 = global write "全局1.vi" "数据发送版本"(w1670) -> ()
    n1543 = local write "2011发送"(w1668) -> ()
  }
  n1544 = for {
    N: 1 -> [_]
    w1768 = "数据发送协议"
    w1775 = "线程一自主部署站点保存"
    w1791 = "数据发送通道" ("section")
    (unwired) path "C:/LabVIEW Project/builds/平台数据发送系统" ("Application Directory")
    w1842 = "" ("参数")
    w1803 = FALSE ("数据发送中断")
    w1813 = 0 ("数值")
    # "版本改动:增加了远程反控命令，和仪器端双向通讯，modbus TCP读写"
    # "ST参数选择"
    # "初始化"
    n1545 = property class="VI"() -> ("Panel"=w1846:refnum<vi>)  [unwired: 2 in, 2 out]
    n1546 = local write "核查数据上传"(w1803) -> ()
    n1547 = global write "全局 实时数据参数.vi" "参数"(w1842) -> ()
    n1548 = local write "心跳包"(w1803) -> ()
    n1549 = local write "查询数据发送"(w1803) -> ()
    n1550 = local write "实时小时数据上传"(w1803) -> ()
    n1551 = local write "系统状态改变"(w1803) -> ()
    n1552 = global write "全局 小时数据发送次数.vi" "小时数据发送次数"(w1813) -> ()
    n1553 = local write "重发数据"(w1803) -> ()
    n1554 = property class="Pnl"(reference=w1846) -> ("Panes[]"=w1845:refnum<vi>[])  [unwired: 1 in, 2 out]
    n1555 = global write "全局 实时数据参数.vi" "data"(string[][] [] ("data")) -> ()
    n1556 = property on="窗格" class="Pane"("Origin"=T11 {"Horizontal"=0, "Vertical"=0} ("原点")) -> ()  [unwired: 2 in, 2 out]
    n1557 = local write "空闲时间"(0.0 ("try")) -> ()
    n1558 = global write "全局1.vi" "枚举"(enum16{"返回请求应答", "上传数据", "返回执行结果"}."返回请求应答" ("枚举")) -> ()
    n1559 = global write "全局 实时数据参数.vi" "连接的字符串"(w1842) -> ()
    n1560 = call <vilib>:"Application Directory.vi"() -> ("Application Directory"=w1840:path)
    n1561 = for {
      tunnel: w1845 -> [w1857] mode=indexing
      tunnel: u32 15592941 ("窗格颜色") -> [w1858]
      n1562 = property class="Pane"(reference=w1857, "PaneColor"=w1858) -> ()  [unwired: 1 in, 2 out]
    }
    n1563 = Build Path(base path=w1840, name or relative path="data\\Set.ini" ("名称或相对路径")) -> (appended path=w1838:path)
    n1564 = call <vilib>:"Open Config Data.vi"("configuration file path"=w1838) -> ("error out"=w1836:errorcluster, "refnum"=w1837:T8)  [unwired: 8 in, 1 out]
    n1565 = call <vilib>:"Application Directory.vi"() -> ("Application Directory"=w1802:path)
    n1566 = call-poly <vilib>:"Read Key.vi"("section"=w1775, "error in (no error)"=w1836, "key"="站点名称", "refnum"=w1837) -> ("error out"=w1833:errorcluster, "value"=w1789:string, "refnum out"=w1834:T8)  [unwired: 4 in, 1 out]
    n1567 = call <vilib>:"Application Directory.vi"() -> ("Application Directory"=w1758:path)
    n1568 = call <vilib>:"Application Directory.vi"() -> ("Application Directory"=w1798:path)
    n1569 = call <vilib>:"Recursive File List.vi"("pattern"="*.exe", "Folder Path"=w1802) -> ("All Files in Dir"=w1811:path[])  [unwired: 5 in, 4 out]
    n1570 = Build Path(base path=w1758, name or relative path="data\\sys.ini" ("名称或相对路径")) -> (appended path=w1756:path)
    n1571 = local write "站点名称"(w1789) -> ()
    n1572 = Build Path(base path=w1798, name or relative path="data\\background.jpg" ("名称或相对路径")) -> (appended path=w1797:path)
    n1573 = call <vilib>:"Open Config Data.vi"("configuration file path"=w1756) -> ("error out"=w1762:errorcluster, "refnum"=w1761:T8)  [unwired: 8 in, 1 out]
    n1574 = Index Array(array=w1811) -> (element=w1810:path)  [unwired: 1 in]
    n1575 = Get Date/Time In Seconds() -> (seconds since 1Jan1904=w1850:timestamp)
    n1576 = call <vilib>:"Read JPEG File.vi"("path to JPEG file"=w1797) -> ("error out"=w1795:errorcluster, "image data"=w1796:T13)  [unwired: 8 in, 1 out]
    n1577 = vi-ref "断电保存全局.vi"() -> (w1760:refnum<vi>)
    n1578 = Format Date/Time String(time format string (%c)="%Y%m%d%H%M%S%3u" ("时间格式字符串(%c)"), seconds (now)=w1850) -> (date/time string=w1849:string)  [unwired: 1 in]
    n1579 = call-poly <vilib>:"Read Key.vi"("section"=w1775, "error in (no error)"=w1833, "key"="站点设备", "refnum"=w1834) -> ("error out"=w1830:errorcluster, "value"=w1788:string, "refnum out"=w1831:T8)  [unwired: 4 in, 1 out]
    n1580 = File/Directory Info(path=w1810) -> (last mod=w1809:timestamp)  [unwired: 1 in, 6 out]
    n1581 = call <vilib>:"FileVersionInfo.vi"("Application Path in"=w1810) -> ("error out"=w1794:errorcluster, "File Version Info"=w1806:string)  [unwired: 7 in, 2 out]
    n1582 = call <userlib>:"Read Panel from INI__ogtk.vi"("error in (no error)"=w1762, "VI ref"=w1760, "refnum"=w1761) -> ("error out"=w1755:errorcluster, "refnum out"=w1759:T8)  [unwired: 7 in]
    n1583 = property on="窗格" class="Pane"("BackgroundImage"=w1796) -> ()  [unwired: 2 in, 2 out]
    n1584 = Format Date/Time String(time format string (%c)="\n%Y%m%d%H%M" ("时间格式字符串(%c)"), seconds (now)=w1809) -> (date/time string=w1805:string)  [unwired: 1 in]
    n1585 = local write "站点设备"(w1788) -> ()
    n1586 = case shown="错误" w1755 {
      frame No Error {
      }
      frame Error {
        n1587 = global write "断电保存全局.vi" "判断数据反馈"(TRUE ("判断数据反馈")) -> ()
      }
    }
    n1588 = Search and Replace String(input string=w1849, search string="." ("搜索字符串")) -> (result string=w1847:string)  [unwired: 6 in, 3 out]
    n1589 = call <vilib>:"Close Config Data.vi"("error in (no error)"=w1755, "refnum"=w1759) -> ()  [unwired: 8 in, 2 out]
    n1590 = call-poly <vilib>:"Read Key.vi"("section"=w1775, "error in (no error)"=w1830, "key"="IP", "refnum"=w1831) -> ("error out"=w1827:errorcluster, "value"=w1787:string, "refnum out"=w1828:T8)  [unwired: 4 in, 1 out]
    n1591 = Concatenate Strings("V" ("字符串"), w1806, w1805) -> (→"软件版本":string)
    n1592 = local write "QN"(w1847) -> ()
    n1593 = call <vilib>:"Simple Error Handler.vi"("error in (no error)"=w1794) -> ()  [unwired: 4 in, 5 out]
    n1594 = call <vilib>:"Simple Error Handler.vi"("error in (no error)"=w1795) -> ()  [unwired: 4 in, 5 out]
    n1595 = local write "IP"(w1787) -> ()
    n1596 = call-poly <vilib>:"Read Key.vi"("section"=w1775, "error in (no error)"=w1827, "key"="PORT", "refnum"=w1828) -> ("error out"=w1823:errorcluster, "value"=w1786:string, "refnum out"=w1824:T8)  [unwired: 4 in, 1 out]
    n1597 = call <vilib>:"Application Directory.vi"() -> ("Application Directory"=w1801:path)
    n1598 = local write "PORT"(w1786) -> ()
    n1599 = call "查询启动项.vi"("启动文件路径"=w1801) -> ("包含启动项"=w1800:bool)  [unwired: 9 in, 1 out]
    n1600 = call-poly <vilib>:"Read Key.vi"("section"=w1775, "error in (no error)"=w1823, "key"="MN", "refnum"=w1824) -> ("error out"=w1782:errorcluster, "value"=w1785:string, "refnum out"=w1783:T8)  [unwired: 4 in, 1 out]
    n1601 = local write "MN"(w1785) -> ()
    n1602 = local write "开机启动"(w1800) -> ()
    n1603 = call-poly <vilib>:"Read Key.vi"("section"=w1775, "error in (no error)"=w1782, "key"="PW", "refnum"=w1783) -> ("error out"=w1780:errorcluster, "value"=w1784:string, "refnum out"=w1781:T8)  [unwired: 4 in, 1 out]
    n1604 = local write "PW"(w1784) -> ()
    n1605 = call-poly <vilib>:"Read Key.vi"("section"=w1775, "error in (no error)"=w1780, "key"="VISA", "refnum"=w1781) -> ("error out"=w1776:errorcluster, "value"=w1778:string, "refnum out"=w1777:T8)  [unwired: 4 in, 1 out]
    n1606 = local write "VISA resource name"(w1778) -> ()
    n1607 = call-poly <vilib>:"Read Key.vi"("section"=w1775, "error in (no error)"=w1776, "key"="BAUDRATE", "refnum"=w1777) -> ("error out"=w1771:errorcluster, "value"=w1773:i32, "refnum out"=w1772:T8)  [unwired: 4 in, 1 out]
    n1608 = local write "baud rate"(w1773) -> ()
    n1609 = call-poly <vilib>:"Read Key.vi"("section"="系统编码选择", "error in (no error)"=w1771, "key"="系统编码", "refnum"=w1772) -> ("error out"=w1817:errorcluster, "value"=w1819:string, "refnum out"=w1818:T8)  [unwired: 4 in, 1 out]
    n1610 = local write "系统编码选择框"(w1819) -> ()
    n1611 = call-poly <vilib>:"Read Key.vi"("section"="掉线时间存储", "error in (no error)"=w1817, "key"="掉线时间", "refnum"=w1818) -> ("error out"=w1792:errorcluster, "value"=w1814:string, "refnum out"=w1793:T8)  [unwired: 4 in, 1 out]
    n1612 = global write "全局 数据发送重叠.vi" "TCP掉线时间节点"(w1814) -> ()
    n1613 = local write "TCP掉线时间节点"(w1814) -> ()
    n1614 = call-poly <vilib>:"Read Key.vi"("section"=w1791, "error in (no error)"=w1792, "key"=w1791, "refnum"=w1793) -> ("error out"=w1769:errorcluster, "value"=w1790:i32, "refnum out"=w1770:T8)  [unwired: 4 in, 1 out]
    n1615 = local write "数据发送通道"(w1790) -> ()
    n1616 = call-poly <vilib>:"Read Key.vi"("section"=w1768, "error in (no error)"=w1769, "key"=w1768, "refnum"=w1770) -> ("error out"=w1766:errorcluster, "value"=w1764:i32, "found?"=w1765:bool, "refnum out"=w1767:T8)  [unwired: 4 in]
    n1617 = case shown="假" w1765 {
      tunnel: w1764 -> [_ w1856]
      tunnel: [1 ("value") w1856] -> w1763
      frame False {
      }
      frame True {
      }
    }
    n1618 = local write "数据发送协议"(w1763) -> ()
    n1619 = call <vilib>:"Close Config Data.vi"("error in (no error)"=w1766, "refnum"=w1767) -> ()  [unwired: 8 in, 2 out]
    "TCP服务端掉线计数" <- w1813
  }
  n1620 = property class="App"() -> ("App.Kind"=w31:T14)  [unwired: 2 in, 2 out]
  n1621 = case shown="\"Development System\", 默认" w31 {
    tunnel: [T15."Standard" ("状态") T15."Hidden" ("状态")] -> w3
    frame "Development System", Default {
    }
    frame "Run Time System" {
    }
  }
  n1622 = call "获取需发送的数据表.vi"() -> ("error out"=w42:errorcluster, "tables"=w51:string[])  [unwired: 10 in]
  n1623 = call <vilib>:"Clear Errors.vi"("error in (no error)"=w42) -> ()  [unwired: 5 in, 2 out]
  n1624 = call <vilib>:"Application Directory.vi"() -> ("Application Directory"=w25:path)
  n1625 = Build Path(base path=w25, name or relative path="data\\tubiao.ico" ("名称或相对路径")) -> (appended path=w15:path)
  n1626 = Insert Into Array(array=w51, index=0 ("索引"), new element="实时数据" ("新元素/子数组")) -> (w52:string[])
  n1627 = Current VI's Path() -> (path=w28:path)
  n1628 = Build Array(w15) -> (w20:path[])
  n1629 = Open VI Reference(vi path=w28) -> (vi reference=w29:refnum<vi>)  [unwired: 5 in, 1 out]
  n1630 = Array Size(array=w52) -> (size(s)=w49:i32)
  n1631 = invoke class="VI" method="FP.Open"(reference=w29, "Activate"=TRUE ("激活？"), "State"=w3) -> (error out=w30:errorcluster)  [unwired: 2 in, 4 out]
  n1632 = call <vilib>:"Constructor.vi"("error in"=w30, "IconFilePathList"=w20) -> ("error out"=w16:errorcluster, "NotifyIcon"=w24:refnum<class "NotifyIcon.lvclass">)  [unwired: 8 in]
  n1633 = Obtain Queue(name (unnamed)="STEP" ("名称（未命名）"), element data type=T6."初始化" ("枚举")) -> (queue out=w47:refnum<queue>)  [unwired: 3 in, 2 out]
  n1634 = for {
    shift-right: [w1865] -> w1
    shift-left: w16 -> [w1866]
    tunnel: string[] ["Open线程一", "-", "Exit线程一"] -> [w1864] mode=indexing
    tunnel: w23 -> [w1863] mode=indexing
    shift-right: [w1861] -> w2
    shift-left: w24 -> [w1862]
    # "2."
    n1635 = call <vilib>:"InsertMenuItem.vi"("error in"=w1866, "ItemTag"=w1863, "ItemName"=w1864, "NotifyIcon in"=w1862) -> ("error out"=w1865:errorcluster, "NotifyIcon out"=w1861:refnum<class "NotifyIcon.lvclass">)  [unwired: 6 in]
  }
  n1636 = Index Array(array=w23) -> (element=w22:string)  [unwired: 1 in]
  n1637 = Enqueue Element(queue=w47, element=T6."初始化" ("元素")) -> (queue out=w55:refnum<queue>)  [unwired: 2 in, 2 out]
  "主队列输出" <- w55
  n1638 = property class="NotifyIcon"(reference=w2, error in=w1, "Public:Visible"=TRUE ("Visible"), "Public:DefaultMenuItem"=w22, "Public:TipText"="平台发送系统线程一" ("TipText")) -> (reference out=w7:refnum<class "NotifyIcon.lvclass">, error out=w17:errorcluster, "Public:SelectedItemEvent"=w18:refnum<user-event>)
  n1639 = while {
    shift-right: [w1867] -> _
    shift-left: errorcluster {"status"=FALSE, "code"=0, "source"=""} ("error out") -> [w1879]
    shift-right: [w1876] -> _
    shift-left: _ -> [w1875]
    tunnel: w55 -> [w1878]
    tunnel: w52 -> [w1874]
    shift-right: [w1872] -> _
    shift-left: 0 ("索引") -> [w1873]
    tunnel: w49 -> [w1871]
    shift-right: [w1869] -> _
    shift-left: 0 ("索引") -> [w1870]
    stop <- FALSE stop-if-true
    n1640 = Wait (ms)(milliseconds to wait=u32 300 ("等待时间（毫秒）")) -> ()  [unwired: 1 out]
    n1641 = case shown="无错误" w1879 {
      selector: w1879 -> [w1897 w2643]
      tunnel: [w1880 w2646] -> w1867
      tunnel: w1878 -> [w1896 w2641]
      tunnel: [w1881 w2645] -> w1876
      tunnel: w1875 -> [w1893 w2645]
      tunnel: w1874 -> [w1892 _]
      tunnel: w1873 -> [w1887 w2644]
      tunnel: [w1890 w2644] -> w1872
      tunnel: w1871 -> [w1889 _]
      tunnel: w1870 -> [w1884 w2640]
      tunnel: [w1883 w2640] -> w1869
      frame No Error {
        n1642 = Less?(x=w1887, y=w1889) -> (x < y?=w1888:bool)
        n1643 = Dequeue Element(queue=w1896) -> (queue out=w1894:refnum<queue>, element=w1895:T6)  [unwired: 2 in, 2 out]
        "步骤" <- w1895
        n1644 = Select(t=w1887, s=w1888, f=0) -> (s? t:f=w1886:i32)
        n1645 = local read "元素"() -> (w1882:string)
        n1646 = Index Array(array=w1892, index=w1886) -> (element=→"元素":string)
        n1647 = case shown="\"读取数据\"" w1895 {
          tunnel: w1897 -> [w1904 _ w1929 w2072 w2555 w2637]
          tunnel: w1894 -> [w1900 w1918 w1924 w2082 w2553 w2635]
          tunnel: [w1904 w1906 w1929 w2070 w2552 w2637] -> w1880
          tunnel: [string[] [] ("待发送第一条数据") w1920 w1923 w2103 w2556 _] -> w1881
          tunnel: w1893 -> [_ w1920 _ w2103 w2556 w2636]
          tunnel: w1882 -> [_ _ _ _ _ w2630]
          tunnel: w1886 -> [w1901 w1917 w1928 w2104 w2557 w2626]
          tunnel: [w1901 w1917 w1927 w2104 w2557 w2627] -> w1890
          tunnel: w1884 -> [w1898 w1915 w1926 _ w2548 w2624]
          tunnel: [w1898 w1915 w1926 0 ("索引") w2551 w2624] -> w1883
          frame "初始化", Default {
            n1648 = Enqueue Element(queue=w1900, element=T6."打开连接" ("元素"), timeout in ms (-1)=1000 ("超时毫秒(-1)")) -> ()  [unwired: 1 in, 3 out]
          }
          frame "打开连接" {
            (unwired) "47.98.43.76"
            # "和时通数据接入平台端接收IP端口号，61.191.22.195:10003。"
            # "47.98.43.76:6666"
            n1649 = Enqueue Element(queue=w1918, element=T6."表格比对" ("元素"), timeout in ms (-1)=1000 ("超时毫秒(-1)")) -> ()  [unwired: 1 in, 3 out]
            n1650 = local read "数据发送通道"() -> (w1905:enum16{"TCP", "VISA"})
            n1651 = call "VISATCP组合选择发送.vi"("IP"="IP", "数据发送通道"=w1905, "命令"="open", "PORT"="PORT", "VISA resource name"="VISA resource name", "baud rate"="baud rate") -> ("错误输出"=w1906:errorcluster)  [unwired: 6 in, 3 out]
            n1652 = Unbundle By Name(w1906) -> ("status"=w1914:bool, "code"=→"1st Error to Convert":i32)
            n1653 = Not(x=w1914) -> (.not. x?=→"通信状态":bool)
          }
          frame "表格比对" {
            # "在发送数据完之后通过TCP掉线计数仍然大于1且列队中还有元素判定再次回到表格对比\n再在表格对比这里加上出列队（前提先一次把水样测试、核查等5个元素入列队）...........LOOP直到5种测量数据全部发送完毕"
            n1654 = disable-structure shown="禁用" {
              disable-tunnel: [w1931 _] -> _
              frame Disabled {
                n1655 = local read "TCP服务端掉线计数"() -> (w1933:i32)
                n1656 = Greater Or Equal?(x=w1933, y=1) -> (x >= y?=w1930:bool)
                n1657 = case shown="真" w1930 {
                  tunnel: [T6."读取数据" ("元素") w1935] -> w1931
                  frame False {
                  }
                  frame True {
                    n1658 = local read "重发数据"() -> (w1936:bool)
                    n1659 = Obtain Queue(name (unnamed)="重发掉线数据" ("名称（未命名）"), element data type=T16."水样测试") -> (queue out=w1942:refnum<queue>, error out=w1939:errorcluster)  [unwired: 3 in, 1 out]
                    n1660 = case shown="假" w1936 {
                      tunnel: w1942 -> [w1948 w1955]
                      tunnel: [w1946 w1955] -> w1940
                      tunnel: w1939 -> [w1945 w1954]
                      tunnel: [w1944 w1954] -> w1938
                      frame False {
                        n1661 = for {
                          N: 8 -> [_]
                          tunnel: w1948 -> [w1953]
                          tunnel: [w1951] -> w1946
                          tunnel: w1945 -> [w1950]
                          tunnel: [w1949] -> w1944
                          i -> [w1952]
                          n1662 = Enqueue Element(queue=w1953, element=w1952, error in (no error)=w1950) -> (queue out=w1951:refnum<queue>, error out=w1949:errorcluster)  [unwired: 1 in, 1 out]
                        }
                      }
                      frame True {
                      }
                    }
                    n1663 = Dequeue Element(queue=w1940, error in (no error)=w1938) -> (element=w1937:T16)  [unwired: 1 in, 3 out]
                    n1664 = case shown="\"加标回收\"" w1937 {
                      tunnel: [w1956 w1971 w1985 w1995 w2005 w2018 w2031 w2044] -> w1935
                      frame "水样测试", Default {
                        n1665 = flat-sequence {
                          tunnel: [w1964] -> w1956
                          frame #0 {
                            n1666 = global write "全局 小时数据发送次数.vi" "小时数据发送次数"(0 ("数值")) -> ()
                            n1667 = global write "全局 实时数据参数.vi" "实时数据参数"("水样测试") -> ()
                            n1668 = local write "table元素"("提取实时数据" ("新元素/子数组")) -> ()
                            n1669 = global write "全局1.vi" "枚举"(enum16{"返回请求应答", "上传数据", "返回执行结果"}."上传数据" ("枚举")) -> ()
                          }
                          frame #1 {
                            n1670 = call "从数据库获取数据通用可配置(子VI).vi"("table输入"="实时数据" ("新元素/子数组"), "列队名（唯一）"="adiao") -> ()  [unwired: 8 in, 2 out]
                          }
                          frame #2 {
                            # "数据处理整合"
                            n1671 = call "数据处理整合 (子VI).vi"("枚举"=enum16{"实时数据排序", "小时数据排序"}."实时数据排序") -> ("已排序的数组"=w1968:string[])  [unwired: 10 in]
                            n1672 = Array Size(array=w1968) -> (size(s)=w1967:i32)
                            n1673 = global write "全局 数据数组大小.vi" "数据数组大小"(w1967) -> ()
                            n1674 = Greater Than 0?(x=w1967) -> (x > 0?=w1966:bool)
                            n1675 = case shown="真" w1966 {
                              tunnel: [T6."表格比对" ("元素") T6."发送数据" ("元素")] -> w1964
                              frame False {
                              }
                              frame True {
                              }
                            }
                            "重发数据" <- TRUE ("重发数据中")
                          }
                        }
                      }
                      frame "小时数据" {
                        n1676 = flat-sequence {
                          tunnel: [w1979] -> w1971
                          frame #0 {
                            n1677 = local read "TCP掉线时间节点"() -> (w1973:string)
                            n1678 = call "当前时间格式显示 (子VI).vi"() -> ("当前时间格式显示"=w1972:string)  [unwired: 11 in]
                            n1679 = global write "全局 时间2.vi" "小时数据时间2"(w1972) -> ()
                            n1680 = global write "全局 水样时间.vi" "小时数据时间"(w1973) -> ()
                            n1681 = global write "全局 小时数据发送次数.vi" "小时数据发送次数"(0 ("数值")) -> ()
                            n1682 = local write "table元素"("小时数据" ("新元素/子数组")) -> ()
                            n1683 = global write "全局1.vi" "枚举"(enum16{"返回请求应答", "上传数据", "返回执行结果"}."返回请求应答" ("枚举")) -> ()
                          }
                          frame #1 {
                            n1684 = call "从数据库获取数据通用可配置(子VI).vi"("table输入"="小时数据" ("新元素/子数组"), "列队名（唯一）"="XS" ("名称（未命名）")) -> ()  [unwired: 8 in, 2 out]
                          }
                          frame #2 {
                            # "数据处理整合"
                            n1685 = call "数据处理整合 (子VI).vi"() -> ("已排序的数组"=w1982:string[])  [unwired: 11 in]
                            n1686 = Array Size(array=w1982) -> (size(s)=w1981:i32)
                            n1687 = global write "全局 数据数组大小.vi" "数据数组大小"(w1981) -> ()
                            n1688 = Greater Than 0?(x=w1981) -> (x > 0?=w1980:bool)
                            n1689 = case shown="真" w1980 {
                              tunnel: [T6."表格比对" ("元素") T6."发送数据" ("元素")] -> w1979
                              frame False {
                              }
                              frame True {
                              }
                            }
                          }
                        }
                      }
                      frame "日志信息" {
                        n1690 = flat-sequence {
                          tunnel: [w1989] -> w1985
                          frame #0 {
                            n1691 = global write "全局 小时数据发送次数.vi" "小时数据发送次数"(0 ("数值")) -> ()
                            n1692 = global write "全局1.vi" "枚举"(enum16{"返回请求应答", "上传数据", "返回执行结果"}."上传数据" ("枚举")) -> ()
                            n1693 = local write "table元素"("操作日志" ("新元素/子数组")) -> ()
                          }
                          frame #1 {
                            n1694 = call "获取操作日志 (子VI).vi"() -> ()  [unwired: 12 in]
                          }
                          frame #2 {
                            # "数据处理整合"
                            n1695 = call "数据处理整合 (子VI).vi"() -> ("已排序的数组"=w1992:string[])  [unwired: 11 in]
                            n1696 = Array Size(array=w1992) -> (size(s)=w1991:i32)
                            n1697 = global write "全局 数据数组大小.vi" "数据数组大小"(w1991) -> ()
                            n1698 = Greater Than 0?(x=w1991) -> (x > 0?=w1990:bool)
                            n1699 = case shown="假" w1990 {
                              tunnel: [T6."表格比对" ("元素") T6."发送数据" ("元素")] -> w1989
                              frame False {
                              }
                              frame True {
                              }
                            }
                          }
                        }
                      }
                      frame "报警信息" {
                        n1700 = flat-sequence {
                          tunnel: [w1999] -> w1995
                          frame #0 {
                            n1701 = global write "全局 小时数据发送次数.vi" "小时数据发送次数"(0 ("数值")) -> ()
                            n1702 = global write "全局1.vi" "枚举"(enum16{"返回请求应答", "上传数据", "返回执行结果"}."上传数据" ("枚举")) -> ()
                            n1703 = local write "table元素"("报警信息" ("新元素/子数组")) -> ()
                          }
                          frame #1 {
                            n1704 = call "获取报警信息 (子VI).vi"() -> ()  [unwired: 12 in]
                          }
                          frame #2 {
                            # "数据处理整合"
                            n1705 = call "数据处理整合 (子VI).vi"() -> ("已排序的数组"=w2002:string[])  [unwired: 11 in]
                            n1706 = Array Size(array=w2002) -> (size(s)=w2001:i32)
                            n1707 = Greater Than 0?(x=w2001) -> (x > 0?=w2000:bool)
                            n1708 = global write "全局 数据数组大小.vi" "数据数组大小"(w2001) -> ()
                            n1709 = case shown="假" w2000 {
                              tunnel: [T6."表格比对" ("元素") T6."发送数据" ("元素")] -> w1999
                              frame False {
                              }
                              frame True {
                              }
                            }
                          }
                        }
                      }
                      frame "零点核查" {
                        n1710 = flat-sequence {
                          tunnel: [w2012] -> w2005
                          frame #0 {
                            n1711 = global write "全局 小时数据发送次数.vi" "小时数据发送次数"(0 ("数值")) -> ()
                            n1712 = global write "全局 实时数据参数.vi" "实时数据参数"("空白测试") -> ()
                            n1713 = local write "table元素"("实时数据" ("新元素/子数组")) -> ()
                            n1714 = global write "全局1.vi" "枚举"(enum16{"返回请求应答", "上传数据", "返回执行结果"}."返回请求应答" ("枚举")) -> ()
                          }
                          frame #1 {
                            n1715 = call "从数据库获取数据通用可配置(子VI).vi"("table输入"="实时数据" ("新元素/子数组"), "列队名（唯一）"="bdiao") -> ()  [unwired: 8 in, 2 out]
                          }
                          frame #2 {
                            # "数据处理整合"
                            n1716 = call "数据处理整合 (子VI).vi"() -> ("已排序的数组"=w2015:string[])  [unwired: 11 in]
                            n1717 = Array Size(array=w2015) -> (size(s)=w2014:i32)
                            n1718 = global write "全局 数据数组大小.vi" "数据数组大小"(w2014) -> ()
                            n1719 = Greater Than 0?(x=w2014) -> (x > 0?=w2013:bool)
                            n1720 = case shown="假" w2013 {
                              tunnel: [T6."表格比对" ("元素") T6."发送数据" ("元素")] -> w2012
                              frame False {
                              }
                              frame True {
                              }
                            }
                          }
                        }
                      }
                      frame "标样核查" {
                        n1721 = flat-sequence {
                          tunnel: [w2025] -> w2018
                          frame #0 {
                            n1722 = global write "全局 小时数据发送次数.vi" "小时数据发送次数"(0 ("数值")) -> ()
                            n1723 = global write "全局 实时数据参数.vi" "实时数据参数"("跨度核查") -> ()
                            n1724 = global write "全局1.vi" "枚举"(enum16{"返回请求应答", "上传数据", "返回执行结果"}."返回请求应答" ("枚举")) -> ()
                            n1725 = local write "table元素"("实时数据" ("新元素/子数组")) -> ()
                          }
                          frame #1 {
                            n1726 = call "从数据库获取数据通用可配置(子VI).vi"("table输入"="实时数据" ("新元素/子数组"), "列队名（唯一）"="cdiao") -> ()  [unwired: 8 in, 2 out]
                          }
                          frame #2 {
                            # "数据处理整合"
                            n1727 = call "数据处理整合 (子VI).vi"() -> ("已排序的数组"=w2028:string[])  [unwired: 11 in]
                            n1728 = Array Size(array=w2028) -> (size(s)=w2027:i32)
                            n1729 = global write "全局 数据数组大小.vi" "数据数组大小"(w2027) -> ()
                            n1730 = Greater Than 0?(x=w2027) -> (x > 0?=w2026:bool)
                            n1731 = case shown="假" w2026 {
                              tunnel: [T6."表格比对" ("元素") T6."发送数据" ("元素")] -> w2025
                              frame False {
                              }
                              frame True {
                              }
                            }
                          }
                        }
                      }
                      frame "平行样" {
                        n1732 = flat-sequence {
                          tunnel: [w2038] -> w2031
                          frame #0 {
                            n1733 = global write "全局 小时数据发送次数.vi" "小时数据发送次数"(0 ("数值")) -> ()
                            n1734 = global write "全局 实时数据参数.vi" "实时数据参数"("平行样测试") -> ()
                            n1735 = local write "table元素"("提取实时数据" ("新元素/子数组")) -> ()
                            n1736 = global write "全局1.vi" "枚举"(enum16{"返回请求应答", "上传数据", "返回执行结果"}."上传数据" ("枚举")) -> ()
                          }
                          frame #1 {
                            n1737 = call "从数据库获取数据通用可配置(子VI).vi"("table输入"="实时数据" ("新元素/子数组"), "列队名（唯一）"="ddiao") -> ()  [unwired: 8 in, 2 out]
                          }
                          frame #2 {
                            # "数据处理整合"
                            n1738 = call "数据处理整合 (子VI).vi"() -> ("已排序的数组"=w2041:string[])  [unwired: 11 in]
                            n1739 = Array Size(array=w2041) -> (size(s)=w2040:i32)
                            n1740 = global write "全局 数据数组大小.vi" "数据数组大小"(w2040) -> ()
                            n1741 = Greater Than 0?(x=w2040) -> (x > 0?=w2039:bool)
                            n1742 = case shown="假" w2039 {
                              tunnel: [T6."表格比对" ("元素") T6."发送数据" ("元素")] -> w2038
                              frame False {
                              }
                              frame True {
                              }
                            }
                          }
                        }
                      }
                      frame "加标回收" {
                        n1743 = flat-sequence {
                          tunnel: [w2052] -> w2044
                          frame #0 {
                            n1744 = global write "全局 小时数据发送次数.vi" "小时数据发送次数"(0 ("数值")) -> ()
                            n1745 = global write "全局 实时数据参数.vi" "实时数据参数"("加标回收测试") -> ()
                            n1746 = global write "全局1.vi" "枚举"(enum16{"返回请求应答", "上传数据", "返回执行结果"}."上传数据" ("枚举")) -> ()
                            n1747 = local write "table元素"("实时数据" ("新元素/子数组")) -> ()
                          }
                          frame #1 {
                            n1748 = call "从数据库获取数据通用可配置(子VI).vi"("table输入"="加标回收" ("新元素/子数组"), "列队名（唯一）"="ediao") -> ()  [unwired: 8 in, 2 out]
                          }
                          frame #2 {
                            # "数据处理整合"
                            n1749 = call "加标回收数据处理整合 (子VI).vi"() -> ("已排序的数组"=w2051:string[])  [unwired: 11 in]
                            n1750 = Array Size(array=w2051) -> (size(s)=w2054:i32)
                            n1751 = global write "全局 数据数组大小.vi" "数据数组大小"(w2054) -> ()
                            n1752 = Greater Than 0?(x=w2054) -> (x > 0?=w2053:bool)
                            n1753 = case shown="假" w2053 {
                              tunnel: [T6."读取数据" ("元素") T6."发送数据" ("元素")] -> w2052
                              frame False {
                              }
                              frame True {
                              }
                            }
                          }
                        }
                      }
                    }
                  }
                }
              }
              frame Enabled {
              }
            }
            n1754 = disable-structure shown="启用" {
              disable-tunnel: [w2063 _] -> w1923
              frame Disabled {
                n1755 = call "数据表比对.vi"("查询元素输入"="氨氮" ("table输入 2"), "table输入"="实时数据") -> ("待发送第一条数据"=w2063:string[], "待发送数据"=w2057:string[][])  [unwired: 6 in, 2 out]
                n1756 = Empty Array?(array=w2057) -> (empty?=w2062:bool)
                n1757 = local read "心跳包"() -> (w2060:bool)
                n1758 = Not(x=w2062) -> (.not. x?=w2061:bool)
                n1759 = Or(x=w2061, y=w2060) -> ()  [unwired: 1 out]
              }
              frame Enabled {
              }
            }
            n1760 = case shown="假" FALSE {
              tunnel: w1928 -> [w2065 w2066]
              tunnel: [w2064 w2066] -> w1927
              frame False {
                n1761 = Increment(x=w2065) -> (x+1=w2064:i32)
              }
              frame True {
              }
            }
            n1762 = Enqueue Element(queue=w1924, element=T6."读取数据" ("元素"), timeout in ms (-1)=1000 ("超时毫秒(-1)")) -> ()  [unwired: 1 in, 3 out]
          }
          frame "读取数据" {
            w2078 = FALSE ("数据正在发送")
            # "设置测量时间间隔"
            # "1000设置超时时间和重发次数\n1011提取监测仪表时间\n1012设置监测仪表时间\n1014提取数采仪时间\n1015设置数采仪时间\n1061提取实时数据间隔\n1062设置实时数据间隔\n1072设置数采仪访问密码"
            # "6分钟掉线重连"
            n1763 = property on="TCP服务端掉线计数" class="DigNum (严格)"("Value"=0 ("TCP服务端掉线计数")) -> ()  [unwired: 2 in, 2 out]
            n1764 = global write "全局 数据发送重叠.vi" "掉线指示灯"(FALSE ("数据发送重叠")) -> ()
            n1765 = local write "重发数据"(w2078) -> ()
            n1766 = local write "查询数据发送"(w2078) -> ()
            n1767 = property on="实时数据发送时间间隔/min" class="DigNum (严格)"() -> ("Value"=w2090:u32)  [unwired: 2 in, 2 out]
            n1768 = global write "实时数据发送间隔全局.vi" "实时数据发送间隔"(w2090) -> ()
            n1769 = property on="设置超时时间/min" class="DigNum (严格)"() -> ("Value"=w2092:i32)  [unwired: 2 in, 2 out]
            n1770 = Multiply(x=w2092, y=10000) -> ()  [unwired: 1 out]
            n1771 = local read "数据发送通道"() -> (w2074:enum16{"TCP", "VISA"})
            n1772 = call "VISATCP组合选择发送.vi"("数据发送通道"=w2074, "命令"="read", "error in (no error)"=w2072) -> ("读取缓冲区"=w2071:string, "错误输出"=w2070:errorcluster)  [unwired: 9 in, 2 out]
            n1773 = Empty String/Path?(string/path=w2071) -> (empty?=w2075:bool)
            n1774 = case shown="假" w2075 {
              tunnel: w2071 -> [w2105 _]
              frame False {
                n1775 = call "数据记录.vi"("写入字段"=w2105) -> ("连接的字符串"=→"读取报文显示":string)  [unwired: 10 in]
                n1776 = global write "全局1.vi" "数据输出"(w2105) -> ()
                "数据输出" <- w2105
              }
              frame True {
              }
            }
            n1777 = control-ref of="数组 2"() -> (w2094:refnum<vi>)
            n1778 = control-ref of="数组"() -> (w2093:refnum<vi>)
            n1779 = call "读取数据处理 (子VI).vi"("Array输入"=w2094, "data out"=w2071, "reference"=w2093) -> ("数组"=→"数组":string[], "系统编码ST"=→"系统编码ST":string, "数组 2"=→"数组 2":string[], "命令编码CN"=w2083:string, "设备编码MN"=→"设备编码MN":string, "密码PW"=→"密码PW":string, "数据"=→"数据":string, "拆分包及应答Flag"=→"拆分包及应答Flag":string, "时间QN"=w2086:string)  [unwired: 4 in]
            "命令编码CN" <- w2083
            "时间QN" <- w2086
            n1780 = Search/Split String(string=w2086, search string/char (-)="QN=" ("搜索字符串/字符(-)")) -> (match + rest of string=w2084:string)  [unwired: 1 in, 2 out]
            n1781 = String Subset(string=w2084, offset (0)=3 ("偏移量(0)")) -> (substring=→"QN":string)  [unwired: 1 in]
            n1782 = Search/Split String(string=w2083, search string/char (-)="CN=" ("搜索字符串/字符(-)")) -> (match + rest of string=w2067:string)  [unwired: 1 in, 2 out]
            n1783 = String Subset(string=w2067, offset (0)=3 ("偏移量(0)")) -> (substring=w2076:string)  [unwired: 1 in]
            n1784 = case shown="\"3080\", \"3081\", \"3082\", \"3083\", \"3084\", \"3085\", \"3086\"" w2076 {
              tunnel: w2082 -> [w2108 w2110 w2124 w2127 w2130 w2133 w2136 w2139 w2146 w2149 w2168 w2186 w2205 w2223 w2241 w2260 w2279 w2297 w2312 w2434 w2437 w2441 w2447 w2465 w2468 w2480 w2503 w2509]
              tunnel: [w2108 w2110 w2124 w2127 w2130 w2133 w2136 w2139 w2146 w2149 w2168 w2186 w2205 w2223 w2241 w2260 w2279 w2297 w2312 w2434 w2437 w2441 w2447 w2465 w2468 w2480 w2503 w2509] -> w2080
              tunnel: [T6."读取数据" ("元素") T6."发送数据" ("元素") T6."发送数据" ("元素") T6."发送数据" ("元素") T6."发送数据" ("元素") T6."发送数据" ("元素") T6."发送数据" ("元素") T6."发送数据" ("元素") T6."发送数据" ("元素") w2148 w2167 w2185 w2204 w2222 w2240 w2259 w2278 w2296 w2311 T6."发送数据" ("元素") w2436 w2440 T6."发送数据" ("元素") T6."发送数据" ("元素") T6."发送数据" ("元素") T6."发送数据" ("元素") T6."发送数据" ("元素") T6."发送数据" ("元素")] -> w2079
              tunnel: w2076 -> [_ _ _ _ _ _ _ _ _ _ _ _ _ _ _ _ _ _ _ _ _ _ _ _ _ _ _ w2507]
              frame "", Default {
              }
              frame "1000" {
                # "发回给平台"
                # "反控指令"
                # "3042~3086"
                # "1000"
                n1785 = property on="数据" class="Str"() -> ("Value"=w2116:string)  [unwired: 2 in, 2 out]
                n1786 = String Subset(string=w2116, offset (0)=9 ("偏移量(0)"), length (rest)=1 ("长度（剩余）")) -> (substring=w2113:string)
                n1787 = Decimal String To Number(string=w2113) -> (number=→"设置超时时间/min":i32)  [unwired: 2 in, 1 out]
                n1788 = local write "table元素"("反控命令" ("新元素/子数组")) -> ()
              }
              frame "1011" {
                # "1011"
                n1789 = local read "数据"() -> (w2122:string)
                n1790 = Search/Split String(string=w2122, search string/char (-)="PolId=" ("搜索字符串/字符(-)")) -> (match + rest of string=w2120:string)  [unwired: 1 in, 2 out]
                n1791 = String Subset(string=w2120, offset (0)=6 ("偏移量(0)"), length (rest)=6 ("长度（剩余）")) -> (substring=w2117:string)
                n1792 = global write "全局 提取仪器参数.vi" "仪器编码"(w2117) -> ()
                n1793 = local write "table元素"("提取监测仪表时间") -> ()
              }
              frame "1012" {
                # "设置监测仪表时间"
                n1794 = local write "table元素"("反控命令" ("新元素/子数组")) -> ()
              }
              frame "1014" {
                # "1014"
                n1795 = local write "table元素"("提取数采仪时间") -> ()
              }
              frame "1015" {
                # "设置数采仪时间"
                n1796 = local write "table元素"("反控命令" ("新元素/子数组")) -> ()
              }
              frame "1061" {
                # "1061"
                n1797 = local write "table元素"("提取实时数据间隔") -> ()
              }
              frame "1062" {
                # "发回给平台"
                # "反控指令"
                # "3042~3086"
                # "设置数据发送时间间隔"
                # "1062"
                n1798 = property on="数据" class="Str"() -> ("Value"=w2144:string)  [unwired: 2 in, 2 out]
                n1799 = String Subset(string=w2144, offset (0)=12 ("偏移量(0)")) -> (substring=w2142:string)  [unwired: 1 in]
                n1800 = Decimal String To Number(string=w2142) -> (number=w2141:i32)  [unwired: 2 in, 1 out]
                n1801 = property on="实时数据发送时间间隔/min" class="DigNum (严格)"("Value"=w2141) -> ()  [unwired: 2 in, 2 out]
                n1802 = local write "table元素"("反控命令" ("新元素/子数组")) -> ()
              }
              frame "1072" {
                # "设置数采仪密码"
                n1803 = local write "table元素"("反控命令" ("新元素/子数组")) -> ()
              }
              frame "2011" {
                w2154 = 0 ("数值")
                # "2011提取实时数据"
                n1804 = local read "数据"() -> (w2155:string)
                n1805 = String Subset(string=w2155, offset (0)=10 ("偏移量(0)"), length (rest)=14 ("长度（剩余）")) -> (substring=w2151:string)
                n1806 = String Subset(string=w2155, offset (0)=33 ("偏移量(0)"), length (rest)=14 ("长度（剩余）")) -> (substring=w2153:string)
                n1807 = call "格式时间字符串.vi"("字符串"=w2151) -> ("连接的字符串"=w2150:string)  [unwired: 10 in]
                n1808 = call "格式时间字符串.vi"("字符串"=w2153) -> ("连接的字符串"=w2152:string)  [unwired: 10 in]
                n1809 = global write "全局 小时数据发送次数.vi" "小时数据发送次数"(w2154) -> ()
                n1810 = global write "全局1.vi" "枚举"(w2154) -> ()
                n1811 = global write "起始时间.vi" "结束时间"(w2152) -> ()
                n1812 = global write "起始时间.vi" "起始时间"(w2150) -> ()
                n1813 = flat-sequence {
                  tunnel: [T6."发送数据" ("元素")] -> w2148
                  frame #0 {
                    w2160 = "提取实时数据" ("新元素/子数组")
                    n1814 = global write "全局 实时数据参数.vi" "实时数据参数"("水样测试") -> ()
                    n1815 = call "从数据库获取数据通用可配置(子VI).vi"("table输入"=w2160, "列队名（唯一）"=w2160) -> ()  [unwired: 8 in, 2 out]
                  }
                  frame #1 {
                    # "数据处理整合"
                    n1816 = local write "table元素"("提取实时数据" ("新元素/子数组")) -> ()
                    n1817 = call "数据处理整合 (子VI).vi"("枚举"=enum16{"实时数据排序", "小时数据排序"}."实时数据排序") -> ("已排序的数组"=w2163:string[])  [unwired: 10 in]
                    n1818 = Array Size(array=w2163) -> (size(s)=w2164:i32)
                    n1819 = global write "全局 数据数组大小.vi" "数据数组大小"(w2164) -> ()
                  }
                  frame #2 {
                  }
                }
              }
              frame "2061" {
                w2169 = 0 ("数值")
                n1820 = flat-sequence {
                  tunnel: [T6."发送数据" ("元素")] -> w2167
                  frame #0 {
                    # "格式时间"
                    # "2061、提取小时数据"
                    n1821 = local read "数据"() -> (w2176:string)
                    n1822 = String Subset(string=w2176, offset (0)=33 ("偏移量(0)"), length (rest)=14 ("长度（剩余）")) -> (substring=w2171:string)
                    n1823 = String Subset(string=w2176, offset (0)=10 ("偏移量(0)"), length (rest)=14 ("长度（剩余）")) -> (substring=w2172:string)
                    n1824 = call "格式时间字符串.vi"("字符串"=w2172) -> ("连接的字符串"=w2173:string)  [unwired: 10 in]
                    n1825 = call "格式时间字符串.vi"("字符串"=w2171) -> ("连接的字符串"=w2170:string)  [unwired: 10 in]
                    n1826 = global write "全局 水样时间.vi" "小时数据时间"(w2173) -> ()
                    n1827 = global write "全局 时间2.vi" "小时数据时间2"(w2170) -> ()
                  }
                  frame #1 {
                    w2179 = "小时数据" ("名称（未命名）")
                    # "提取COD、氨氮、多参数、总磷、总氮数据"
                    n1828 = call "从数据库获取数据通用可配置(子VI).vi"("table输入"=w2179, "列队名（唯一）"=w2179) -> ()  [unwired: 8 in, 2 out]
                  }
                  frame #2 {
                    # "数据处理整合"
                    n1829 = call "数据处理整合 (子VI).vi"("枚举"=enum16{"实时数据排序", "小时数据排序"}."小时数据排序") -> ("已排序的数组"=w2182:string[])  [unwired: 10 in]
                    n1830 = local write "table元素"("提取小时数据" ("新元素/子数组")) -> ()
                    n1831 = Array Size(array=w2182) -> (size(s)=w2181:i32)
                    n1832 = global write "全局 数据数组大小.vi" "数据数组大小"(w2181) -> ()
                  }
                  frame #3 {
                  }
                }
                n1833 = global write "全局 小时数据发送次数.vi" "小时数据发送次数"(w2169) -> ()
                n1834 = global write "全局1.vi" "枚举"(w2169) -> ()
              }
              frame "2062" {
                w2187 = 0 ("数值")
                n1835 = flat-sequence {
                  tunnel: [T6."发送数据" ("元素")] -> w2185
                  frame #0 {
                    # "格式时间"
                    # "2062、提取标样核查数据"
                    n1836 = local read "数据"() -> (w2194:string)
                    n1837 = String Subset(string=w2194, offset (0)=33 ("偏移量(0)"), length (rest)=14 ("长度（剩余）")) -> (substring=w2189:string)
                    n1838 = String Subset(string=w2194, offset (0)=10 ("偏移量(0)"), length (rest)=14 ("长度（剩余）")) -> (substring=w2190:string)
                    n1839 = call "格式时间字符串.vi"("字符串"=w2190) -> ("连接的字符串"=w2191:string)  [unwired: 10 in]
                    n1840 = call "格式时间字符串.vi"("字符串"=w2189) -> ("连接的字符串"=w2188:string)  [unwired: 10 in]
                    n1841 = global write "全局 水样时间.vi" "时间"(w2191) -> ()
                    n1842 = global write "全局 时间2.vi" "时间2"(w2188) -> ()
                  }
                  frame #1 {
                    # "提取COD、氨氮、多参数、总磷、总氮数据"
                    n1843 = call "从数据库获取数据通用可配置(子VI).vi"("table输入"="标样核查" ("新元素/子数组"), "列队名（唯一）"="核查数据" ("新元素/子数组")) -> ()  [unwired: 8 in, 2 out]
                  }
                  frame #2 {
                    # "数据处理整合"
                    n1844 = local write "table元素"("核查数据" ("新元素/子数组")) -> ()
                    n1845 = call "数据处理整合 (子VI).vi"("枚举"=enum16{"实时数据排序", "小时数据排序"}."实时数据排序") -> ("已排序的数组"=w2200:string[])  [unwired: 10 in]
                    n1846 = Array Size(array=w2200) -> (size(s)=w2201:i32)
                    n1847 = global write "全局 数据数组大小.vi" "数据数组大小"(w2201) -> ()
                  }
                  frame #3 {
                  }
                }
                n1848 = global write "全局 小时数据发送次数.vi" "小时数据发送次数"(w2187) -> ()
                n1849 = global write "全局1.vi" "枚举"(w2187) -> ()
              }
              frame "2063" {
                w2210 = 0 ("数值")
                # "2063提取加标回收数据"
                n1850 = local read "数据"() -> (w2211:string)
                n1851 = String Subset(string=w2211, offset (0)=10 ("偏移量(0)"), length (rest)=14 ("长度（剩余）")) -> (substring=w2207:string)
                n1852 = String Subset(string=w2211, offset (0)=33 ("偏移量(0)"), length (rest)=14 ("长度（剩余）")) -> (substring=w2209:string)
                n1853 = call "格式时间字符串.vi"("字符串"=w2207) -> ("连接的字符串"=w2206:string)  [unwired: 10 in]
                n1854 = call "格式时间字符串.vi"("字符串"=w2209) -> ("连接的字符串"=w2208:string)  [unwired: 10 in]
                n1855 = global write "全局 小时数据发送次数.vi" "小时数据发送次数"(w2210) -> ()
                n1856 = global write "全局1.vi" "枚举"(w2210) -> ()
                n1857 = global write "起始时间.vi" "结束时间"(w2208) -> ()
                n1858 = global write "起始时间.vi" "起始时间"(w2206) -> ()
                n1859 = flat-sequence {
                  tunnel: [T6."发送数据" ("元素")] -> w2204
                  frame #0 {
                    w2216 = "提取加标回收" ("新元素/子数组")
                    n1860 = call "从数据库获取数据通用可配置(子VI).vi"("table输入"=w2216, "列队名（唯一）"=w2216) -> ()  [unwired: 8 in, 2 out]
                  }
                  frame #1 {
                    n1861 = local write "table元素"("提取加标回收" ("新元素/子数组")) -> ()
                    n1862 = call "加标回收数据处理整合 (子VI).vi"("枚举"=enum16{"实时数据排序", "小时数据排序"}."实时数据排序") -> ("已排序的数组"=w2217:string[])  [unwired: 10 in]
                    n1863 = Array Size(array=w2217) -> (size(s)=w2219:i32)
                    n1864 = global write "全局 数据数组大小.vi" "数据数组大小"(w2219) -> ()
                  }
                  frame #2 {
                  }
                }
              }
              frame "2064" {
                w2228 = 0 ("数值")
                # "2064提取平行样数据"
                n1865 = local read "数据"() -> (w2229:string)
                n1866 = String Subset(string=w2229, offset (0)=10 ("偏移量(0)"), length (rest)=14 ("长度（剩余）")) -> (substring=w2225:string)
                n1867 = String Subset(string=w2229, offset (0)=33 ("偏移量(0)"), length (rest)=14 ("长度（剩余）")) -> (substring=w2227:string)
                n1868 = call "格式时间字符串.vi"("字符串"=w2225) -> ("连接的字符串"=w2224:string)  [unwired: 10 in]
                n1869 = call "格式时间字符串.vi"("字符串"=w2227) -> ("连接的字符串"=w2226:string)  [unwired: 10 in]
                n1870 = global write "全局 小时数据发送次数.vi" "小时数据发送次数"(w2228) -> ()
                n1871 = global write "全局1.vi" "枚举"(w2228) -> ()
                n1872 = global write "起始时间.vi" "结束时间"(w2226) -> ()
                n1873 = global write "起始时间.vi" "起始时间"(w2224) -> ()
                n1874 = flat-sequence {
                  tunnel: [T6."发送数据" ("元素")] -> w2222
                  frame #0 {
                    w2234 = "提取平行样" ("新元素/子数组")
                    n1875 = call "从数据库获取数据通用可配置(子VI).vi"("table输入"=w2234, "列队名（唯一）"=w2234) -> ()  [unwired: 8 in, 2 out]
                  }
                  frame #1 {
                    n1876 = call "数据处理整合 (子VI).vi"("枚举"=enum16{"实时数据排序", "小时数据排序"}."实时数据排序") -> ("已排序的数组"=w2237:string[])  [unwired: 10 in]
                    n1877 = Array Size(array=w2237) -> (size(s)=w2236:i32)
                    n1878 = local write "table元素"("提取平行样" ("新元素/子数组")) -> ()
                    n1879 = global write "全局 数据数组大小.vi" "数据数组大小"(w2236) -> ()
                  }
                  frame #2 {
                  }
                }
              }
              frame "2065" {
                w2242 = 0 ("数值")
                n1880 = flat-sequence {
                  tunnel: [T6."发送数据" ("元素")] -> w2240
                  frame #0 {
                    # "格式时间"
                    # "2065、提取零点核查数据"
                    n1881 = local read "数据"() -> (w2251:string)
                    n1882 = global write "全局 实时数据参数.vi" "实时数据参数"("空白测试" ("新元素/子数组")) -> ()
                    n1883 = local write "table元素"("空白测试" ("新元素/子数组")) -> ()
                    n1884 = String Subset(string=w2251, offset (0)=33 ("偏移量(0)"), length (rest)=14 ("长度（剩余）")) -> (substring=w2246:string)
                    n1885 = String Subset(string=w2251, offset (0)=10 ("偏移量(0)"), length (rest)=14 ("长度（剩余）")) -> (substring=w2247:string)
                    n1886 = call "格式时间字符串.vi"("字符串"=w2247) -> ("连接的字符串"=w2248:string)  [unwired: 10 in]
                    n1887 = call "格式时间字符串.vi"("字符串"=w2246) -> ("连接的字符串"=w2245:string)  [unwired: 10 in]
                    n1888 = global write "全局 水样时间.vi" "时间"(w2248) -> ()
                    n1889 = global write "全局 时间2.vi" "时间2"(w2245) -> ()
                  }
                  frame #1 {
                    w2254 = "空白测试" ("新元素/子数组")
                    n1890 = call "从数据库获取数据通用可配置(子VI).vi"("table输入"=w2254, "列队名（唯一）"=w2254) -> ()  [unwired: 8 in, 2 out]
                  }
                  frame #2 {
                    # "数据处理整合"
                    n1891 = call "数据处理整合 (子VI).vi"("枚举"=enum16{"实时数据排序", "小时数据排序"}."实时数据排序") -> ("已排序的数组"=w2256:string[])  [unwired: 10 in]
                    n1892 = Array Size(array=w2256) -> (size(s)=w2257:i32)
                    n1893 = global write "全局 数据数组大小.vi" "数据数组大小"(w2257) -> ()
                  }
                  frame #3 {
                  }
                }
                n1894 = global write "全局 小时数据发送次数.vi" "小时数据发送次数"(w2242) -> ()
                n1895 = global write "全局1.vi" "枚举"(w2242) -> ()
              }
              frame "2066" {
                w2261 = 0 ("数值")
                n1896 = flat-sequence {
                  tunnel: [T6."发送数据" ("元素")] -> w2259
                  frame #0 {
                    # "格式时间"
                    # "2066、提取跨度核查数据"
                    n1897 = local read "数据"() -> (w2270:string)
                    n1898 = String Subset(string=w2270, offset (0)=33 ("偏移量(0)"), length (rest)=14 ("长度（剩余）")) -> (substring=w2265:string)
                    n1899 = String Subset(string=w2270, offset (0)=10 ("偏移量(0)"), length (rest)=14 ("长度（剩余）")) -> (substring=w2266:string)
                    n1900 = global write "全局 实时数据参数.vi" "实时数据参数"("跨度核查" ("新元素/子数组")) -> ()
                    n1901 = local write "table元素"("跨度核查" ("新元素/子数组")) -> ()
                    n1902 = call "格式时间字符串.vi"("字符串"=w2266) -> ("连接的字符串"=w2267:string)  [unwired: 10 in]
                    n1903 = call "格式时间字符串.vi"("字符串"=w2265) -> ("连接的字符串"=w2264:string)  [unwired: 10 in]
                    n1904 = global write "全局 水样时间.vi" "时间"(w2267) -> ()
                    n1905 = global write "全局 时间2.vi" "时间2"(w2264) -> ()
                  }
                  frame #1 {
                    w2273 = "跨度核查" ("新元素/子数组")
                    (unwired) "跨度核查" ("名称（未命名）")
                    # "提取COD、氨氮、多参数、总磷、总氮数据"
                    n1906 = call "从数据库获取数据通用可配置(子VI).vi"("table输入"=w2273, "列队名（唯一）"=w2273) -> ()  [unwired: 8 in, 2 out]
                  }
                  frame #2 {
                    # "数据处理整合"
                    n1907 = call "数据处理整合 (子VI).vi"("枚举"=enum16{"实时数据排序", "小时数据排序"}."实时数据排序") -> ("已排序的数组"=w2276:string[])  [unwired: 10 in]
                    n1908 = Array Size(array=w2276) -> (size(s)=w2275:i32)
                    n1909 = global write "全局 数据数组大小.vi" "数据数组大小"(w2275) -> ()
                  }
                  frame #3 {
                  }
                }
                n1910 = global write "全局 小时数据发送次数.vi" "小时数据发送次数"(w2261) -> ()
                n1911 = global write "全局1.vi" "枚举"(w2261) -> ()
              }
              frame "2082" {
                w2284 = 0 ("数值")
                # "2082提取集成干预"
                n1912 = local read "数据"() -> (w2285:string)
                n1913 = String Subset(string=w2285, offset (0)=10 ("偏移量(0)"), length (rest)=14 ("长度（剩余）")) -> (substring=w2281:string)
                n1914 = String Subset(string=w2285, offset (0)=33 ("偏移量(0)"), length (rest)=14 ("长度（剩余）")) -> (substring=w2283:string)
                n1915 = call "格式时间字符串.vi"("字符串"=w2281) -> ("连接的字符串"=w2280:string)  [unwired: 10 in]
                n1916 = call "格式时间字符串.vi"("字符串"=w2283) -> ("连接的字符串"=w2282:string)  [unwired: 10 in]
                n1917 = global write "全局 小时数据发送次数.vi" "小时数据发送次数"(w2284) -> ()
                n1918 = global write "全局1.vi" "枚举"(w2284) -> ()
                n1919 = global write "起始时间.vi" "结束时间"(w2282) -> ()
                n1920 = global write "起始时间.vi" "起始时间"(w2280) -> ()
                n1921 = flat-sequence {
                  tunnel: [T6."发送数据" ("元素")] -> w2278
                  frame #0 {
                    w2290 = "提取集成干预" ("新元素/子数组")
                    n1922 = call "从数据库获取数据通用可配置(子VI).vi"("table输入"=w2290, "列队名（唯一）"=w2290) -> ()  [unwired: 8 in, 2 out]
                  }
                  frame #1 {
                    n1923 = call "数据处理整合 (子VI).vi"("枚举"=enum16{"实时数据排序", "小时数据排序"}."实时数据排序") -> ("已排序的数组"=w2293:string[])  [unwired: 10 in]
                    n1924 = Array Size(array=w2293) -> (size(s)=w2292:i32)
                    n1925 = local write "table元素"("提取集成干预" ("新元素/子数组")) -> ()
                    n1926 = global write "全局 数据数组大小.vi" "数据数组大小"(w2292) -> ()
                  }
                  frame #2 {
                  }
                }
              }
              frame "3015" {
                n1927 = flat-sequence {
                  tunnel: [T6."发送数据" ("元素")] -> w2296
                  frame #0 {
                    # "发命令给中控"
                    # "发回给平台"
                    # "3015、手动远程留样"
                    n1928 = local write "table元素"("超标留样返回" ("新元素/子数组")) -> ()
                    n1929 = Insert Into Array(array=u16[] [] ("holding register values"), index=0 ("索引"), new element=u16 1 ("新元素/子数组")) -> (w2300:u16[])
                    n1930 = call "Modbus Master.vi"("Unit ID"=u8 1, "读取写入选择"="写入", "holding register values"=w2300, "starting address"=u16 10) -> ()  [unwired: 6 in, 2 out]
                  }
                  frame #1 {
                  }
                }
              }
              frame "3020" {
                n1931 = flat-sequence {
                  tunnel: [w2316] -> w2310
                  tunnel: [w2317] -> w2309
                  tunnel: [w2315] -> w2308
                  tunnel: [w2313] -> w2307
                  tunnel: w2310 -> [w2366]
                  tunnel: w2309 -> [w2365]
                  tunnel: w2308 -> [w2364]
                  tunnel: w2307 -> [w2363]
                  tunnel: [T6."发送数据" ("元素")] -> w2311
                  frame #0 {
                    w2336 = 0 ("数值")
                    # "3020、提取日志、报警，仪器参数"
                    n1932 = local read "数据"() -> (w2337:string)
                    n1933 = Search/Split String(string=w2337, search string/char (-)="BeginTime=" ("搜索字符串")) -> (match + rest of string=w2335:string)  [unwired: 1 in, 2 out]
                    n1934 = local read "数据"() -> (w2321:string)
                    n1935 = case shown="\"\"" w2335 {
                      tunnel: ["1904/01/01 00:00:00" w2360] -> w2339
                      tunnel: w2335 -> [_ w2354]
                      tunnel: [w2347 w2355] -> w2334
                      frame "" {
                        # "时间"
                        n1936 = Get Date/Time In Seconds() -> (seconds since 1Jan1904=w2348:timestamp)
                        n1937 = Format Date/Time String(time format string (%c)="%Y%m%d%H%M%S%3u" ("时间格式字符串(%c)"), seconds (now)=w2348) -> (date/time string=w2352:string)  [unwired: 1 in]
                        n1938 = Search and Replace String(input string=w2352, search string="." ("搜索字符串")) -> (result string=w2351:string)  [unwired: 6 in, 3 out]
                        n1939 = call "格式时间字符串.vi"("字符串"=w2351) -> ("连接的字符串"=w2347:string)  [unwired: 10 in]
                      }
                      frame "真", Default {
                        # "格式时间"
                        n1940 = String Subset(string=w2354, offset (0)=33 ("偏移量(0)"), length (rest)=14 ("长度（剩余）")) -> (substring=w2358:string)
                        n1941 = String Subset(string=w2354, offset (0)=10 ("偏移量(0)"), length (rest)=14 ("长度（剩余）")) -> (substring=w2359:string)
                        n1942 = call "格式时间字符串.vi"("字符串"=w2358) -> ("连接的字符串"=w2355:string)  [unwired: 10 in]
                        n1943 = call "格式时间字符串.vi"("字符串"=w2359) -> ("连接的字符串"=w2360:string)  [unwired: 10 in]
                      }
                    }
                    n1944 = call "日志报警参数选择 (子VI).vi"("String输入"=w2321) -> ("输出簇"=w2320:T18)  [unwired: 9 in, 1 out]
                    n1945 = Unbundle By Name(w2320) -> ("高锰酸盐"=w2328:string, "化学需氧量"=w2329:string, "氨氮"=w2330:string, "总磷"=w2331:string, "总氮"=w2332:string, "数采仪"=w2333:string, "高锰酸盐"=w2322:bool, "化学需氧量"=w2323:bool, "氨氮"=w2324:bool, "总磷"=w2325:bool, "总氮"=w2326:bool, "数采仪"=w2327:bool)
                    n1946 = Build Array(w2328, w2329, w2330, w2331, w2332, w2333) -> (w2315:string[])
                    n1947 = global write "全局 时间2.vi" "时间2"(w2334) -> ()
                    n1948 = Build Array(w2322, w2323, w2324, w2325, w2326, w2327) -> (w2314:bool[])
                    n1949 = global write "全局 水样时间.vi" "时间"(w2339) -> ()
                    n1950 = Or Array Elements(Boolean array=w2314) -> (logical OR=w2313:bool)
                    n1951 = global write "全局 小时数据发送次数.vi" "小时数据发送次数"(w2336) -> ()
                    n1952 = Obtain Queue(name (unnamed)="操作日志报警信息" ("名称（未命名）"), element data type=T17."CODMn") -> (queue out=w2316:refnum<queue>, error out=w2317:errorcluster)  [unwired: 3 in, 1 out]
                    n1953 = case shown="假" w2313 {
                      tunnel: w2316 -> [_ w2341]
                      tunnel: w2314 -> [_ w2340]
                      frame False {
                      }
                      frame True {
                        n1954 = for {
                          tunnel: w2340 -> [w2343] mode=indexing
                          tunnel: w2341 -> [w2342]
                          i -> [w2344]
                          n1955 = case shown="真" w2343 {
                            tunnel: w2344 -> [_ w2346]
                            tunnel: w2342 -> [_ w2345]
                            frame False {
                            }
                            frame True {
                              n1956 = call "提取日志报警参数入列队 (子VI).vi"("枚举"=w2346, "queue in"=w2345) -> ()  [unwired: 10 in]
                            }
                          }
                        }
                      }
                    }
                    n1957 = global write "全局1.vi" "枚举"(w2336) -> ()
                  }
                  frame #1 {
                    # "按需求提取COD、氨氮、总磷、总氮日志"
                    # "按需求提取COD、氨氮、总磷、总氮日志"
                    n1958 = case shown="真" w2363 {
                      tunnel: w2365 -> [_ w2369]
                      tunnel: w2366 -> [_ w2368]
                      tunnel: w2364 -> [_ w2367]
                      frame False {
                      }
                      frame True {
                        n1959 = while {
                          shift-right: [w2383] -> _
                          shift-left: w2368 -> [w2384]
                          tunnel: w2369 -> [w2382]
                          tunnel: w2367 -> [w2377]
                          stop <- w2379 stop-if-true
                          n1960 = Dequeue Element(queue=w2384, error in (no error)=w2382) -> (queue out=w2381:refnum<queue>, element=w2376:T17)  [unwired: 1 in, 2 out]
                          n1961 = Index Array(array=w2377) -> (element #1=w2375:string, element #2=w2374:string, element #3=w2373:string, element #4=w2372:string, element #5=w2371:string, element #6=w2370:string)  [unwired: 6 in]
                          n1962 = case shown="\"CODCr\"" w2376 {
                            tunnel: w2381 -> [w2389 _ w2398 w2403 w2407 w2412]
                            tunnel: [w2389 _ w2398 w2403 w2407 w2412] -> w2383
                            tunnel: w2375 -> [w2386 _ _ _ _ _]
                            tunnel: w2374 -> [_ w2391 _ _ _ _]
                            tunnel: w2373 -> [_ _ w2395 _ _ _]
                            tunnel: w2372 -> [_ _ _ w2400 _ _]
                            tunnel: w2371 -> [_ _ _ _ w2405 _]
                            tunnel: w2370 -> [_ _ _ _ _ w2409]
                            frame "CODMn" {
                              w2385 = string[][] [] ("氨氮")
                              n1963 = call "数据表比对.vi"("仪器日志参数"="CODMn" ("元素"), "table输入"=w2386) -> ("待发送数据"=w2387:string[][])  [unwired: 6 in, 3 out]
                              n1964 = global write "全局 所有参数.vi" "CODMn"(w2387) -> ()
                              n1965 = global write "全局 所有参数.vi" "总氮"(w2385) -> ()
                              n1966 = global write "全局 所有参数.vi" "CODCr"(w2385) -> ()
                              n1967 = global write "全局 所有参数.vi" "总磷"(w2385) -> ()
                              n1968 = global write "全局 所有参数.vi" "氨氮"(w2385) -> ()
                            }
                            frame "CODCr" {
                              w2390 = string[][] [] ("氨氮")
                              n1969 = call "数据表比对.vi"("仪器日志参数"="CODCr" ("元素"), "table输入"=w2391) -> ("待发送数据"=w2392:string[][])  [unwired: 6 in, 3 out]
                              n1970 = global write "全局 所有参数.vi" "CODCr"(w2392) -> ()
                              n1971 = global write "全局 所有参数.vi" "CODMn"(w2390) -> ()
                              n1972 = global write "全局 所有参数.vi" "总氮"(w2390) -> ()
                              n1973 = global write "全局 所有参数.vi" "总磷"(w2390) -> ()
                              n1974 = global write "全局 所有参数.vi" "氨氮"(w2390) -> ()
                            }
                            frame "氨氮" {
                              w2394 = string[][] [] ("氨氮")
                              n1975 = call "数据表比对.vi"("仪器日志参数"="氨氮" ("元素"), "table输入"=w2395) -> ("待发送数据"=w2396:string[][])  [unwired: 6 in, 3 out]
                              n1976 = global write "全局 所有参数.vi" "氨氮"(w2396) -> ()
                              n1977 = global write "全局 所有参数.vi" "CODMn"(w2394) -> ()
                              n1978 = global write "全局 所有参数.vi" "总氮"(w2394) -> ()
                              n1979 = global write "全局 所有参数.vi" "CODCr"(w2394) -> ()
                              n1980 = global write "全局 所有参数.vi" "总磷"(w2394) -> ()
                            }
                            frame "总磷" {
                              w2399 = string[][] [] ("氨氮")
                              n1981 = call "数据表比对.vi"("仪器日志参数"="总磷" ("元素"), "table输入"=w2400) -> ("待发送数据"=w2401:string[][])  [unwired: 6 in, 3 out]
                              n1982 = global write "全局 所有参数.vi" "总磷"(w2401) -> ()
                              n1983 = global write "全局 所有参数.vi" "CODMn"(w2399) -> ()
                              n1984 = global write "全局 所有参数.vi" "总氮"(w2399) -> ()
                              n1985 = global write "全局 所有参数.vi" "CODCr"(w2399) -> ()
                              n1986 = global write "全局 所有参数.vi" "氨氮"(w2399) -> ()
                            }
                            frame "总氮" {
                              w2404 = string[][] [] ("氨氮")
                              n1987 = call "数据表比对.vi"("仪器日志参数"="总氮" ("元素"), "table输入"=w2405) -> ("待发送数据"=w2406:string[][])  [unwired: 6 in, 3 out]
                              n1988 = global write "全局 所有参数.vi" "总氮"(w2406) -> ()
                              n1989 = global write "全局 所有参数.vi" "CODMn"(w2404) -> ()
                              n1990 = global write "全局 所有参数.vi" "氨氮"(w2404) -> ()
                              n1991 = global write "全局 所有参数.vi" "CODCr"(w2404) -> ()
                              n1992 = global write "全局 所有参数.vi" "总磷"(w2404) -> ()
                            }
                            frame "数采仪" {
                              n1993 = call "数据表比对.vi"("仪器日志参数"="系统" ("元素"), "table输入"=w2409) -> ("待发送数据"=w2410:string[][])  [unwired: 6 in, 3 out]
                              n1994 = global write "全局 所有参数.vi" "DO"(w2410) -> ()
                            }
                          }
                          n1995 = Get Queue Status(queue=w2381) -> (# elements in queue=w2380:i32)  [unwired: 2 in, 7 out]
                          n1996 = Wait (ms)(milliseconds to wait=u32 300 ("等待时间（毫秒）")) -> ()  [unwired: 1 out]
                          n1997 = Equal To 0?(x=w2380) -> (x = 0?=w2379:bool)
                        }
                      }
                    }
                  }
                  frame #2 {
                    n1998 = local read "数据"() -> (w2421:string)
                    n1999 = Search/Split String(string=w2421, search string/char (-)="InfoId=" ("搜索字符串/字符(-)")) -> (match + rest of string=w2419:string)  [unwired: 1 in, 2 out]
                    n2000 = String Subset(string=w2419, offset (0)=7 ("偏移量(0)"), length (rest)=6 ("长度（剩余）")) -> (substring=w2415:string)
                    n2001 = case shown="\"i13001\", \"i13002\", \"i13003\", \"i13004\", \"i13005\", \"i13006\", \"i13007\", \"i13008\", \"i13009\", \"i13010\", \"i13011\", \"i13012\", \"i13013\"" w2415 {
                      selector: w2415 -> [_ w2426 _]
                      tunnel: ["操作日志" ("名称（未命名）") "提取仪器参数" ("名称（未命名）") "报警信息" ("名称（未命名）")] -> w2414
                      tunnel: [w2422 1 ("数据数组大小") w2429] -> w2413
                      frame "i11001", "i21001" {
                        # "数据处理整合"
                        # "i11001日志"
                        n2002 = call "数据处理整合 (子VI).vi"("枚举"=enum16{"实时数据排序", "小时数据排序"}."实时数据排序") -> ("已排序的数组"=w2423:string[])  [unwired: 10 in]
                        n2003 = Array Size(array=w2423) -> (size(s)=w2422:i32)
                      }
                      frame "i13001", "i13002", "i13003", "i13004", "i13005", "i13006", "i13007", "i13008", "i13009", "i13010", "i13011", "i13012", "i13013" {
                        n2004 = global write "全局 提取仪器参数.vi" "参数编码"(w2426) -> ()
                        n2005 = call "数据处理直接插入整合 (子VI).vi"() -> ()  [unwired: 12 in]
                      }
                      frame "i12001", Default {
                        # "数据处理整合"
                        # "i12001状态"
                        n2006 = call "数据处理整合 (子VI).vi"("枚举"=enum16{"实时数据排序", "小时数据排序"}."实时数据排序") -> ("已排序的数组"=w2430:string[])  [unwired: 10 in]
                        n2007 = Array Size(array=w2430) -> (size(s)=w2429:i32)
                      }
                    }
                    n2008 = global write "全局 数据数组大小.vi" "数据数组大小"(w2413) -> ()
                    n2009 = local write "table元素"(w2414) -> ()
                  }
                }
              }
              frame "3021" {
                # "设置仪表参数"
                n2010 = local write "table元素"("反控命令" ("新元素/子数组")) -> ()
              }
              frame "3040" {
                # "提取现场系统信息（3040）"
                n2011 = flat-sequence {
                  tunnel: [T6."发送数据" ("元素")] -> w2436
                  frame #0 {
                    n2012 = local write "table元素"("提取现场系统信息" ("新元素/子数组")) -> ()
                  }
                  frame #1 {
                  }
                }
              }
              frame "3041" {
                # "提取现场经纬度及环境信息（3041）"
                n2013 = flat-sequence {
                  tunnel: [T6."发送数据" ("元素")] -> w2440
                  frame #0 {
                    n2014 = call "获取环境参数 (子VI).vi"() -> ()  [unwired: 12 in]
                    n2015 = local write "table元素"("提取经纬度环境信息" ("新元素/子数组")) -> ()
                  }
                  frame #1 {
                  }
                }
              }
              frame "3042" {
                # "发命令给中控"
                # "反控指令"
                # "0维护，1常规，2应急，3质控"
                # "反控指令\n切换运行模式"
                n2016 = local write "table元素"("反控命令" ("新元素/子数组")) -> ()
                n2017 = property on="数据" class="Str"() -> ("Value"=w2459:string)  [unwired: 2 in, 2 out]
                n2018 = Search/Split String(string=w2459, search string/char (-)="RunMode" ("搜索字符串/字符(-)")) -> (match + rest of string=w2457:string)  [unwired: 1 in, 2 out]
                n2019 = String Subset(string=w2457, offset (0)=8 ("偏移量(0)"), length (rest)=1 ("长度（剩余）")) -> (substring=w2454:string)
                n2020 = case shown="\"2\"" w2454 {
                  tunnel: [u16 0 ("新元素/子数组") u16 1 ("新元素/子数组") u16 2 ("新元素/子数组") u16 3 ("新元素/子数组")] -> w2448
                  frame "0", Default {
                  }
                  frame "1" {
                  }
                  frame "2" {
                  }
                  frame "3" {
                  }
                }
                n2021 = Insert Into Array(array=u16[] [] ("holding register values"), index=0 ("索引"), new element=w2448) -> (w2449:u16[])
                n2022 = call "Modbus Master.vi"("Unit ID"=u8 1, "读取写入选择"="写入", "holding register values"=w2449, "starting address"=u16 0) -> ()  [unwired: 6 in, 2 out]
              }
              frame "3043" {
                # "远程重启数采仪"
                n2023 = local write "table元素"("反控命令" ("新元素/子数组")) -> ()
              }
              frame "3044" {
                # "发回给平台"
                # "反控指令"
                # "3042~3086"
                # "反控指令\n单次测量"
                # "3044"
                n2024 = local write "table元素"("反控命令" ("新元素/子数组")) -> ()
                n2025 = flat-sequence {
                  frame #0 {
                    # "发命令给中控"
                    n2026 = call "Modbus Master.vi"("Unit ID"=u8 1, "读取写入选择"="写入", "holding register values"=u16[] [1], "starting address"=u16 2) -> ()  [unwired: 6 in, 2 out]
                  }
                  frame #1 {
                    n2027 = Wait (ms)(milliseconds to wait=u32 500 ("等待时间（毫秒）")) -> ()  [unwired: 1 out]
                  }
                  frame #2 {
                    n2028 = call "Modbus Master.vi"("Unit ID"=u8 1, "读取写入选择"="写入", "holding register values"=u16[] [0], "starting address"=u16 2) -> ()  [unwired: 6 in, 2 out]
                  }
                }
              }
              frame "3045", "3046" {
                # "发回给平台"
                # "反控指令"
                # "3042~3086"
                # "反控指令\n急停"
                # "3045"
                n2029 = flat-sequence {
                  frame #0 {
                    # "发命令给中控"
                    n2030 = call "Modbus Master.vi"("Unit ID"=u8 1, "读取写入选择"="写入", "holding register values"=u16[] [1], "starting address"=u16 3) -> ()  [unwired: 6 in, 2 out]
                  }
                  frame #1 {
                    n2031 = Wait (ms)(milliseconds to wait=u32 500 ("等待时间（毫秒）")) -> ()  [unwired: 1 out]
                  }
                  frame #2 {
                    n2032 = call "Modbus Master.vi"("Unit ID"=u8 1, "读取写入选择"="写入", "holding register values"=u16[] [0], "starting address"=u16 3) -> ()  [unwired: 6 in, 2 out]
                  }
                }
                n2033 = local write "table元素"("反控命令" ("新元素/子数组")) -> ()
              }
              frame "3056" {
                # "发命令给中控"
                # "设置测量时间间隔"
                # "发回给平台"
                n2034 = property on="数据" class="Str"() -> ("Value"=w2497:string)  [unwired: 2 in, 2 out]
                n2035 = local write "table元素"("反控命令" ("新元素/子数组")) -> ()
                n2036 = Search/Split String(string=w2497, search string/char (-)="RunInterval" ("搜索字符串/字符(-)")) -> (match + rest of string=w2498:string)  [unwired: 1 in, 2 out]
                n2037 = Decimal String To Number(string=w2498, offset=12 ("偏移量(0)")) -> (number=w2493:i32)  [unwired: 1 in, 1 out]
                n2038 = Insert Into Array(array=u16[] [] ("holding register values"), index=0 ("索引"), new element=w2493) -> (w2492:u16[])
                n2039 = call "Modbus Master.vi"("Unit ID"=u8 1, "读取写入选择"="写入", "holding register values"=w2492, "starting address"=u16 14) -> ()  [unwired: 6 in, 2 out]
              }
              frame "3080", "3081", "3082", "3083", "3084", "3085", "3086" {
                # "30 启动标液核查  1CODmn  2 氨氮  3总磷  4总氮  5CODCr\n31 加标回收\n32 平行样测试\n33 零点核查\n34 跨度核查\n35 校零\n36 校标"
                # "发回给平台"
                n2040 = flat-sequence {
                  tunnel: w2507 -> [w2513]
                  tunnel: [w2511] -> w2506
                  tunnel: w2506 -> [w2539]
                  tunnel: [w2539] -> w2505
                  tunnel: w2505 -> [w2542]
                  frame #0 {
                    # "1CODmn  2 氨氮  3总磷  4总氮  5CODCr"
                    # "启动单台仪器标液核查"
                    # "发命令给中控"
                    n2041 = property on="数据" class="Str"() -> ("Value"=w2523:string)  [unwired: 2 in, 2 out]
                    n2042 = Search/Split String(string=w2523, search string/char (-)="PolId" ("搜索字符串/字符(-)")) -> (match + rest of string=w2518:string)  [unwired: 1 in, 2 out]
                    n2043 = String Subset(string=w2518, offset (0)=6 ("偏移量(0)"), length (rest)=6 ("长度（剩余）")) -> (substring=w2515:string)
                    n2044 = case shown="\"w01019\"" w2515 {
                      tunnel: [0 ("长度（剩余）") 1 ("长度（剩余）") 2 ("长度（剩余）") 3 ("长度（剩余）") 4 ("长度（剩余）") 5 ("长度（剩余）")] -> w2514
                      frame "", Default {
                      }
                      frame "w01019" {
                      }
                      frame "w21003" {
                      }
                      frame "w21011" {
                      }
                      frame "w21001" {
                      }
                      frame "w01018" {
                      }
                    }
                    n2045 = Insert Into Array(array=u16[] [] ("holding register values"), index=0 ("索引"), new element=w2514) -> (w2519:u16[])
                    n2046 = case shown="\"3082\"" w2513 {
                      tunnel: [u16 99 ("starting address") u16 30 ("starting address") u16 31 ("starting address") u16 32 ("starting address") u16 33 ("starting address") u16 34 ("starting address") u16 35 ("starting address") u16 36 ("starting address")] -> w2511
                      frame "", Default {
                      }
                      frame "3080" {
                      }
                      frame "3081" {
                      }
                      frame "3082" {
                      }
                      frame "3083" {
                      }
                      frame "3084" {
                      }
                      frame "3085" {
                      }
                      frame "3086" {
                      }
                    }
                    n2047 = call "Modbus Master.vi"("Unit ID"=u8 1, "读取写入选择"="写入", "holding register values"=w2519, "starting address"=w2511) -> ()  [unwired: 6 in, 2 out]
                  }
                  frame #1 {
                    n2048 = Wait (ms)(milliseconds to wait=u32 500 ("等待时间（毫秒）")) -> ()  [unwired: 1 out]
                  }
                  frame #2 {
                    n2049 = call "Modbus Master.vi"("Unit ID"=u8 1, "读取写入选择"="写入", "holding register values"=u16[] [0], "starting address"=w2542) -> ()  [unwired: 6 in, 2 out]
                  }
                }
                n2050 = local write "table元素"("反控命令" ("新元素/子数组")) -> ()
              }
            }
            n2051 = Enqueue Element(queue=w2080, element=w2079, timeout in ms (-1)=1000 ("超时毫秒(-1)")) -> ()  [unwired: 1 in, 3 out]
          }
          frame "发送数据" {
            # "table输入，选择命令编码、发送哪些数据"
            n2052 = local read "table元素"() -> (w2549:string)
            n2053 = case shown="\"报警信息\", \"操作日志\", \"核查数据\", \"空白测试\", \"跨度核查\", \"零点核查\", \"实时数据\", \"提取集成干预\", \"提取加标回收\", \"提取平行样\", \"提取实时数据\", \"提取小时数据\", \"提取仪器参数\", \"仪器参数\"" w2549 {
              tunnel: w2548 -> [w2560 w2564 w2566 w2573]
              tunnel: [w2558 w2563 w2567 w2571] -> w2546
              tunnel: [w2559 w2562 w2568 w2572] -> w2547
              frame "", Default {
                n2054 = Increment(x=w2560) -> (x+1=w2559:i32)
                n2055 = global write "全局1.vi" "枚举"(w2560) -> ()
                n2056 = Greater Or Equal?(x=w2559, y=3) -> (x >= y?=w2558:bool)
              }
              frame "反控命令" {
                n2057 = Increment(x=w2564) -> (x+1=w2562:i32)
                n2058 = global write "全局 反控命令枚举.vi" "反控命令枚举"(w2564) -> ()
                n2059 = Greater Or Equal?(x=w2562, y=2) -> (x >= y?=w2563:bool)
              }
              frame "超标留样返回", "提取监测仪表时间", "提取经纬度环境信息", "提取现场系统信息" {
                n2060 = Increment(x=w2566) -> (x+1=w2568:i32)
                n2061 = global write "全局1.vi" "枚举"(w2566) -> ()
                n2062 = Greater Or Equal?(x=w2568, y=3) -> (x >= y?=w2567:bool)
              }
              frame "报警信息", "操作日志", "核查数据", "空白测试", "跨度核查", "零点核查", "实时数据", "提取集成干预", "提取加标回收", "提取平行样", "提取实时数据", "提取小时数据", "提取仪器参数", "仪器参数" {
                n2063 = global read "全局 小时数据发送次数.vi" "小时数据发送次数"() -> (w2575:i32)
                n2064 = global read "全局 数据数组大小.vi" "数据数组大小"() -> (w2570:i32)
                n2065 = Greater Or Equal?(x=w2575, y=w2570) -> (x >= y?=w2576:bool)
                n2066 = case shown="真" w2576 {
                  tunnel: w2573 -> [w2581 w2588]
                  tunnel: [w2581 w2582] -> w2577
                  frame False {
                  }
                  frame True {
                    n2067 = global read "全局 小时数据发送次数.vi" "小时数据发送次数"() -> (w2587:i32)
                    n2068 = global read "全局 数据数组大小.vi" "数据数组大小"() -> (w2584:i32)
                    n2069 = Equal To 0?(x=w2584) -> (x = 0?=w2585:bool)
                    n2070 = Equal To 0?(x=w2587) -> (x = 0?=w2586:bool)
                    n2071 = And(x=w2586, y=w2585) -> (x .and. y?=w2583:bool)
                    n2072 = case shown="真" w2583 {
                      tunnel: w2588 -> [w2590 _]
                      tunnel: [w2589 0 ("索引")] -> w2582
                      frame False {
                        n2073 = Increment(x=w2590) -> (x+1=w2589:i32)
                      }
                      frame True {
                      }
                    }
                  }
                }
                n2074 = Equal To 0?(x=w2577) -> (x = 0?=w2578:bool)
                n2075 = global write "全局1.vi" "枚举"(w2577) -> ()
                n2076 = case shown="真" w2578 {
                  tunnel: w2577 -> [w2579 _]
                  tunnel: [w2579 1] -> w2572
                  frame False {
                  }
                  frame True {
                  }
                }
                n2077 = Greater Or Equal?(x=w2572, y=2) -> (x >= y?=w2571:bool)
              }
            }
            n2078 = case shown="假" w2546 {
              tunnel: w2547 -> [w2592 _]
              tunnel: [w2592 1 ("索引")] -> w2551
              frame False {
              }
              frame True {
              }
            }
            n2079 = flat-sequence {
              tunnel: "table元素" -> [w2603]
              tunnel: w2555 -> [w2602]
              tunnel: [w2598] -> w2554
              tunnel: [w2607] -> w2552
              tunnel: w2554 -> [w2607]
              tunnel: w2553 -> [w2606]
              tunnel: w2546 -> [w2605]
              frame #0 {
                # "数据记录"
                # "数据编码"
                n2080 = local read "QN"() -> (w2601:string)
                n2081 = local read "MN"() -> (w2595:string)
                n2082 = local read "PW"() -> (w2594:string)
                n2083 = call "数据编码.vi"("table输入"=w2603, "错误常量 2"=w2602, "QN"=w2601, "MN"=w2595, "PW"=w2594) -> ("错误常量"=w2600:errorcluster, "通讯包字符串"=w2599:string)  [unwired: 9 in]
                n2084 = local read "数据发送通道"() -> (w2597:enum16{"TCP", "VISA"})
                n2085 = call "数据记录.vi"("写入字段"=w2599) -> ("连接的字符串"=→"发送报文显示":string)  [unwired: 10 in]
                n2086 = call "VISATCP组合选择发送.vi"("数据发送通道"=w2597, "命令"="write", "error in (no error)"=w2600, "写入缓冲区"=w2599) -> ("错误输出"=w2598:errorcluster)  [unwired: 8 in, 3 out]
              }
              frame #1 {
                n2087 = case shown="真" w2605 {
                  tunnel: w2606 -> [w2608 w2620]
                  frame False {
                    n2088 = Enqueue Element(queue=w2608, element=T6."发送数据" ("元素")) -> ()  [unwired: 2 in, 3 out]
                  }
                  frame True {
                    n2089 = local read "TCP服务端掉线计数"() -> (w2615:i32)
                    n2090 = Obtain Queue(name (unnamed)="重发掉线数据" ("名称（未命名）"), element data type=T16."水样测试") -> (queue out=w2613:refnum<queue>, error out=w2614:errorcluster)  [unwired: 3 in, 1 out]
                    n2091 = Get Queue Status(queue=w2613, error in (no error)=w2614) -> (# elements in queue=w2617:i32)  [unwired: 1 in, 7 out]
                    n2092 = Not Equal To 0?(x=w2617) -> (x != 0?=w2618:bool)
                    n2093 = Greater Or Equal?(x=w2615, y=1) -> (x >= y?=w2619:bool)
                    n2094 = And(x=w2618, y=w2619) -> (x .and. y?=w2611:bool)
                    n2095 = case shown="真" w2611 {
                      tunnel: [T6."读取数据" ("元素") T6."表格比对" ("元素")] -> w2621
                      frame False {
                      }
                      frame True {
                      }
                    }
                    n2096 = Enqueue Element(queue=w2620, element=w2621) -> ()  [unwired: 2 in, 3 out]
                  }
                }
              }
            }
            "查询数据发送" <- TRUE
          }
          frame "数据处理" {
            n2097 = local write "空闲时间"(0.0 ("空闲时间")) -> ()
            n2098 = local read "心跳包"() -> (w2632:bool)
            n2099 = Equal?(x=w2630, y="实时数据") -> (x = y?=w2628:bool)
            n2100 = case shown="假" w2632 {
              tunnel: w2636 -> [w2639 _]
              tunnel: w2630 -> [w2638 _]
              frame False {
                n2101 = call "插入单条数据.vi"("table输入"=w2638, "插入数据"=w2639) -> ()  [unwired: 8 in, 2 out]
              }
              frame True {
              }
            }
            n2102 = Select(t=0, s=w2628, f=w2626) -> (s? t:f=w2627:i32)
            n2103 = Enqueue Element(queue=w2635, element=T6."表格比对" ("元素"), timeout in ms (-1)=1000 ("超时毫秒(-1)")) -> ()  [unwired: 1 in, 3 out]
          }
        }
      }
      frame Error {
        n2104 = Unbundle By Name(w2643) -> ("code"=w2642:i32)
        n2105 = case shown="63" w2642 {
          tunnel: w2643 -> [w2648 w2658 w2691 w2719]
          tunnel: [w2654 w2674 w2707 w2719] -> w2647
          tunnel: w2641 -> [w2655 w2669 w2702 w2716]
          frame 0, Default {
            n2106 = Flush Queue(queue=w2655) -> (queue out=w2653:refnum<queue>)  [unwired: 1 in, 2 out]
            n2107 = Enqueue Element(queue=w2653, element=T6."初始化" ("元素"), timeout in ms (-1)=1000 ("超时毫秒(-1)")) -> ()  [unwired: 1 in, 3 out]
            n2108 = local read "数据发送通道"() -> (w2650:enum16{"TCP", "VISA"})
            n2109 = call "VISATCP组合选择发送.vi"("数据发送通道"=w2650, "命令"="close", "error in (no error)"=w2648) -> ("错误输出"=w2649:errorcluster)  [unwired: 9 in, 3 out]
            n2110 = call <vilib>:"Clear Errors.vi"("error in (no error)"=w2649) -> ("error out"=w2654:errorcluster)  [unwired: 5 in, 1 out]
            n2111 = global write "全局 数据发送重叠.vi" "掉线指示灯"(TRUE ("掉线指示灯")) -> ()
          }
          frame 63 {
            # "TCP服务器端口掉线"
            n2112 = Flush Queue(queue=w2669) -> (queue out=w2670:refnum<queue>)  [unwired: 1 in, 2 out]
            n2113 = local read "查询数据发送"() -> (w2666:bool)
            n2114 = property on="TCP服务端掉线计数" class="DigNum (严格)"() -> ("Value"=w2665:i32)  [unwired: 2 in, 2 out]
            n2115 = call <vilib>:"Boolean Crossing PtByPt.vi"("direction"=enum16{"either", "false-true", "true-false"}."false-true", "input"=w2666) -> ("crossing"=w2667:bool)  [unwired: 1 in]
            n2116 = Less Or Equal?(x=w2665, y=1) -> (x <= y?=w2663:bool)
            n2117 = Enqueue Element(queue=w2670, element=T6."初始化" ("元素"), timeout in ms (-1)=1000 ("超时毫秒(-1)")) -> ()  [unwired: 1 in, 3 out]
            n2118 = case shown="真" w2667 {
              frame False {
              }
              frame True {
                n2119 = disable-structure shown="禁用" {
                  frame Disabled {
                    # "判定数据为空时不写入临时表格"
                    n2120 = call "每个元素都写入临时表格 (子VI).vi"("组合框"="小时数据存储") -> ()  [unwired: 10 in, 1 out]
                  }
                  frame Enabled {
                  }
                }
              }
            }
            n2121 = case shown="真" w2663 {
              frame False {
                n2122 = global write "全局 数据发送重叠.vi" "TCP掉线时间节点"("TCP掉线时间节点") -> ()
                n2123 = local write "TCP掉线时间节点"("TCP掉线时间节点") -> ()
              }
              frame True {
                n2124 = Get Date/Time In Seconds() -> (seconds since 1Jan1904=w2687:timestamp)
                n2125 = Format Date/Time String(time format string (%c)="%Y%m%d%H%M%S%3u" ("时间格式字符串(%c)"), seconds (now)=w2687) -> (date/time string=w2689:string)  [unwired: 1 in]
                n2126 = call "格式时间字符串.vi"("字符串"=w2689) -> ("连接的字符串"=w2677:string)  [unwired: 10 in]
                n2127 = local write "TCP掉线时间节点"(w2677) -> ()
                n2128 = call <vilib>:"Application Directory.vi"() -> ("Application Directory"=w2685:path)
                n2129 = Build Path(base path=w2685, name or relative path="data\\Set.ini" ("名称或相对路径")) -> (appended path=w2686:path)
                n2130 = call <vilib>:"Open Config Data.vi"("configuration file path"=w2686) -> ("error out"=w2682:errorcluster, "refnum"=w2683:T8)  [unwired: 8 in, 1 out]
                n2131 = call-poly <vilib>:"Write Key.vi"("section"="掉线时间存储", "error in (no error)"=w2682, "value"=w2677, "key"="掉线时间", "refnum"=w2683) -> ("error out"=w2680:errorcluster, "refnum out"=w2681:T8)  [unwired: 4 in, 1 out]
                n2132 = call <vilib>:"Close Config Data.vi"("error in (no error)"=w2680, "refnum"=w2681) -> ()  [unwired: 8 in, 2 out]
              }
            }
            n2133 = local read "数据发送通道"() -> (w2660:enum16{"TCP", "VISA"})
            n2134 = call "VISATCP组合选择发送.vi"("数据发送通道"=w2660, "命令"="close", "error in (no error)"=w2658) -> ("错误输出"=w2659:errorcluster)  [unwired: 9 in, 3 out]
            n2135 = call <vilib>:"Clear Errors.vi"("error in (no error)"=w2659) -> ("error out"=w2674:errorcluster)  [unwired: 5 in, 1 out]
            n2136 = global write "全局 数据发送重叠.vi" "掉线指示灯"(TRUE ("掉线指示灯")) -> ()
            n2137 = property on="TCP服务端掉线计数" class="DigNum (严格)"() -> ("Value"=w2673:i32)  [unwired: 2 in, 2 out]
            n2138 = Increment(x=w2673) -> (x+1=w2671:i32)
            n2139 = property on="TCP服务端掉线计数" class="DigNum (严格)"("Value"=w2671) -> ()  [unwired: 2 in, 2 out]
          }
          frame 54 {
            # "TCP服务器端口掉线"
            n2140 = local read "查询数据发送"() -> (w2699:bool)
            n2141 = Flush Queue(queue=w2702) -> (queue out=w2703:refnum<queue>)  [unwired: 1 in, 2 out]
            n2142 = property on="TCP服务端掉线计数" class="DigNum (严格)"() -> ("Value"=w2698:i32)  [unwired: 2 in, 2 out]
            n2143 = call <vilib>:"Boolean Crossing PtByPt.vi"("direction"=enum16{"either", "false-true", "true-false"}."false-true", "input"=w2699) -> ("crossing"=w2700:bool)  [unwired: 1 in]
            n2144 = Less Or Equal?(x=w2698, y=1) -> (x <= y?=w2696:bool)
            n2145 = Enqueue Element(queue=w2703, element=T6."初始化" ("元素"), timeout in ms (-1)=1000 ("超时毫秒(-1)")) -> ()  [unwired: 1 in, 3 out]
            n2146 = case shown="真" w2700 {
              frame False {
              }
              frame True {
                n2147 = disable-structure shown="禁用" {
                  frame Disabled {
                    # "判定数据为空时不写入临时表格"
                    n2148 = call "每个元素都写入临时表格 (子VI).vi"("组合框"="小时数据存储") -> ()  [unwired: 10 in, 1 out]
                  }
                  frame Enabled {
                  }
                }
              }
            }
            n2149 = case shown="真" w2696 {
              frame False {
                n2150 = local read "TCP掉线时间节点"() -> (w2709:string)
                n2151 = global write "全局 数据发送重叠.vi" "TCP掉线时间节点"(w2709) -> ()
                n2152 = local write "TCP掉线时间节点"(w2709) -> ()
              }
              frame True {
                n2153 = Get Date/Time In Seconds() -> (seconds since 1Jan1904=w2711:timestamp)
                n2154 = Format Date/Time String(time format string (%c)="%Y%m%d%H%M%S%3u" ("时间格式字符串(%c)"), seconds (now)=w2711) -> (date/time string=w2713:string)  [unwired: 1 in]
                n2155 = call "格式时间字符串.vi"("字符串"=w2713) -> ("连接的字符串"=w2710:string)  [unwired: 10 in]
                n2156 = local write "TCP掉线时间节点"(w2710) -> ()
              }
            }
            n2157 = local read "数据发送通道"() -> (w2693:enum16{"TCP", "VISA"})
            n2158 = property on="TCP服务端掉线计数" class="DigNum (严格)"() -> ("Value"=w2706:i32)  [unwired: 2 in, 2 out]
            n2159 = call "VISATCP组合选择发送.vi"("数据发送通道"=w2693, "命令"="close", "error in (no error)"=w2691) -> ("错误输出"=w2692:errorcluster)  [unwired: 9 in, 3 out]
            n2160 = Increment(x=w2706) -> (x+1=w2704:i32)
            n2161 = property on="TCP服务端掉线计数" class="DigNum (严格)"("Value"=w2704) -> ()  [unwired: 2 in, 2 out]
            n2162 = call <vilib>:"Clear Errors.vi"("error in (no error)"=w2692) -> ("error out"=w2707:errorcluster)  [unwired: 5 in, 1 out]
            n2163 = global write "全局 数据发送重叠.vi" "掉线指示灯"(TRUE ("掉线指示灯")) -> ()
          }
          frame 56 {
            n2164 = Flush Queue(queue=w2716) -> (queue out=w2717:refnum<queue>)  [unwired: 1 in, 2 out]
            n2165 = Enqueue Element(queue=w2717, element=T6."读取数据" ("元素"), timeout in ms (-1)=1000 ("超时毫秒(-1)")) -> ()  [unwired: 1 in, 3 out]
          }
        }
        n2166 = call <vilib>:"Clear Errors.vi"("error in (no error)"=w2647) -> ("error out"=w2646:errorcluster)  [unwired: 5 in, 1 out]
      }
    }
  }
  n2167 = register-events(error in=w17, w18) -> (reference out=w6:refnum<event-registration>, error out=w5:errorcluster)  [unwired: 1 in]
  n2168 = while {
    shift-right: [w2723] -> w9
    shift-left: w5 -> [w2722]
    shift-right: [w2724] -> w12
    shift-left: w7 -> [w2725]
    shift-right: [w2721] -> w11
    shift-left: w6 -> [w2726]
    tunnel: [w2720] -> _
    stop <- w2720 stop-if-true
    n2169 = case shown="无错误" w2722 {
      selector: w2722 -> [w2728 w2762]
      tunnel: w2726 -> [w2733 w2757]
      tunnel: w2725 -> [w2732 w2758]
      tunnel: [w2731 w2758] -> w2724
      tunnel: [w2730 w2760] -> w2723
      tunnel: [w2729 FALSE ("Discard?")] -> w2720
      tunnel: [w2727 w2757] -> w2721
      frame No Error {
        n2170 = event shown="[0] <Public:SelectedItemEvent>: 用户事件" {
          selector: w2733 -> [_ _ _]
          dyn-events: [_ _ _] -> w2727
          timeout: _ -> [_ _ _]
          tunnel: w2728 -> [w2736 w2746 w2755]
          tunnel: [w2736 w2746 w2754] -> w2730
          tunnel: [w2735 TRUE FALSE ("Discard?")] -> w2729
          tunnel: w2732 -> [w2734 w2744 w2756]
          tunnel: [w2734 w2744 w2753] -> w2731
          event User Event {
            # "5."
            n2171 = event-data() -> ("ItemTag"=w2737:string)  [unwired: 1 in]
            n2172 = case shown="\"EXIT线程一\"" w2737 {
              tunnel: [FALSE TRUE] -> w2735
              frame Default {
                n2173 = Current VI's Path() -> (path=w2738:path)
                n2174 = Open VI Reference(vi path=w2738) -> (vi reference=w2739:refnum<vi>)  [unwired: 5 in, 1 out]
                n2175 = invoke class="VI" method="FP.Open"(reference=w2739, "Activate"=TRUE ("激活？")) -> ()  [unwired: 3 in, 5 out]
              }
              frame "EXIT线程一" {
              }
            }
          }
          event "停止 2": Value Change {
            # "5."
            n2176 = event-data() -> ()  [unwired: 1 in, 2 out]
            n2177 = Stop(stop? (T)=TRUE ("可见")) -> ()
          }
          event Panel Close? {
            # "4."
            n2178 = event-data() -> ("VIRef"=w2749:refnum<vi>)  [unwired: 1 in, 3 out]
            n2179 = invoke class="VI" method="FP.Open"(reference=w2749, "State"=T15."Hidden" ("状态")) -> ()  [unwired: 3 in, 5 out]
            n2180 = call <vilib>:"ShowBalloonTip.vi"("Balloon Icon"=BalloonIcon."Information", "error in"=w2755, "Text"="欢迎使用平台发送系统", "NotifyIcon in"=w2756) -> ("error out"=w2754:errorcluster, "NotifyIcon out"=w2753:refnum<class "NotifyIcon.lvclass">)  [unwired: 6 in]
            n2181 = event-data("Discard?"=TRUE ("放弃？")) -> ()  [unwired: 1 in, 1 out]
          }
        }
      }
      frame Error {
        n2182 = call <vilib>:"Simple Error Handler.vi"("error in (no error)"=w2762) -> ("error out"=w2761:errorcluster)  [unwired: 4 in, 4 out]
        n2183 = call <vilib>:"Clear Errors.vi"("error in (no error)"=w2761) -> ("error out"=w2760:errorcluster)  [unwired: 5 in, 1 out]
      }
    }
  }
  n2184 = Unregister For Events(event registration refnum=w11, error in=w9) -> (error out=w8:errorcluster)
  n2185 = property class="App"() -> ("App.Kind"=w13:T14)  [unwired: 2 in, 2 out]
  n2186 = call <vilib>:"Destructor.vi"("error in"=w8, "NotifyIcon"=w12) -> ("error out"=w14:errorcluster)  [unwired: 9 in]
  n2187 = case shown="\"Development System\"" w13 {
    tunnel: w14 -> [_ _ _ _ _ _ _]
    frame "invalid app kind", Default {
    }
    frame "Development System" {
      n2188 = Stop(stop? (T)=TRUE ("可见")) -> ()
    }
    frame "Run Time System" {
      n2189 = Quit LabVIEW(quit? (T)=TRUE ("退出？(T)")) -> ()
    }
    frame "Student Edition" {
    }
    frame "Embedded LabVIEW" {
    }
    frame "Evaluation" {
    }
    frame "Custom" {
    }
  }
  n2190 = call <vilib>:"Simple Error Handler.vi"("error in (no error)"=w14) -> ("error out"=→"error out":errorcluster)  [unwired: 4 in, 4 out]
